vi "myRIO_BRig_RT_v0,84.vi"() -> ()   [LabVIEW 2014]
uses:
  myRIO_BRig_RT__Case_Exp_stateList.ctl
  myRIO_BRig_RT__Case_NonExp_stateList.ctl
  <vilib>/Platform/TimedLoop/XDataNode/timing_clust.ctl
  <vilib>/Platform/TimedLoop/XDataNode/nitl_modes.ctl
  <vilib>/Platform/TimedLoop/XDataNode/wakeup.ctl
  <vilib>/WebDAVClient/Advanced/SessionHandle.ctl
  <vilib>/myRIO/Common/Instrument Driver Framework/myRIO v1.0/UART/vis/myRIO v1.0 Close UART.vi
  <vilib>/FPGAPlugInAG/myRIO-1900/niLvFpga_Open_myRIO-1900.vi
  <vilib>/rvi/interface/common/dynamic/niFpgaDynamicAddResources.vi
  <vilib>/Utility/error.llb/Error Cluster From Error Code.vi
  <vilib>/rvi/errors/niLvFpgaAdjustHostInterfaceError.vi
  <vilib>/FPGAPlugInAG/Dynamic/niLvFpga_Close_Dynamic.vi
  <vilib>/myRIO/Common/Instrument Driver Framework/Utilities/vis/FPGA Ref Manager.vi
  <vilib>/myRIO/Common/Instrument Driver Framework/myRIO v1.0/myRIO v1.0 Reset FPGA.vi
  <vilib>/myRIO/Common/Instrument Driver Framework/myRIO v1.0/IRQ/vis/myRIO v1.0 IRQ Info FGV.vi
  <vilib>/myRIO/Common/Instrument Driver Framework/myRIO v1.0/IRQ/vis/myRIO v1.0 Timer IRQ Info FGV.vi
  <vilib>/myRIO/Common/Instrument Driver Framework/myRIO v1.0/IRQ/vis/myRIO v1.0 ISR Agent.vi
  <vilib>/rvi/interface/nirviOpenFPGA/nirviOpenFPGA.xnode
  myRIO_BRig_FPGA_v3,81_build.lvbitx
  myRIO_BRig_FPGA_v3,81.vi
  <vilib>/rvi/interface/nirviReadWriteControl/nirviReadWriteControl.xnode
  <vilib>/Platform/TimedLoop/XDataNode/XDataNode.xnode
  <vilib>/rvi/interface/nirviCloseFPGA/nirviCloseFPGA.xnode
  <vilib>/Platform/TimedLoop/XDataNode/XDNodeRunTimeDep.lvlib
  <vilib>/rvi/interface/Simulation/niFpgaSimulationCallBeginRW.vi
  <vilib>/myRIO/Instrument Drivers/Utilities/Utilities.lvlib
  <vilib>/WebDAVClient/NI_WebDAV.lvlib
  NiFpgaLv.dll
panel:
  in  "Laser2_baseline":bool
  in  "Laser1_baseline":bool
  in  "CueLed_baseline":bool
  out "allReward_R":bool
  out "allReward_L":bool
  in  "I_allReward":bool caption="NonSpecific Lick Direction"
  in  "Tcycle_Reward_max_R":u16=1000 caption="Max" min=5 max=5000 step=5
  in  "Tcycle_Reward_min_R":u16=1000 caption="Min" min=5 max=5000 step=5
  in  "Tcycle_Reward_step_R":u16=1000 caption="Penalty" min=1 max=10000 step=1
  in  "Tcycle_Reward_max_L":u16=1000 caption="Max" min=5 max=5000 step=5
  in  "Tcycle_Reward_min_L":u16=1000 caption="Min" min=5 max=5000 step=5
  in  "Tcycle_Reward_step_L":u16=1000 caption="Penalty" min=1 max=10000 step=1
  in  "MTrig_CueLed":bool
  out "Threshold":bool
  out "tLoop":dbl
  in  "Tcycle_Cue_LED_max":u16=1000 caption="Max" min=5 max=5000 step=5
  in  "Tcycle_Cue_LED_min":u16=1000 caption="Min" min=5 max=5000 step=5
  in  "Tcycle_CuePenalty_LED":u16=1000 caption="Penalty" min=1 max=10000 step=1
  out "power_l2":dbl
  in  "MTrig_Laser_Switch":bool
  in  "Cue1Param_AudioLed_Count_NS":u16
  in  "Cue1Param_AudioLed_Count_Switch":u16
  in  "Cue1Param_AudioLed_Probability_NS":u16
  in  "Cue1Param_CueType_NS":u16(slide) max=2 step=1 scale=0.0..2.0
  in  "Cue1Param_AudioLed_Probability_Switch":u16
  in  "Cue1Param_CueType_Switch":u16(slide) max=2 step=1 scale=0.0..2.0
  in  "CueLed_Freq":dbl=10.0
  in  "CueLed_Tpeak":dbl=2.0
  in  "Laser_power_step_l2":dbl
  in  "Laser_power_max_l2":dbl
  in  "Laser_power_min_l2":dbl
  in  "Laser_Tshutter_l2":dbl=2.0
  in  "Laser_Freq_l2":dbl=10.0
  in  "Laser_Tpeak_l2":dbl=2.0
  in  "Laser_duration_l2":u16
  in  "LC_Sel_Count_NS_l2":u16
  in  "LC_Sel_Count_Switch_l2":u16
  in  "LC_Sel_Probability_NS_l2":u16
  in  "LC_Sel_Block_NS_l2":u16(slide) max=2 step=1 scale=0.0..2.0
  in  "LC_Sel_OnOff_NS_l2":bool
  in  "LC_Sel_Probability_Switch_l2":u16
  in  "LC_Sel_Block_Switch_l2":u16(slide) max=2 step=1 scale=0.0..2.0
  in  "LC_Sel_OnOff_Switch_l2":bool
  in  "LC_Sel_Tdelay_NS_l2":u16
  in  "LC_Sel_Tdelay_Switch_l2":u16
  in  "LC_Cue1_Count_NS_l2":u16
  in  "LC_Cue1_Count_Switch_l2":u16
  in  "LC_Cue1_delayOpt_NS_l2":bool
  in  "LC_ENL1_delayOpt_NS_l2":bool
  in  "LC_ENL1_Count_NS_l2":u16
  in  "LC_ENL1_Count_Switch_l2":u16
  in  "LC_Cue1_delayOpt_Switch_l2":bool
  in  "LC_ENL1_delayOpt_Switch_l2":bool
  in  "LC_Cue1_Probability_NS_l2":u16
  in  "LC_Cue1_Block_NS_l2":u16(slide) max=2 step=1 scale=0.0..2.0
  in  "LC_Cue1_OnOff_NS_l2":bool
  in  "LC_Cue1_Probability_Switch_l2":u16
  in  "LC_Cue1_Block_Switch_l2":u16(slide) max=2 step=1 scale=0.0..2.0
  in  "LC_Cue1_OnOff_Switch_l2":bool
  in  "LC_ENL1_Probability_NS_l2":u16 max=100 step=1
  in  "LC_ENL1_Block_NS_l2":u16(slide) max=2 step=1 scale=0.0..2.0
  in  "LC_ENL1_OnOff_NS_l2":bool
  in  "LC_ENL1_Probability_Switch_l2":u16 max=100 step=1
  in  "LC_ENL1_Block_Switch_l2":u16(slide) max=2 step=1 scale=0.0..2.0
  in  "LC_Cue1_Tdelay_NS_l2":u16
  in  "LC_ENL1_Tdelay_NS_l2":u16
  in  "LC_Cue1_Tdelay_Switch_l2":u16
  in  "LC_ENL1_Tdelay_Switch_l2":u16
  in  "LC_ENL1_OnOff_Switch_l2":bool
  in  "LC_Wrong_Probability_l2":u16
  in  "LC_Wrong_Trial_l2":u16(slide) max=2 step=1 scale=0.0..2.0
  in  "LC_Wrong_Block_l2":u16(slide) max=2 step=1 scale=0.0..2.0
  in  "LC_Wrong_OnOff_l2":bool
  in  "LC_Reward_Probability_l2":u16
  in  "LC_Reward_Trial_l2":u16(slide) max=2 step=1 scale=0.0..2.0
  in  "LC_Reward_Block_l2":u16(slide) max=2 step=1 scale=0.0..2.0
  in  "LC_Reward_OnOff_l2":bool
  in  "LC_Wrong_Tdelay_l2":u16
  in  "LC_Reward_Tdelay_l2":u16
  in  "LC_Sel_Count_NS_l1":u16
  in  "LC_Sel_Count_Switch_l1":u16
  in  "LC_Sel_Probability_NS_l1":u16
  in  "LC_Sel_Block_NS_l1":u16(slide) max=2 step=1 scale=0.0..2.0
  in  "LC_Sel_OnOff_NS_l1":bool
  in  "LC_Sel_Probability_Switch_l1":u16
  in  "LC_Sel_Block_Switch_l1":u16(slide) max=2 step=1 scale=0.0..2.0
  in  "LC_Sel_OnOff_Switch_l1":bool
  in  "LC_Sel_Tdelay_NS_l1":u16
  in  "LC_Sel_Tdelay_Switch_l1":u16
  out "I_connect_TCP":bool
  in  "get_countPerMS":bool
  in  "count_warmup_R_reset":bool
  in  "count_warmup_L_reset":bool
  out "count_warmup_R":u16
  out "count_warmup_L":u16
  out "SolenoidReward":bool
  in  "SolenoidProbability_L":u16=100 caption="Reward Time [ms]" min=1 max=1000 step=1
  in  "SolenoidProbability_R":u16=100 caption="Reward Time [ms]" min=1 max=1000 step=1
  out "power_l1":dbl caption="LaserPower"
  in  "Laser_power_step_l1":dbl
  in  "Laser_power_max_l1":dbl
  in  "Recording":bool
  in  "Laser_power_min_l1":dbl
  in  "FPGA_count2ms":dbl=159.0
  in  "Laser_Tshutter_l1":dbl=2.0
  in  "Laser_Freq_l1":dbl=10.0
  in  "Laser_Tpeak_l1":dbl=2.0
  in  "Laser_duration_l1":u16
  out "error out":errorcluster
  in  "LC_Cue1_Count_NS_l1":u16
  in  "LC_Cue1_Count_Switch_l1":u16
  in  "LC_Cue1_delayOpt_NS_l1":bool
  in  "LC_ENL1_delayOpt_NS_l1":bool
  in  "LC_ENL1_Count_NS_l1":u16
  in  "LC_ENL1_Count_Switch_l1":u16
  in  "LC_Cue1_delayOpt_Switch_l1":bool
  in  "LC_ENL1_delayOpt_Switch_l1":bool
  in  "Tcycle_Cue_Audio_max":u16=1000 caption="Max" min=5 max=5000 step=5
  in  "Tcycle_Cue_Audio_min":u16=1000 caption="Min" min=5 max=5000 step=5
  in  "SendData":bool
  out "cSpout":enum16{"Left", "Right"}(ring) caption="Left or Right Spout"
  out "A4":u32 caption="LickCounter_Right"
  out "A2":u32 caption="LickCounter_Left"
  in  "LR_wrong_Event":bool
  out "SelectWrong":bool
  out "SelectReward":bool
  in  "Left(F)_or_Right(T)":bool
  in  "ignoreWrong":bool
  in  "SelectionState":bool
  in  "LR_wrong_Laser":bool
  in  "LR_reward_Laser":bool
  in  "LR_reward_Event":bool
  out "nRewards_Right":u16 caption="# Rewards Total (Right)"
  out "nRewards_Left":u16 caption="# Rewards Total (Left)"
  out "nRewards_cur":u16 caption="# Rewards in Current Block"
  out "TpB_target":u16 caption="Target Trials Per Block"
  out "cState_NonExp":T1 caption="WarmUp State"
  out "iBlock":u16 caption="Current Block"
  out "cState":T2 caption="Experimental State"
  out "iTrial":u16 caption="Current Trial"
  in  "warmupType":u8(slide) max=2 step=1 scale=0.0..2.0
  in  "TestConnection":bool
  in  "warmup":bool caption="WarmUp"
  in  "Data Set Prefix":string="Exp1_TM2"
  out "Connected To Host?":bool
  in  "Host Password":string="sabalab"
  in  "Host UserName":string="Test2"
  in  "sp_RightSpout":u16(slide)=2 max=2 step=1 scale=0.0..2.0
  in  "sp_LeftSpout":u16(slide)=2 max=2 step=1 scale=0.0..2.0
  in  "BUR_max":u16 caption="Count Reward Structure  (0 = off)"
  in  "LC_Wrong_Probability_l1":u16
  in  "LC_Wrong_Trial_l1":u16(slide) max=2 step=1 scale=0.0..2.0
  in  "LC_Wrong_Block_l1":u16(slide) max=2 step=1 scale=0.0..2.0
  in  "LC_Wrong_OnOff_l1":bool
  in  "LC_Reward_Probability_l1":u16
  in  "LC_Reward_Trial_l1":u16(slide) max=2 step=1 scale=0.0..2.0
  in  "LC_Reward_Block_l1":u16(slide) max=2 step=1 scale=0.0..2.0
  in  "LC_Reward_OnOff_l1":bool
  in  "LC_Cue1_Probability_NS_l1":u16
  in  "LC_Cue1_Block_NS_l1":u16(slide) max=2 step=1 scale=0.0..2.0
  in  "LC_Cue1_OnOff_NS_l1":bool
  in  "LC_Cue1_Probability_Switch_l1":u16
  in  "LC_Cue1_Block_Switch_l1":u16(slide) max=2 step=1 scale=0.0..2.0
  in  "LC_Cue1_OnOff_Switch_l1":bool
  in  "LC_ENL1_Probability_NS_l1":u16 max=100 step=1
  in  "LC_ENL1_Block_NS_l1":u16(slide) max=2 step=1 scale=0.0..2.0
  in  "LC_ENL1_OnOff_NS_l1":bool
  in  "LC_ENL1_Probability_Switch_l1":u16 max=100 step=1
  in  "LC_ENL1_Block_Switch_l1":u16(slide) max=2 step=1 scale=0.0..2.0
  in  "Tcycle_Timeout":u16=1000 caption="Timeout Time [ms]" min=10 max=10000 step=1
  in  "Tcycle_Wrong":u16=1000 caption="Wrong Time [ms]" min=10 max=10000 step=1
  in  "Tcycle_Selection":u16=1000 caption="Answer Time [ms]" min=1 max=10000 step=1
  in  "Tcycle_RewardPost":u16=1000 caption="Consumption Time [ms]" min=250 max=10000 step=250
  in  "TpB_Max_R":u16=4 caption="Max TrialsPerBlock" min=1 max=12 step=1
  in  "TpB_Min_R":u16=4 caption="Min TrialsPerBlock" min=1 max=12 step=1
  in  "TpB_Max_L":u16=4 caption="Max TrialsPerBlock" min=1 max=12 step=1
  in  "TpB_Min_L":u16=4 caption="Min TrialsPerBlock" min=1 max=12 step=1
  in  "BUR_min":u16 caption="Count Reward Structure\n(0 = off)"
  in  "TrialUntilReward":bool caption="Ignore Wrong Selection"
  in  "CueCycles":u16=1 caption="Cue Structure" min=1 max=1 step=1
  in  "MTrig_Laser_Tcycle":u16=10 caption="Time [ms]"
  in  "MTrig_Laser_trig":bool
  in  "MTrig_Audio_trig__R":bool caption="Trigger Audio"
  in  "MTrig_Audio_trig__L":bool caption="Trigger Audio"
  in  "RewCalib_Trig_R":bool caption="Calibrate_R"
  in  "RewCalib_Trig_L":bool caption="Calibrate_L"
  in  "MTrig_Solenoid_Tcycle__R":u16=300 caption="Time [ms]"
  in  "MTrig_Solenoid_Tcycle__L":u16=300 caption="Time [ms]"
  in  "MTrig_Solenoid_trig__R":bool caption="Solenoid"
  in  "MTrig_Solenoid_trig__L":bool caption="Solenoid"
  in  "STOP_abort":bool caption="Stop LabView\n(Stops myRio and FPGA)"
  in  "STOP_endBlock":bool caption="Stop Experiment\n@ End of Block"
  in  "STOP_endTrial":bool caption="Stop Experiment\n@ End of Trial"
  in  "START":bool caption="Start Experiment"
  in  "Tcycle_CuePenalty_Audio":u16=1000 caption="Penalty" min=1 max=10000 step=1
  in  "Audio_Amp__R":u16=100 caption="Amp"
  in  "Audio_Freq__R":u8=5 caption="Freq [kHz]" max=14 step=1
  in  "Audio_Amp__L":u16=100 caption="Amp"
  in  "Audio_Freq__L":u8=5 caption="Freq [kHz]" max=14 step=1
  in  "LC_Wrong_Tdelay_l1":u16
  in  "LC_Cue1_Tdelay_NS_l1":u16
  in  "LC_ENL1_Tdelay_NS_l1":u16
  in  "LC_Reward_Tdelay_l1":u16
  in  "LC_Cue1_Tdelay_Switch_l1":u16
  in  "LC_ENL1_Tdelay_Switch_l1":u16
  in  "LC_ENL1_OnOff_Switch_l1":bool
  in  "Tcycle_ENLPenalty":u16=100 caption="Penalty" min=10 max=10000 step=10
  in  "Tcycle_ENL_max":u16=1000 caption="Max" min=250 max=10000 step=250
  in  "Tcycle_ENL_min":u16=1000 caption="Min" min=250 max=10000 step=250
  # "Communication (Host PC)"
  # "Recording Rig"
  # "Experimental Run"
  # "Experiment Task Structure"
  # "STOP experiment at"
  # "Min            Max            Penalty"
  # "(1) = Switching\n(2) = Two Choice"
  # "Enforced\nNonLick"
  # "FPGA Count per [ms]"
  # "Cue Audio"
  # "Current State"
  # "Cue LED"
  # "Global Parameters                                                         Trial Parameters"
  # "Selection"
  # "WarmUp"
  # "Reward - Dispense Water"
  # "Left/Right        Give Reward?        Laser Power [V]"
  # "Laser1      Laser2"
  # "Left"
  # "Cue then reward (no lick)\n \nLeft                    Right"
  # "Right"
  # "Min"
  # "Max"
  # "Dispense Water Probability"
  # "Block                   Trial            Target Trials       # Rewards \n                                                            Per Block             Current"
  # "Left"
  # "WarmUp State"
  # "Trial Per Block Structure \n               Left                        Right"
  # "Lick Counter"
  # "Right"
  # "Left           Right"
  # "Reward - Consumption"
  # "Manual Control"
  # "Min"
  # "# Rewards Total\n                                                                  Left                    Right"
  # "Experimental State"
  # "Penalty - Wrong Choice"
  # "Solenoid\n \nLeft              Right"
  # "Speaker\n \nLeft                    Right"
  # "Laser 1  |  Laser 2"
  # "Max"
  # "Penalty - Choice Timeout"
  # "Time\n[ms]"
  # "Time\n[ms]"
  # "Time = Cue Min"
  # "Cue LED"
  # "Power = Min"
  # "Cue1 Control\n                                  Cue Type           LED Probability [%]      Count"
  # "Laser1 Control\n                               On/Off      Block        Probability [%]   Delay [ms]                              Count"
  # "Laser2 Control\n                               On/Off      Block        Probability [%]   Delay [ms]                              Count"
  # "Audio or LED"
  # "Cue 1"
  # "Enforced\nNonLick\n      1"
  # "Enforced\nNonLick\n      1"
  # "from end"
  # "from end"
  # "Switch\nTrial"
  # "Switch\nTrial"
  # "Switch\nTrial"
  # "from start"
  # "from start"
  # "from end"
  # "from end"
  # "NonSwitch\nTrials"
  # "NonSwitch\nTrials"
  # "NonSwitch\nTrials"
  # "from start"
  # "from start"
  # "Cue 1"
  # "Cue 1"
  # "from end"
  # "from end"
  # "Switch\nTrial"
  # "Switch\nTrial"
  # "Cue Audio Parameters"
  # "Cue LED Parameters"
  # "from start"
  # "from start"
  # "Left                  Right"
  # "Frequency\n[Hz]"
  # "Frequency\n[kHz]"
  # "from end"
  # "from end"
  # "NonSwitch\nTrials"
  # "NonSwitch\nTrials"
  # "Timing [ms]\n                    Peak Width"
  # "from start"
  # "from start"
  # "Amp\n(0 - 32,000)"
  # "Selection"
  # "Selection"
  # "from start"
  # "from start"
  # "Switch\nTrial"
  # "Switch\nTrial"
  # "Speaker\nPattern\nDuring Cue"
  # "from start"
  # "from start"
  # "NonSwitch\nTrials"
  # "NonSwitch\nTrials"
  # "Laser1 Parameters"
  # "Laser2 Parameters"
  # "Laser1 Response\n                               On/Off      Block       Trial       Probability [%]   Delay [ms]"
  # "Laser2 Response\n                               On/Off      Block       Trial       Probability [%]   Delay [ms]"
  # "Frequency\n[Hz]"
  # "Frequency\n[Hz]"
  # "Timing [ms]\n Duration     Peak Width   Shutter"
  # "Timing [ms]\n Duration     Peak Width   Shutter"
  # "Selection Reward"
  # "Selection Reward"
  # "Laser Power [V]\nMin          Max              Step"
  # "Laser Power [V]\nMin          Max              Step"
  # "Selection Wrong"
  # "Selection Wrong"
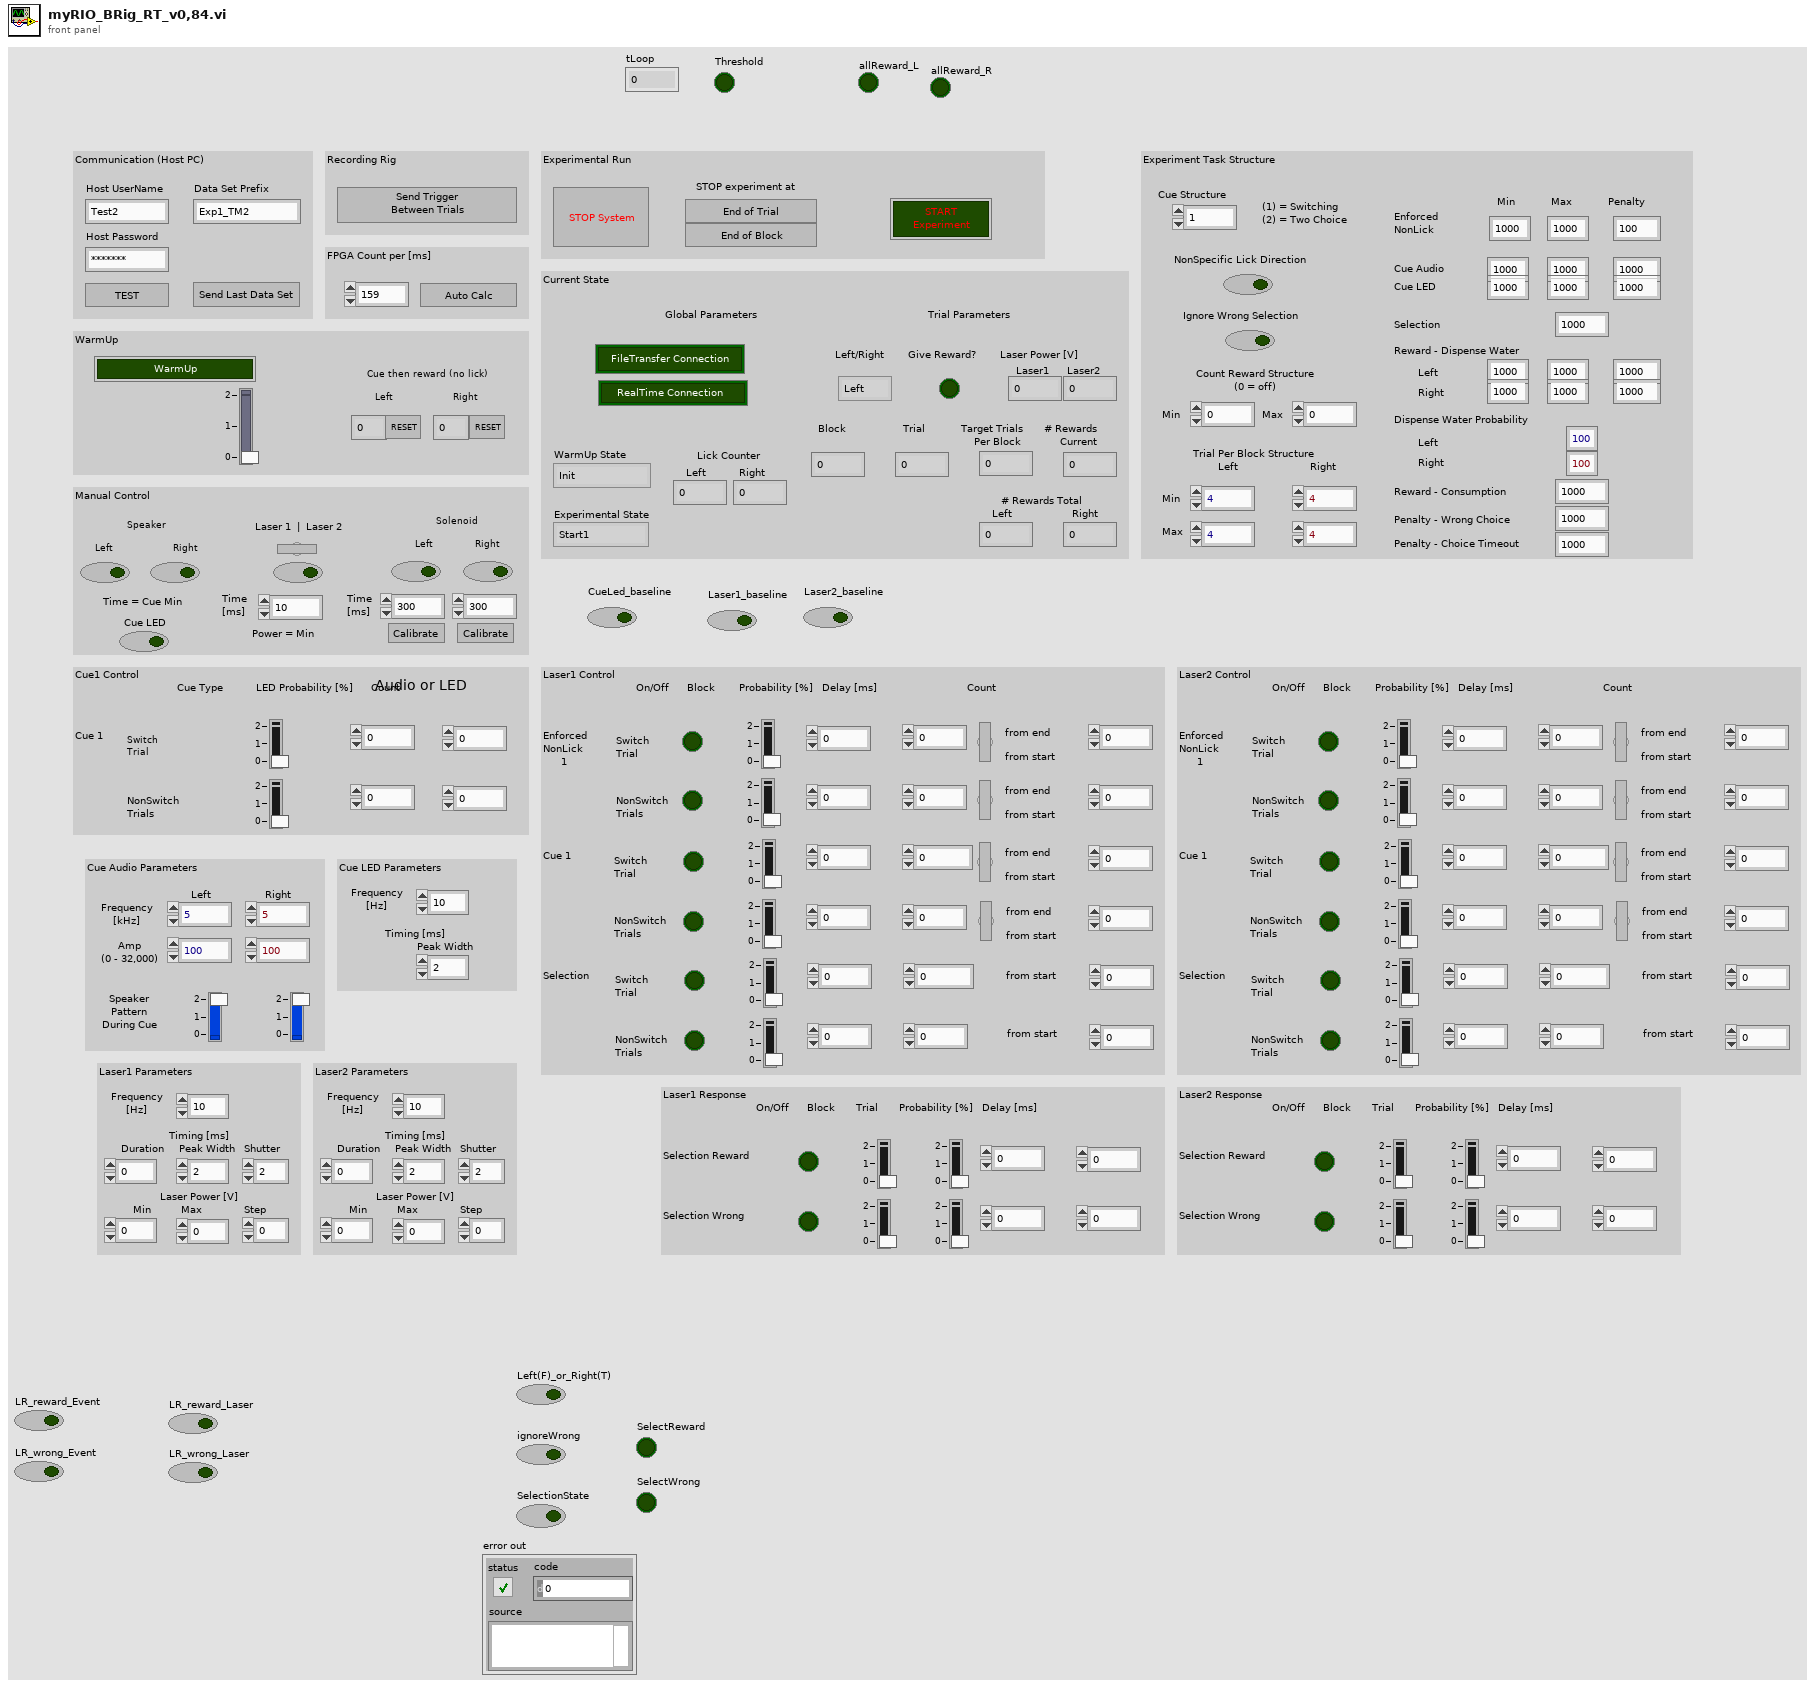
[diagram p1: front panel]
types:
  T1 = typedef "myRIO_BRig_RT__Case_NonExp_stateList.ctl" = enum16{"Init", "UploadSettings_pre", "UploadSettings_Read_dataExp", "UploadSettings_dataExp_1", "UploadSettings_dataExp_2", "UploadSettings_Read_dataLC", "UploadSettings_dataLC_1", "UploadSettings_dataLC_2", "UploadSettings_dataLC_3", "UploadSettings_dataLC_4", "UploadSettings_Read_dataMTrig", "UploadSettings_dataMTrig_1", "UploadSettings_post", "Idle_pre", "IdleEmpty", "IdleEmpty2", "IdleEmpty3", "IdleEmpty4", "Idle", "Idle_2", "Idle_3", "Idle_4", "Idle_5", "Idle_6", "Idle_post", "Cue_pre__pre", "Cue_pre", "Cue", "Cue_LED", "Cue_post", "RewardCalibration_pre", "DispenseWater_pre__pre", "DispenseWater_pre", "DispenseWater", "DispenseWater_post", "TestConnection", "SendData", "Get_FPGA_count_per_ms", "End"}
  T2 = typedef "myRIO_BRig_RT__Case_Exp_stateList.ctl" = enum16{"Start1", "Start2", "Start3", "saveSettings1", "saveSettings2", "saveSettings3", "saveSettings4", "saveSettings_LC_ENL_l1", "saveSettings_LC_ENL_l2", "saveSettings_LC_Cue_l1", "saveSettings_LC_Cue_l2", "saveSettings6_LC_l1_Other", "SaveSettings6_LC_l2_Other", "setSettings_Audio", "setSettings_Laser", "initBlock_pre", "initBlock", "initBlock2", "initBlock_post", "initTrial_pre", "initTrial", "initTrial2", "initTrial3", "initTrial4", "initTrial_LC_ENL1", "initTrial_LC_Cue1", "initTrial_LC_Cue1_2", "initTrial_LC_Sel", "initTrial_post", "ENL1_pre", "ENL1", "ENL1_post", "ENL1Penalty_pre", "ENL1Penalty", "ENL2_pre", "ENL2", "ENL2Penalty_pre", "ENL2Penalty", "Cue1_pre", "Cue1", "Cue1_post", "Cue1Penalty_pre", "Cue1Penalty", "Cue2_pre", "Cue2", "Cue2Penalty_pre", "Cue2Penalty", "Selection_pre", "Selection", "Select_post", "SelectReward_pre", "SelectReward", "SelectRewardPost_pre", "SelectRewardPost", "SelectWrong_pre", "SelectWrong", "SelectWrong_post", "SelectTimeout_pre", "SelectTimeout", "SelectTimeout_post", "endTrial_pre", "endTrial1", "endTrial2", "endTrial3", "endTrial_post", "endBlock_pre", "endBlock", "endBlock_post", "endExp", "commConnect", "commUpload_pre", "commUpload_dataBlock", "commUpload_dataCurrent", "commUpload_dataExp", "commUpload_dataLC", "commUpload_dataTrial", "commUpload_post", "saveData_pre", "saveData_dataBlock", "saveData_dataCurrent", "saveData_dataExp", "saveData_dataLC", "saveData_dataTrial", "saveData_post", "empty_endBlock1", "empty_endBlock2", "empty_endTrial1", "empty_endTrial2", "empty_endTrial3", "empty_endTrial4", "empty_endTrial5", "dummyState", "dummyState_endBlock"}
  T3 = typedef "XDNodeRunTimeDep.lvlib/timing_clust.ctl" = cluster{"Expected End [f-1]":u64, "Actual End [f-1]":u64, "Finished Late? [f-1]":bool, "Expected End [i-1]":u64, "Actual End [i-1]":u64, "Finished Late? [i-1]":bool, "Expected Start [i]":u64, "Actual Start [i]":u64, "Expected Start [f]":u64, "Actual Start [f]":u64, "Source Name":string, "Structure Name":string, "Period":i64, "Deadline":i64, "Offset":i64, "Start":i64, "Priority":i32, "Timeout":i32, "Mode":T4, "Wakeup Reason":T5, "Error":errorcluster, "Source Type":string, "Secondary Source Type":string, "Global End Time":u64, "Global Start Time":u64, "Frame Duration":u64, "Iteration Duration":u64, "Assigned CPU":i32, "I/O Scan Engine Mode":u32}
  T4 = typedef "XDNodeRunTimeDep.lvlib/nitl_modes.ctl" = enum32{"No Change", "Process missed periods, maintain original phase", "Discard missed periods, maintain original phase", "Process missed periods, ignore original phase", "Discard missed periods, ignore original phase"}
  T5 = typedef "XDNodeRunTimeDep.lvlib/wakeup.ctl" = enum32{"Normal", "Aborted", "Asynchronous wakeup", "Timing source error", "Timed loop error", "Timeout"}
  T6 = typedef "NI_WebDAV.lvlib/SessionHandle.ctl" = refnum<k1>
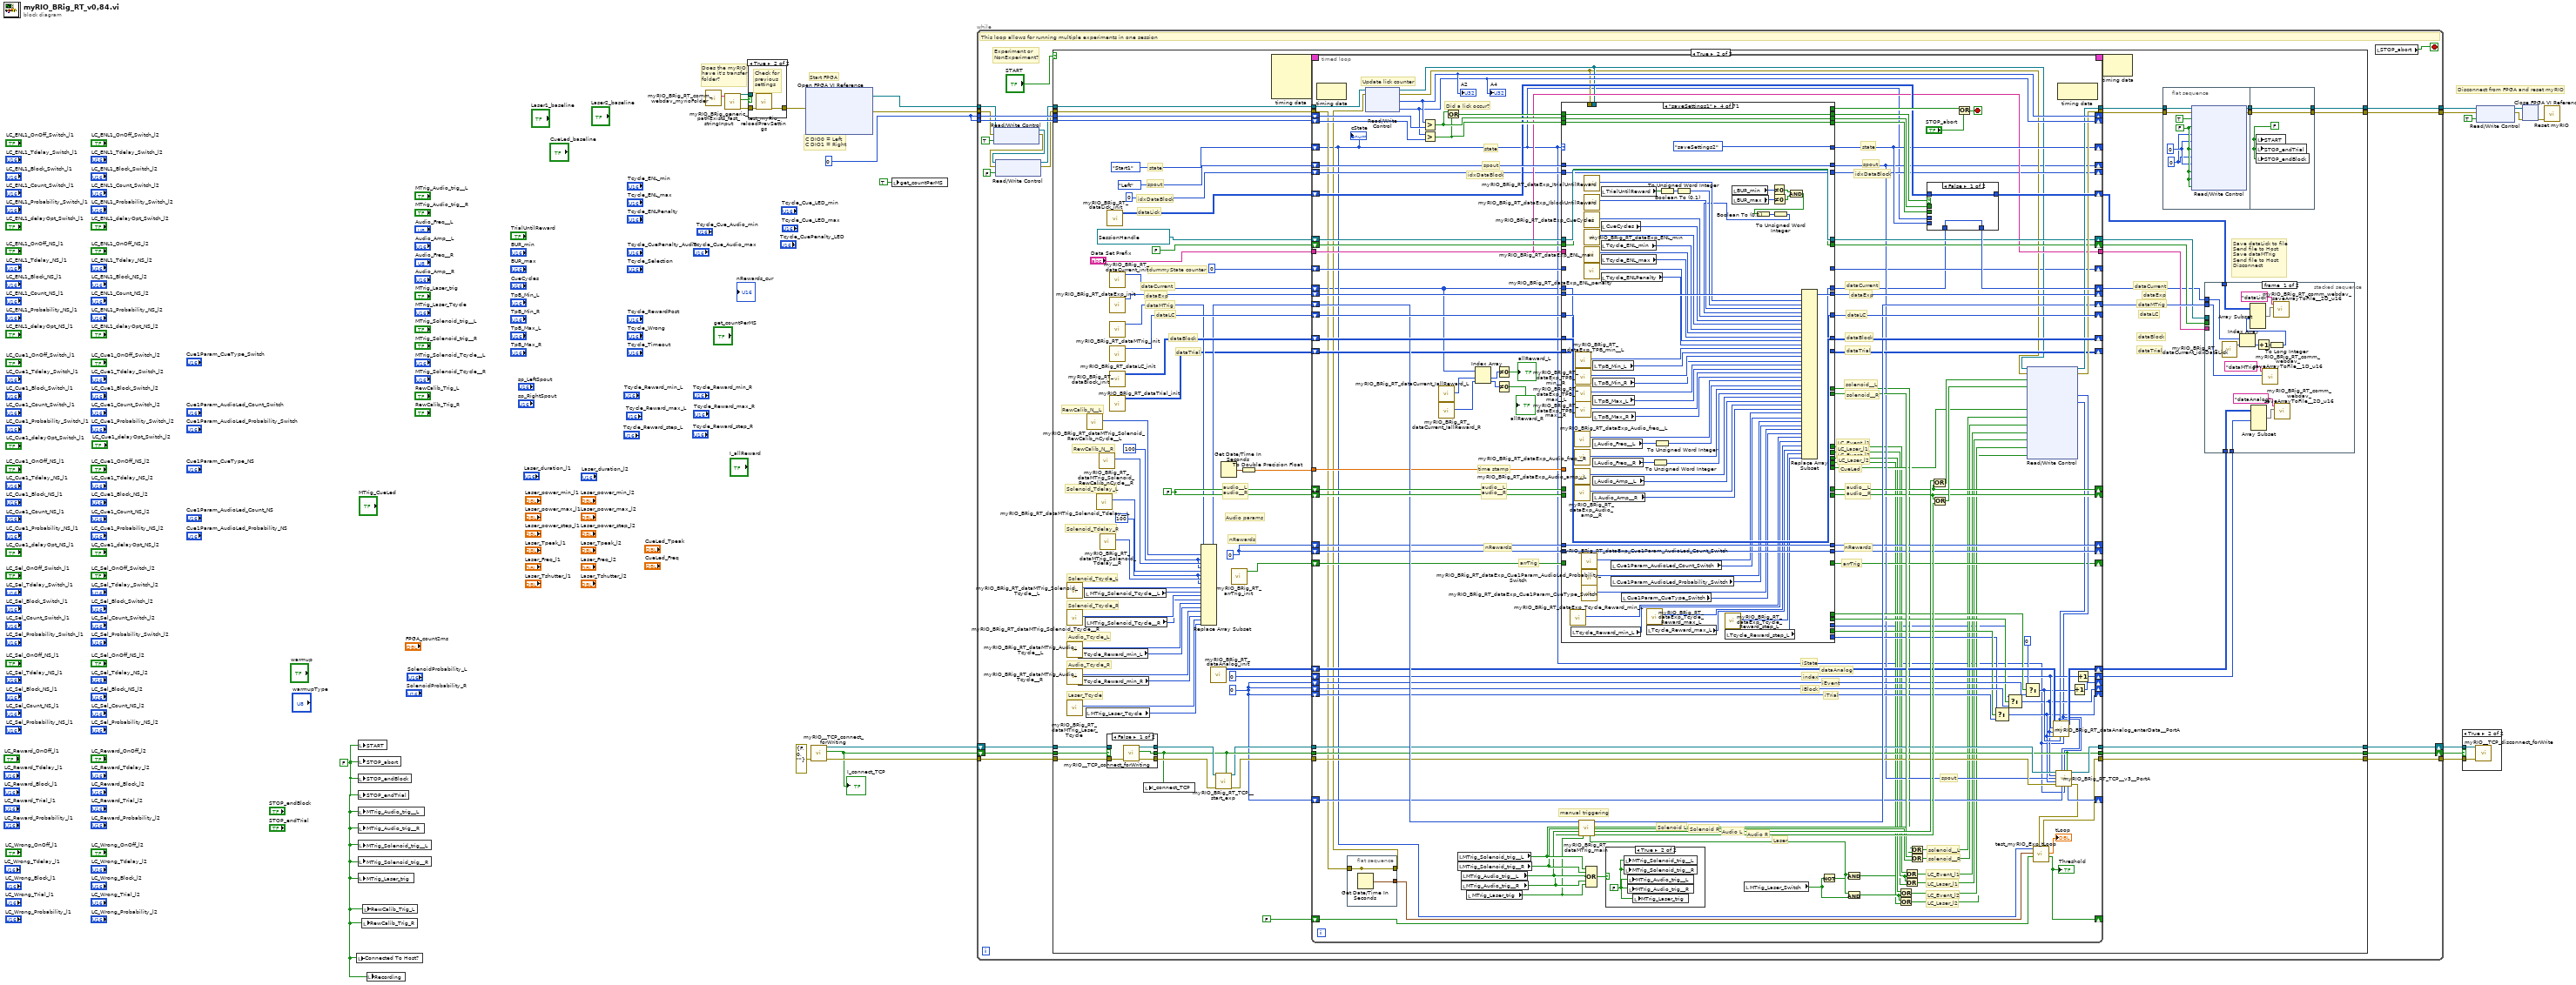
[diagram p0: block diagram]
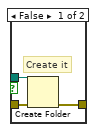
[diagram p3: hidden frame]
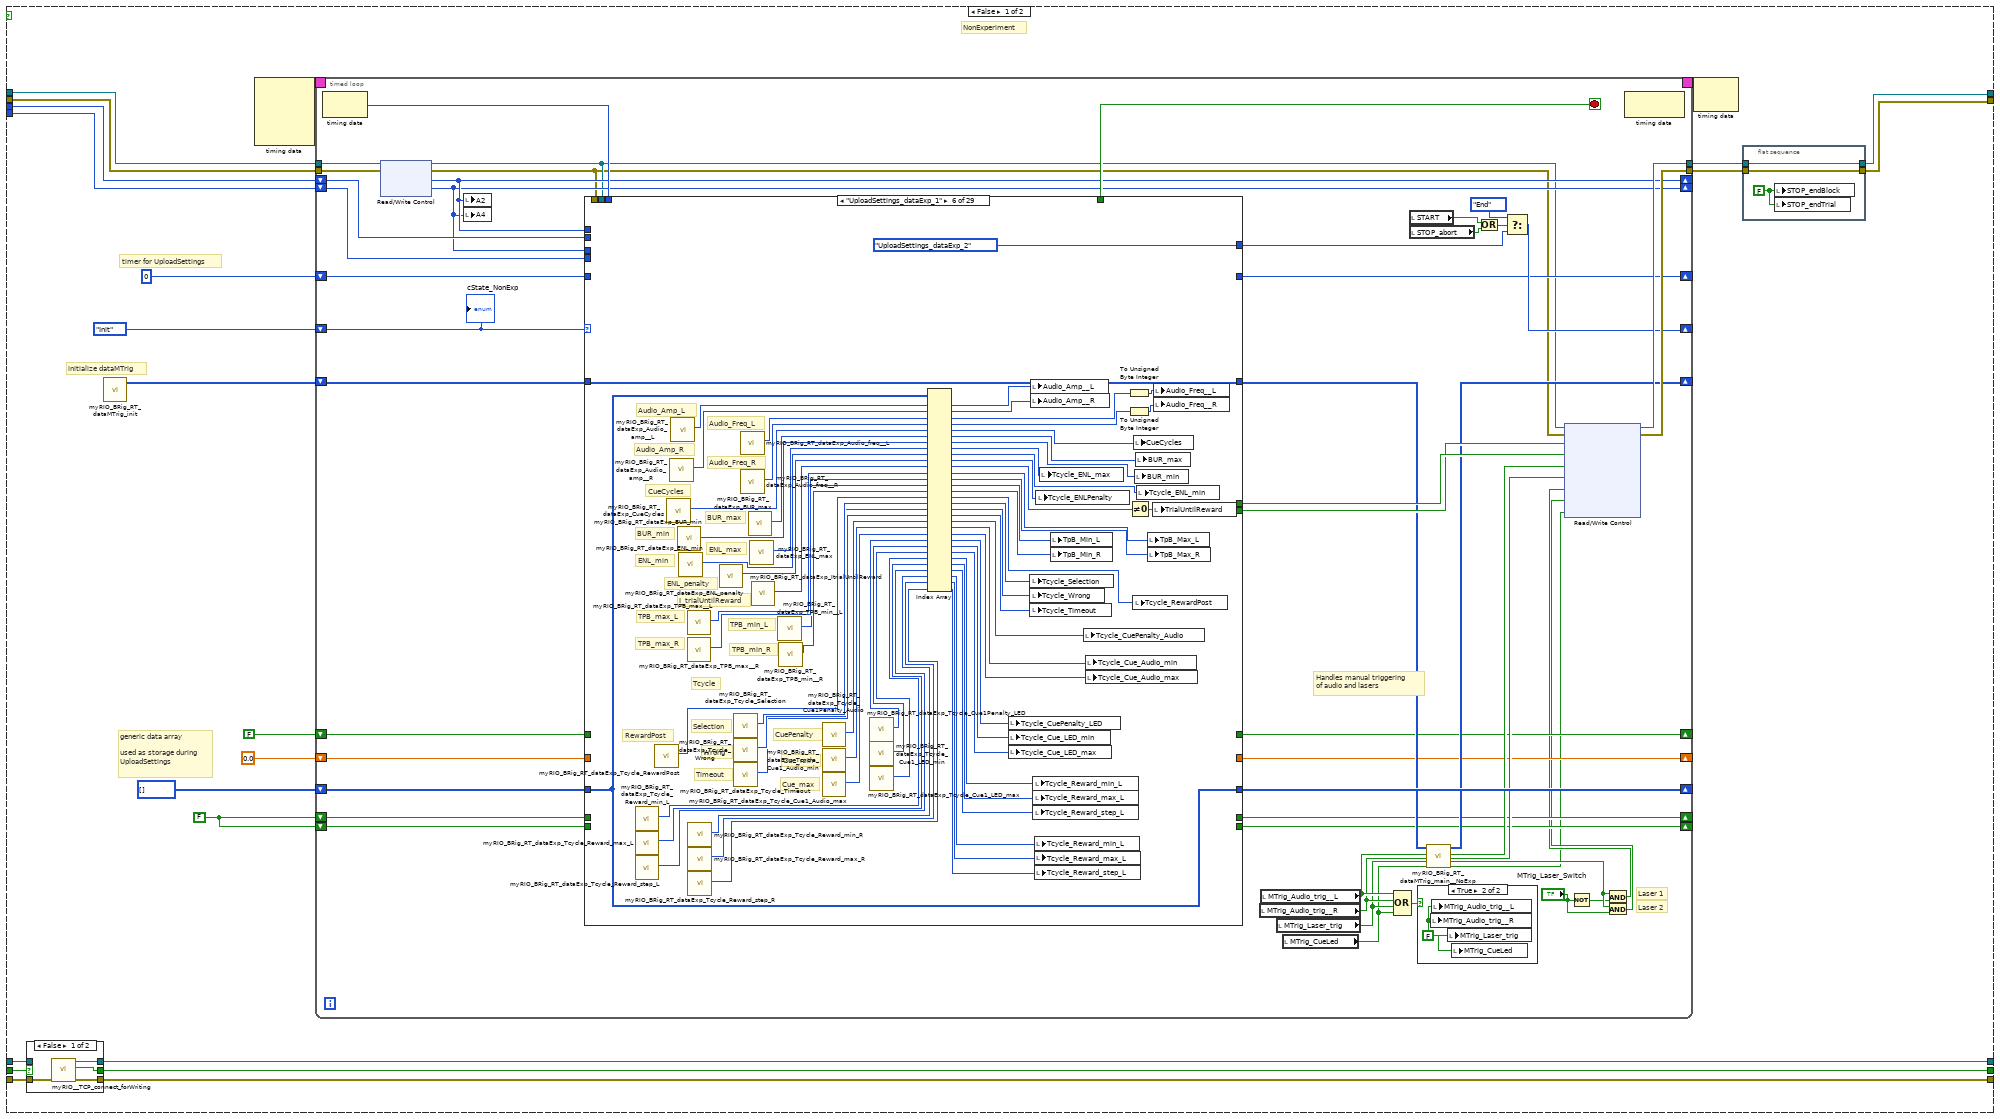
[diagram p4: hidden frame]
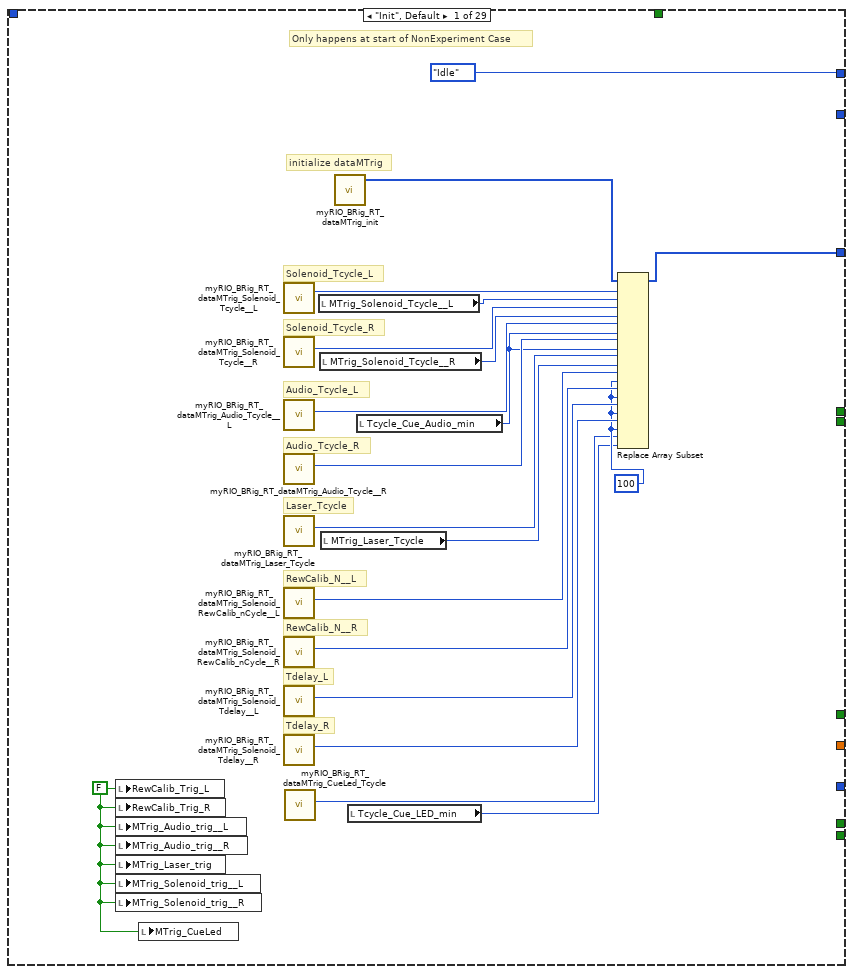
[diagram p7: hidden frame]
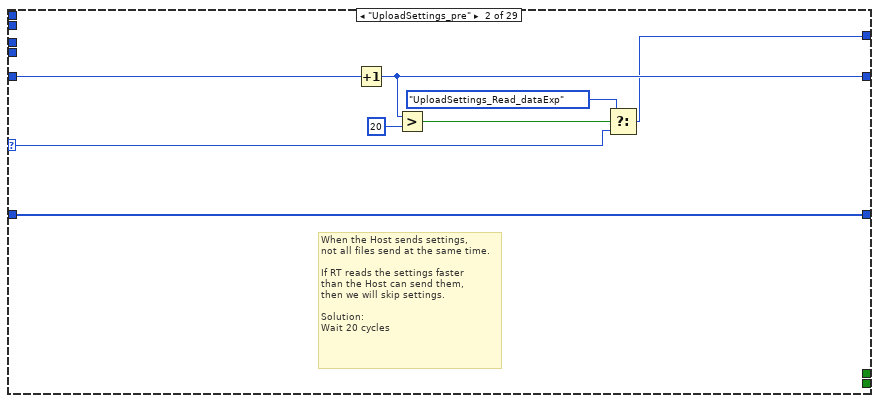
[diagram p8: hidden frame]
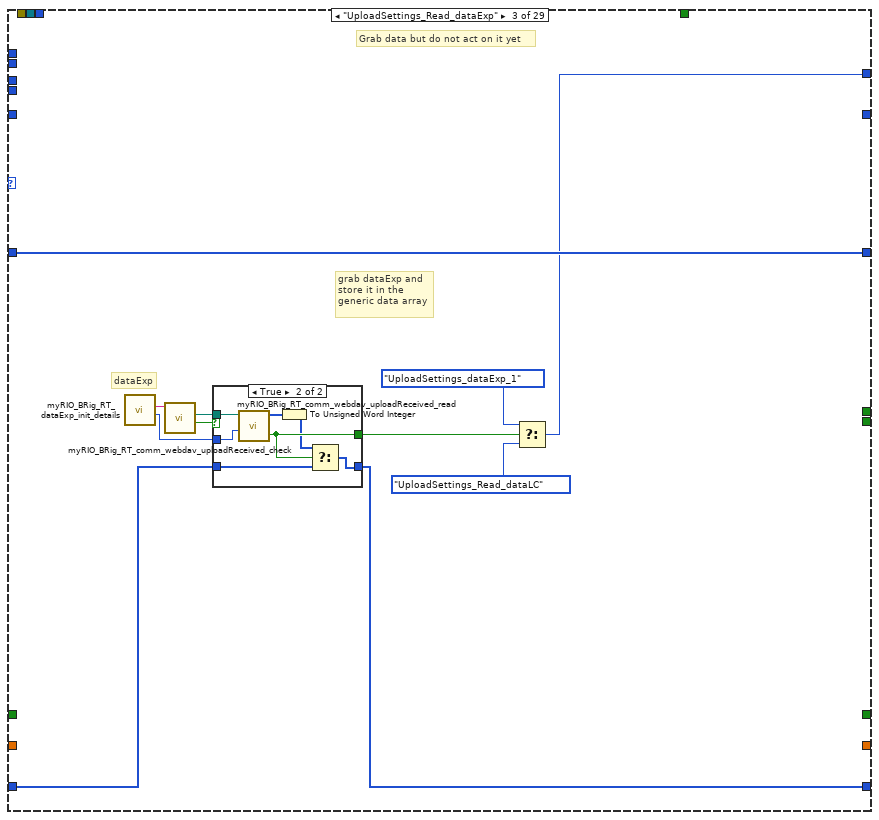
[diagram p9: hidden frame]
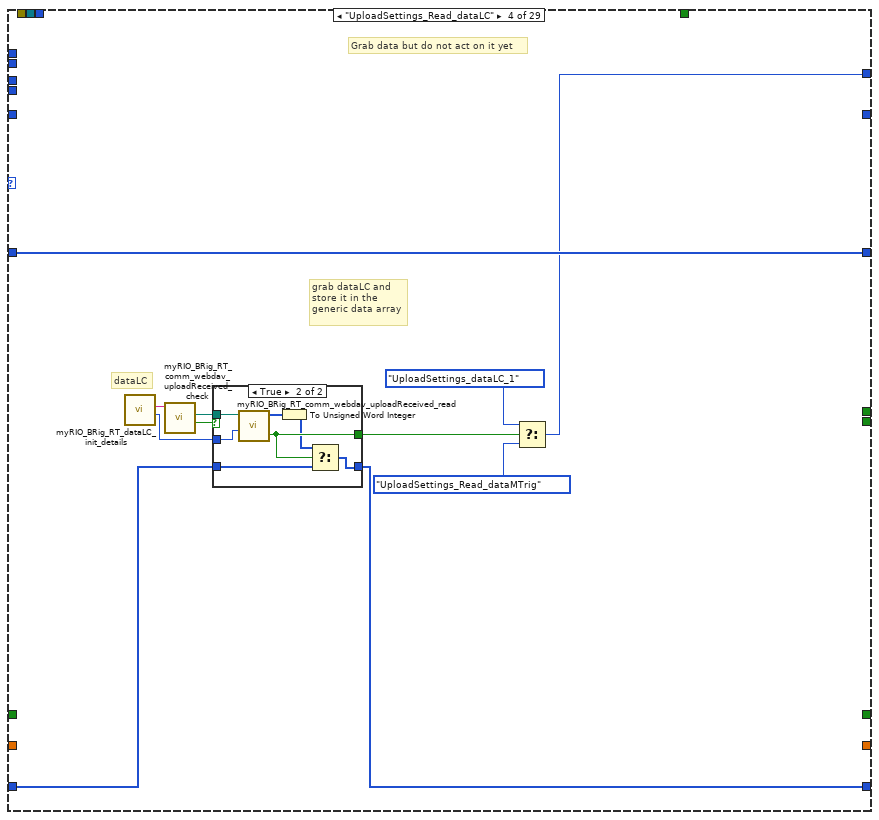
[diagram p11: hidden frame]
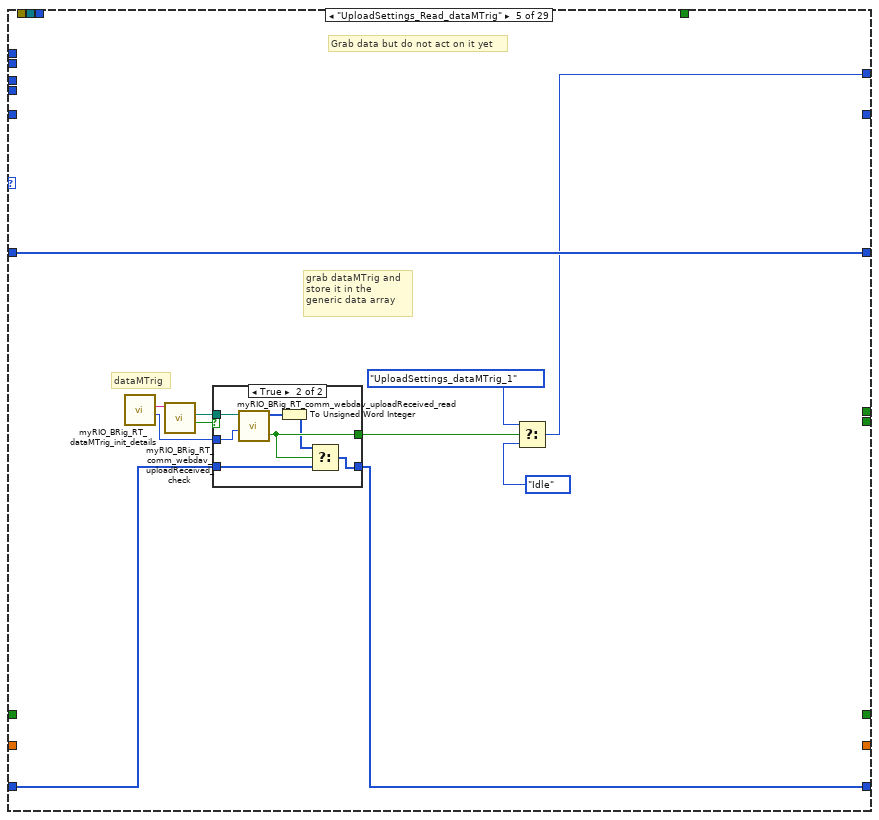
[diagram p13: hidden frame]
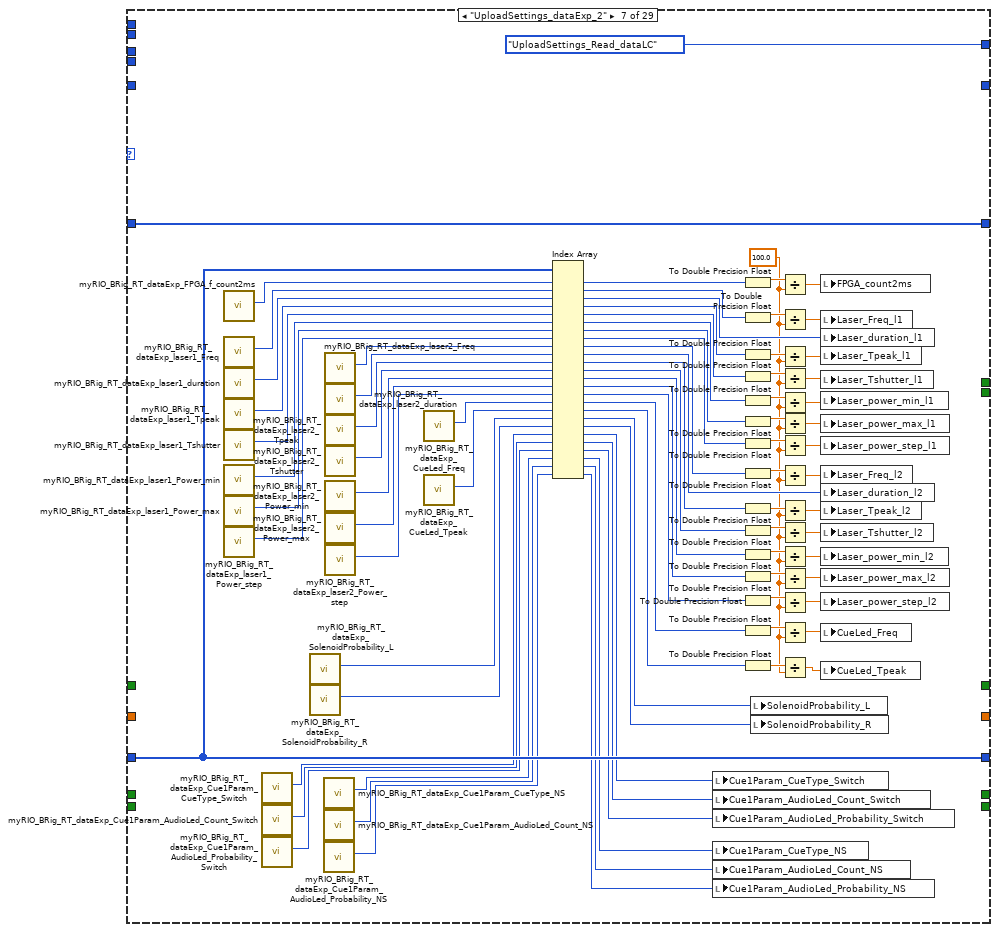
[diagram p15: hidden frame]
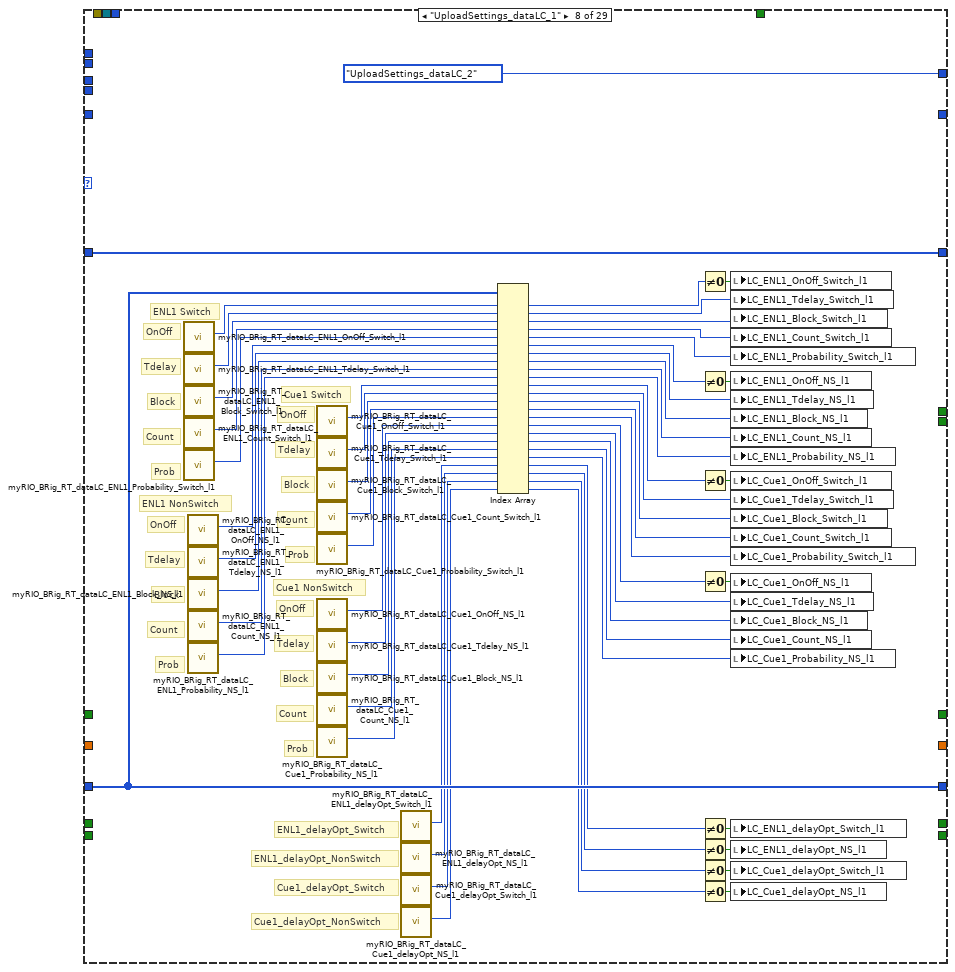
[diagram p16: hidden frame]
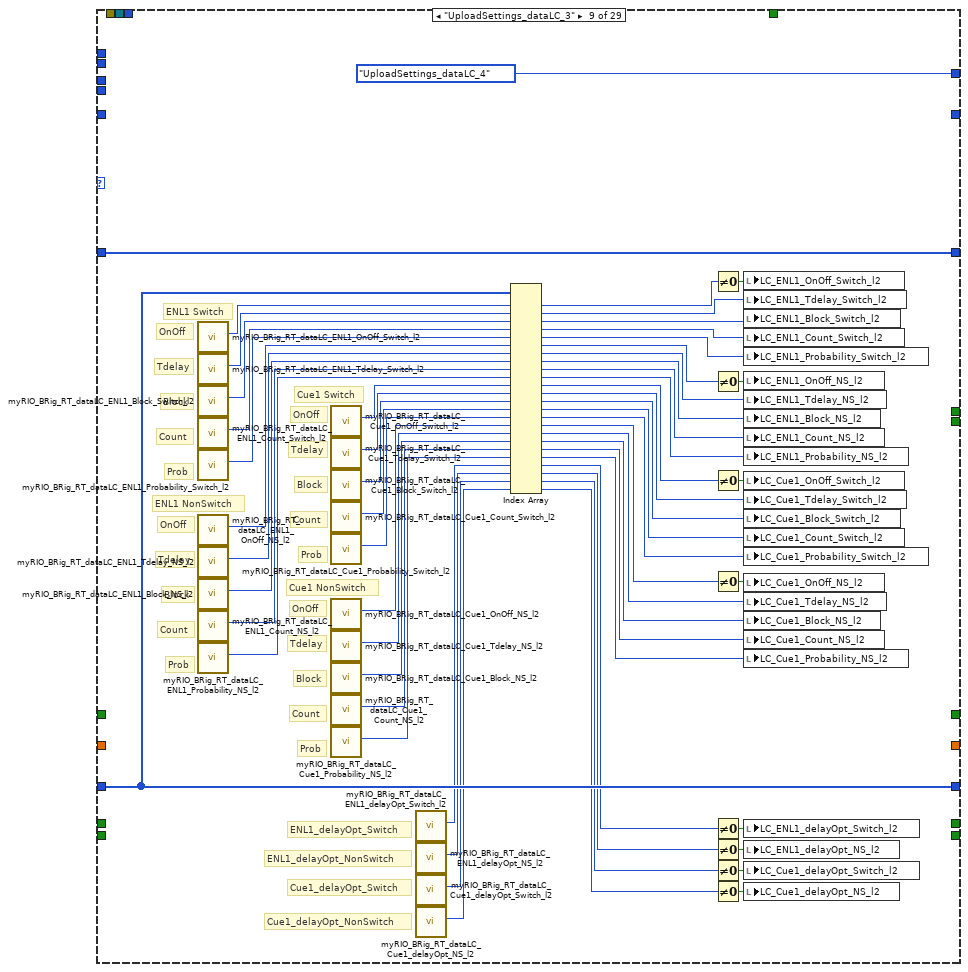
[diagram p17: hidden frame]
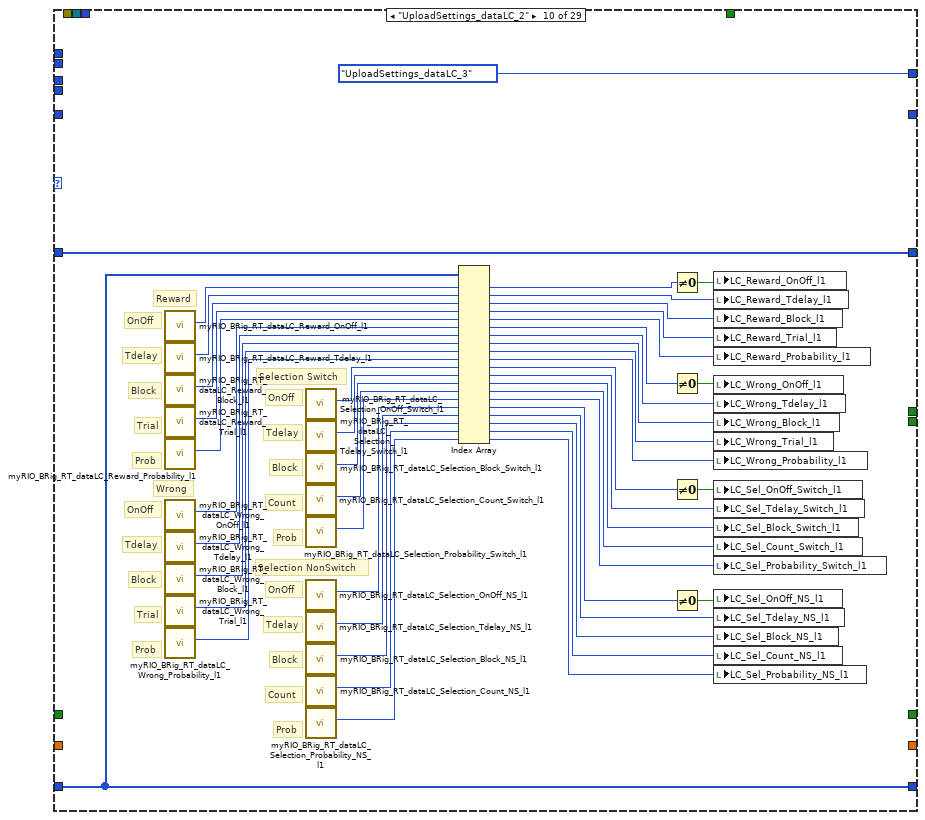
[diagram p18: hidden frame]
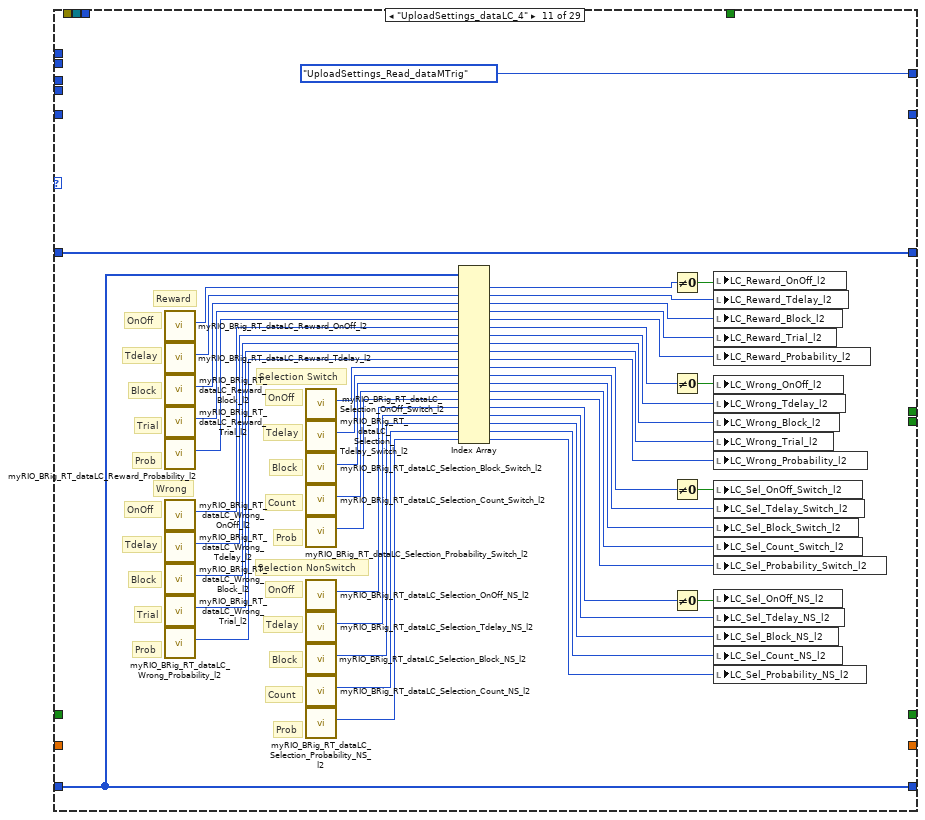
[diagram p19: hidden frame]
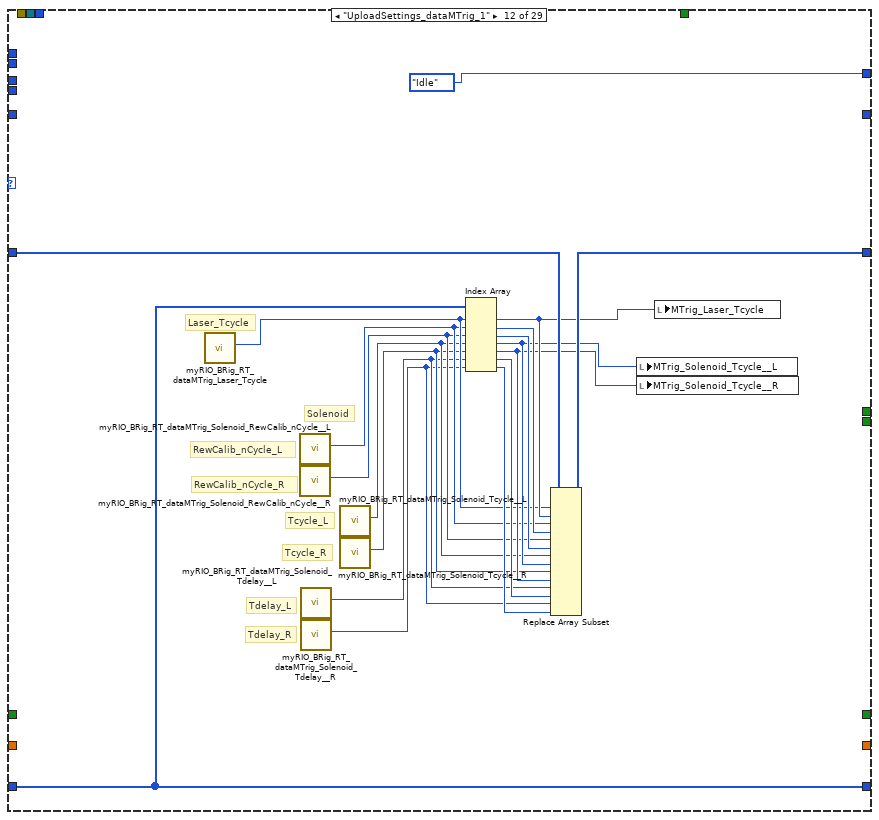
[diagram p20: hidden frame]
diagram:
  w17 = u32 0
  w1 = FALSE
  # "Does the myRIO\nhave it's transfer\nfolder?"
  # "C DIO0 = Left\nC DIO1 = Right"
  # "Start FPGA"
  # "Disconnect from FPGA and reset myRIO"
  n1 = local write "Connected To Host?"(w1) -> ()
  n2 = local write "START"(w1) -> ()
  n3 = local write "STOP_abort"(w1) -> ()
  n4 = local write "STOP_endBlock"(w1) -> ()
  n5 = local write "STOP_endTrial"(w1) -> ()
  n6 = local write "MTrig_Audio_trig__L"(w1) -> ()
  n7 = local write "MTrig_Audio_trig__R"(w1) -> ()
  n8 = local write "MTrig_Solenoid_trig__L"(w1) -> ()
  n9 = local write "MTrig_Solenoid_trig__R"(w1) -> ()
  n10 = local write "MTrig_Laser_trig"(w1) -> ()
  n11 = local write "RewCalib_Trig_R"(w1) -> ()
  n12 = local write "RewCalib_Trig_L"(w1) -> ()
  n13 = local write "Recording"(w1) -> ()
  n14 = call "myRIO_BRig_RT_comm_webdav_myrioFolder.vi"() -> ("output_myrioFolder"=w14:string)  [unwired: 11 in]
  n15 = call "myRIO_BRig_generic_pathExists_fast_stringInput.vi"("input_filePath"=w14) -> ("output_error"=w13:errorcluster, "output_Iexist"=w12:bool, "output_filePath"=w11:path)  [unwired: 8 in]
  n16 = case shown="True" w12 {
    tunnel: w11 -> [w26 _]
    tunnel: w13 -> [w25 w28]
    tunnel: [w24 w27] -> w9
    frame False {
      # "Create it"
      n17 = Create Folder(path (use dialog)=w26, error in=w25) -> (error out=w24:errorcluster)  [unwired: 1 in, 2 out]
    }
    frame True {
      # "Check for\nprevious\nsettings"
      n18 = call "test_myRio_reloadPrevSettings.vi"("input_error"=w28) -> ("output_error"=w27:errorcluster)  [unwired: 10 in]
    }
  }
  n19 = xnode "Open FPGA VI Reference"("error in"=w9) -> ("FPGA VI Reference Out"=w19:refnum<k20>, "error out"=w18:errorcluster)  [unwired: 1 in]
  n20 = call "myRIO__TCP_connect_forWriting.vi"("input_error"=errorcluster {"status"=FALSE, "code"=0, "source"=""}) -> ("output_error"=w7:errorcluster, "output_connected"=w6:bool, "output_hTCP"=w10:refnum<k5>)  [unwired: 8 in]
  "I_connect_TCP" <- w6
  n21 = local write "get_countPerMS"(TRUE ("get_countPerMS")) -> ()
  n22 = while {
    tunnel: w19 -> [w38]
    tunnel: w18 -> [w43]
    tunnel: w17 -> [w46]
    tunnel: w17 -> [w45]
    tunnel: [w36] -> w16
    tunnel: [w35] -> w15
    shift-right: [w32] -> w5
    shift-left: w6 -> [w33]
    tunnel: w7 -> [w31]
    shift-right: [w30] -> w4
    shift-left: w10 -> [w34]
    tunnel: [w29] -> w3
    stop <- w44 stop-if-true
    # "Experiment or\nNonExperiment?"
    # "This loop allows for running multiple experiments in one session"
    n23 = xnode "Read/Write Control"("FPGA VI Reference In"=w38, "error in"=w43, "Counts_Reset"=TRUE) -> ("FPGA VI Reference Out"=w40:refnum<k20>, "error out"=w41:errorcluster)
    n24 = xnode "Read/Write Control"("FPGA VI Reference In"=w40, "error in"=w41, "Counts_Reset"=FALSE) -> ("FPGA VI Reference Out"=w37:refnum<k20>, "error out"=w39:errorcluster)
    n25 = case shown="True" "START" {
      tunnel: w46 -> [w67 w1525]
      tunnel: w45 -> [w66 w1524]
      tunnel: w39 -> [w64 w1459]
      tunnel: w37 -> [w65 w1460]
      tunnel: [w62 w1521] -> w36
      tunnel: [w60 w1516] -> w35
      tunnel: w34 -> [w53 w1470]
      tunnel: [w51 w1474] -> w30
      tunnel: w33 -> [w52 w1472]
      tunnel: [w50 w1473] -> w32
      tunnel: w31 -> [w54 w1471]
      tunnel: [w49 w1469] -> w29
      frame False {
        w57 = FALSE
        # "generic data array\n\nused as storage during\nUploadSettings"
        # "timer for UploadSettings"
        # "initialize dataMTrig"
        # "NonExperiment"
        n26 = case shown="False" w52 {
          selector: w52 -> [_ w76]
          tunnel: w54 -> [w73 w78]
          tunnel: [w74 w78] -> w49
          tunnel: w53 -> [_ w77]
          tunnel: [w75 w77] -> w51
          tunnel: [w72 w76] -> w50
          frame False {
            n27 = call "myRIO__TCP_connect_forWriting.vi"("input_error"=w73) -> ("output_error"=w74:errorcluster, "output_connected"=w72:bool, "output_hTCP"=w75:refnum<k5>)  [unwired: 8 in]
          }
          frame True {
          }
        }
        n28 = call "myRIO_BRig_RT_dataMTrig_init.vi"() -> ("output_dataMTrig"=w68:u16[])  [unwired: 5 in]
        n29 = node-c288() -> (w71:T3)  [unwired: 4 in]
        n30 = timed-loop {
          timing: w71 -> [_]
          timing-out: [_] -> w70
          shift-right: [w117] -> _
          shift-left: w68 -> [w129]
          shift-right: [w111] -> _
          shift-left: myRIO_BRig_RT__Case_NonExp_stateList."Init" ("Enum") -> [w123]
          shift-right: [w105] -> _
          shift-left: w67 -> [w106]
          shift-right: [w103] -> _
          shift-left: w66 -> [w104]
          tunnel: [w125] -> w63
          tunnel: [w124] -> w61
          tunnel: w64 -> [w127]
          tunnel: w65 -> [w126]
          shift-right: [w122] -> _
          shift-left: u16[] [] ("output_data") -> [w121]
          shift-right: [w107] -> _
          shift-left: u16 0 ("Audio_Amp__L") -> [w108]
          shift-right: [w100] -> _
          shift-left: w57 -> [w102]
          shift-right: [w99] -> _
          shift-left: w57 -> [w101]
          shift-right: [w95] -> _
          shift-left: FALSE -> [w96]
          shift-right: [w93] -> _
          shift-left: 0.0 -> [w94]
          stop <- w130 stop-if-true
          # "Laser 2"
          # "Laser 1"
          # "Handles manual triggering\nof audio and lasers"
          n31 = node-c288() -> (w128:i64)  [unwired: 1 in]
          n32 = xnode "Read/Write Control"("FPGA VI Reference In"=w126, "error in"=w127) -> ("FPGA VI Reference Out"=w98:refnum<k20>, "error out"=w97:errorcluster, "A2_LickL"=w105:u32, "A4_LickR"=w103:u32)
          n33 = local write "A2"(w105) -> ()
          n34 = local write "A4"(w103) -> ()
          n35 = case shown="\"UploadSettings_dataExp_1\"" w123 {
            selector: w123 -> [_ w155 _ _ _ _ _ _ _ _ _ _ _ _ _ _ _ _ _ w1074 w1133 _ _ w1338 _ _ _ w1411 w1452]
            tunnel: [myRIO_BRig_RT__Case_NonExp_stateList."Idle" ("Enum") w153 w160 w179 w198 myRIO_BRig_RT__Case_NonExp_stateList."UploadSettings_dataExp_2" ("Enum") myRIO_BRig_RT__Case_NonExp_stateList."UploadSettings_Read_dataLC" ("Enum") myRIO_BRig_RT__Case_NonExp_stateList."UploadSettings_dataLC_2" ("Enum") myRIO_BRig_RT__Case_NonExp_stateList."UploadSettings_dataLC_4" ("Enum") myRIO_BRig_RT__Case_NonExp_stateList."UploadSettings_dataLC_3" ("f") myRIO_BRig_RT__Case_NonExp_stateList."UploadSettings_Read_dataMTrig" ("f") myRIO_BRig_RT__Case_NonExp_stateList."Idle" ("Enum") w621 w657 myRIO_BRig_RT__Case_NonExp_stateList."Idle_5" ("Enum") w730 w848 w1010 w1041 w1069 w1128 myRIO_BRig_RT__Case_NonExp_stateList."DispenseWater_pre" ("Enum") w1284 w1336 w1358 myRIO_BRig_RT__Case_NonExp_stateList."Idle" ("Enum") myRIO_BRig_RT__Case_NonExp_stateList."Idle" ("Enum") w1410 w1452] -> w112
            tunnel: [w143 w152 w170 w189 w208 w284 w368 w421 w480 w533 w580 w596 w625 w672 w716 w735 w853 w1008 w1048 w1075 w1134 w1195 w1321 w1343 w1369 w1403 w1408 w1420 w1450] -> w118
            tunnel: [_ _ _ _ _ _ _ _ _ _ _ _ _ _ _ _ _ _ _ _ _ _ _ _ _ _ _ _ TRUE] -> w130
            tunnel: w129 -> [_ w152 w170 w189 w208 w284 w368 w421 w480 w533 w580 w597 w624 w672 w716 w736 w854 w1008 w1049 w1076 w1135 w1181 w1317 w1344 w1370 w1403 w1408 w1420 w1450]
            tunnel: w128 -> [_ _ _ _ _ _ _ _ _ _ _ _ _ _ _ _ _ _ _ _ _ _ _ w1348 _ _ _ _ _]
            tunnel: [_ _ w161 w180 w199 w249 w366 w422 w481 w529 w576 w581 _ _ _ _ _ _ w1037 _ w1122 _ _ _ _ _ _ _ _] -> w122
            tunnel: w121 -> [_ _ w162 w181 w200 w249 w366 w422 w481 w529 w576 w581 _ _ _ _ _ _ _ _ w1123 _ _ _ _ _ _ _ _]
            tunnel: [_ _ _ _ _ _ _ _ _ _ _ _ _ _ _ _ _ _ _ _ _ _ _ w1345 _ _ _ _ _] -> w120
            tunnel: [_ _ _ _ _ _ _ _ _ _ _ _ _ _ _ _ _ _ _ _ _ _ _ w1327 _ _ _ _ _] -> w119
            tunnel: w108 -> [_ w159 _ _ _ _ _ _ _ _ _ _ _ _ _ _ _ _ _ _ _ _ _ _ _ _ _ _ _]
            tunnel: [_ w158 _ _ _ _ _ _ _ _ _ _ _ _ _ _ _ _ _ _ _ _ _ _ _ _ _ _ _] -> w107
            tunnel: w106 -> [_ _ _ _ _ _ _ _ _ _ _ _ _ _ _ _ _ _ _ w1080 w1139 _ _ _ _ _ _ _ _]
            tunnel: w105 -> [_ _ _ _ _ _ _ _ _ _ _ _ _ _ _ _ _ _ _ w1081 w1140 _ _ _ _ _ _ _ _]
            tunnel: w104 -> [_ _ _ _ _ _ _ _ _ _ _ _ _ _ _ _ _ _ _ w1078 w1137 _ _ _ _ _ _ _ _]
            tunnel: w103 -> [_ _ _ _ _ _ _ _ _ _ _ _ _ _ _ _ _ _ _ w1079 w1138 _ _ _ _ _ _ _ _]
            tunnel: w102 -> [_ _ _ _ _ _ _ _ _ _ _ _ _ _ _ _ _ _ _ w1066 w1125 _ _ _ _ _ _ _ _]
            tunnel: w101 -> [_ _ _ _ _ _ _ _ _ _ _ _ _ _ _ _ _ _ _ w1065 w1124 _ _ _ _ _ _ _ _]
            tunnel: [_ _ _ _ _ _ _ _ _ _ _ _ _ _ _ _ _ _ w1039 w1066 w1125 _ _ _ _ _ _ _ _] -> w100
            tunnel: [_ _ _ _ _ _ _ _ _ _ _ _ _ _ _ _ _ _ w1038 w1065 w1124 _ _ _ _ _ _ _ _] -> w99
            tunnel: w98 -> [_ _ _ _ _ _ _ _ _ _ _ _ w614 w630 w718 _ _ _ _ _ w1121 _ _ _ _ _ _ w1415 _]
            tunnel: w97 -> [_ _ _ _ _ _ _ _ _ _ _ _ w613 w631 w717 _ _ _ _ _ w1120 _ _ _ _ _ _ w1414 _]
            tunnel: w96 -> [_ _ _ _ _ _ _ _ _ _ _ _ _ _ _ _ _ _ _ _ _ _ _ _ _ _ _ w1419 _]
            tunnel: [_ _ _ _ _ _ _ _ _ _ _ _ _ _ _ _ _ _ _ _ _ _ _ _ _ _ _ TRUE _] -> w95
            tunnel: w94 -> [_ _ _ _ _ _ _ _ _ _ _ _ _ _ _ _ _ _ _ _ _ _ _ _ _ _ _ w1417 _]
            tunnel: [_ _ _ _ _ _ _ _ _ _ _ _ _ _ _ _ _ _ _ _ _ _ _ _ _ _ _ w1416 _] -> w93
            frame "Init", Default {
              w134 = FALSE ("RewCalib_Trig_L")
              w135 = u16 100 ("new element/subarray")
              # "Only happens at start of NonExperiment Case"
              # "Tdelay_R"
              # "Tdelay_L"
              # "RewCalib_N__R"
              # "RewCalib_N__L"
              # "Solenoid_Tcycle_R"
              # "Solenoid_Tcycle_L"
              # "Laser_Tcycle"
              # "Audio_Tcycle_R"
              # "Audio_Tcycle_L"
              # "initialize dataMTrig"
              n36 = local write "RewCalib_Trig_L"(w134) -> ()
              n37 = local write "RewCalib_Trig_R"(w134) -> ()
              n38 = local write "MTrig_Audio_trig__L"(w134) -> ()
              n39 = local write "MTrig_Audio_trig__R"(w134) -> ()
              n40 = local write "MTrig_Laser_trig"(w134) -> ()
              n41 = local write "MTrig_Solenoid_trig__L"(w134) -> ()
              n42 = local write "MTrig_Solenoid_trig__R"(w134) -> ()
              n43 = local write "MTrig_CueLed"(w134) -> ()
              n44 = call "myRIO_BRig_RT_dataMTrig_Solenoid_Tcycle__L.vi"() -> ("output_Solenoid_Tcycle__L"=w145:i32)  [unwired: 11 in]
              n45 = call "myRIO_BRig_RT_dataMTrig_Solenoid_Tcycle__R.vi"() -> ("output_Solenoid_Tcycle__R"=w146:i32)  [unwired: 11 in]
              n46 = call "myRIO_BRig_RT_dataMTrig_Audio_Tcycle__L.vi"() -> ("output_Audio_Tcycle__L"=w147:i32)  [unwired: 11 in]
              n47 = call "myRIO_BRig_RT_dataMTrig_Audio_Tcycle__R.vi"() -> ("output_Audio_Tcycle__R"=w148:i32)  [unwired: 11 in]
              n48 = call "myRIO_BRig_RT_dataMTrig_Laser_Tcycle.vi"() -> ("output_Laser_Tcycle"=w149:i32)  [unwired: 11 in]
              n49 = call "myRIO_BRig_RT_dataMTrig_Solenoid_RewCalib_nCycle__L.vi"() -> ("output_Solenoid_RewCalib_nCycle__L"=w141:i32)  [unwired: 11 in]
              n50 = call "myRIO_BRig_RT_dataMTrig_Solenoid_RewCalib_nCycle__R.vi"() -> ("output_Solenoid_RewCalib_nCycle__R"=w140:i32)  [unwired: 11 in]
              n51 = call "myRIO_BRig_RT_dataMTrig_Solenoid_Tdelay__L.vi"() -> ("output_Solenoid_Tdelay__L"=w139:i32)  [unwired: 11 in]
              n52 = call "myRIO_BRig_RT_dataMTrig_Solenoid_Tdelay__R.vi"() -> ("output_Solenoid_Tdelay__R"=w138:i32)  [unwired: 11 in]
              n53 = call "myRIO_BRig_RT_dataMTrig_CueLed_Tcycle.vi"() -> ("output_CueLed_Tcycle"=w133:i32)  [unwired: 11 in]
              n54 = local read "MTrig_Solenoid_Tcycle__L"() -> (w150:u16)
              n55 = local read "MTrig_Solenoid_Tcycle__R"() -> (w151:u16)
              n56 = local read "MTrig_Laser_Tcycle"() -> (w136:u16)
              n57 = call "myRIO_BRig_RT_dataMTrig_init.vi"() -> ("output_dataMTrig"=w144:u16[])  [unwired: 5 in]
              n58 = local read "Tcycle_Cue_LED_min"() -> (w132:u16)
              n59 = local read "Tcycle_Cue_Audio_min"() -> (w137:u16)
              n60 = Replace Array Subset(array=w144, new element #1=w150, index #1=w145, new element #2=w151, index #2=w146, new element #3=w137, index #3=w147, new element #4=w137, index #4=w148, new element #5=w136, index #5=w149, new element #6=w135, index #6=w141, new element #7=w135, index #7=w140, new element #8=w135, index #8=w139, new element #9=w135, index #9=w138, new element #10=w132, index #10=w133) -> (w143:u16[])
            }
            frame "UploadSettings_pre" {
              # "When the Host sends settings,\nnot all files send at the same time.\n\nIf RT reads the settings faster\nthan the Host can send them,\nthen we will skip settings.\n\nSolution:\nWait 20 cycles"
              n61 = Increment(x=w159) -> (x+1=w158:u16)
              n62 = Greater?(x=w158, y=u16 20) -> (0:w156:bool)
              n63 = Select(t=myRIO_BRig_RT__Case_NonExp_stateList."UploadSettings_Read_dataExp", s=w156, f=w155) -> (s? t:f=w153:T1)
            }
            frame "UploadSettings_Read_dataExp" {
              # "Grab data but do not act on it yet"
              # "grab dataExp and\nstore it in the\ngeneric data array"
              # "dataExp"
              n64 = call "myRIO_BRig_RT_dataExp_init_details.vi"() -> ("output_dataSize"=w166:i32, "output_dataName"=w169:string)  [unwired: 10 in]
              n65 = call "myRIO_BRig_RT_comm_webdav_uploadReceived_check.vi"("input_dataName"=w169) -> ("output_Iexist"=w168:bool, "output_dataPath"=w167:path)  [unwired: 9 in]
              n66 = case shown="True" w168 {
                tunnel: w167 -> [_ w178]
                tunnel: w166 -> [_ w177]
                tunnel: [_ w176] -> w165
                tunnel: w162 -> [w171 w175]
                tunnel: [w171 w172] -> w161
                frame False {
                }
                frame True {
                  n67 = call "myRIO_BRig_RT_comm_webdav_uploadReceived_read.vi"("input_dataSize"=w177, "input_filePath"=w178) -> ("output_Ivalid"=w176:bool, "output_data"=w174:i64[])  [unwired: 8 in]
                  n68 = To Unsigned Word Integer(number=w174) -> (unsigned 16bit integer=w173:u16[])
                  n69 = Select(t=w173, s=w176, f=w175) -> (s? t:f=w172:u16[])
                }
              }
              n70 = Select(t=myRIO_BRig_RT__Case_NonExp_stateList."UploadSettings_dataExp_1", s=w165, f=myRIO_BRig_RT__Case_NonExp_stateList."UploadSettings_Read_dataLC" ("t")) -> (s? t:f=w160:T1)
            }
            frame "UploadSettings_Read_dataLC" {
              # "Grab data but do not act on it yet"
              # "grab dataLC and\nstore it in the\ngeneric data array"
              # "dataLC"
              n71 = call "myRIO_BRig_RT_dataLC_init_details.vi"() -> ("output_dataSize"=w185:i32, "output_dataName"=w188:string)  [unwired: 10 in]
              n72 = call "myRIO_BRig_RT_comm_webdav_uploadReceived_check.vi"("input_dataName"=w188) -> ("output_Iexist"=w187:bool, "output_dataPath"=w186:path)  [unwired: 9 in]
              n73 = case shown="True" w187 {
                tunnel: w186 -> [_ w197]
                tunnel: w185 -> [_ w196]
                tunnel: [_ w195] -> w184
                tunnel: w181 -> [w190 w194]
                tunnel: [w190 w191] -> w180
                frame False {
                }
                frame True {
                  n74 = call "myRIO_BRig_RT_comm_webdav_uploadReceived_read.vi"("input_dataSize"=w196, "input_filePath"=w197) -> ("output_Ivalid"=w195:bool, "output_data"=w193:i64[])  [unwired: 8 in]
                  n75 = To Unsigned Word Integer(number=w193) -> (unsigned 16bit integer=w192:u16[])
                  n76 = Select(t=w192, s=w195, f=w194) -> (s? t:f=w191:u16[])
                }
              }
              n77 = Select(t=myRIO_BRig_RT__Case_NonExp_stateList."UploadSettings_dataLC_1", s=w184, f=myRIO_BRig_RT__Case_NonExp_stateList."UploadSettings_Read_dataMTrig" ("t")) -> (s? t:f=w179:T1)
            }
            frame "UploadSettings_Read_dataMTrig" {
              # "Grab data but do not act on it yet"
              # "grab dataMTrig and\nstore it in the\ngeneric data array"
              # "dataMTrig"
              n78 = call "myRIO_BRig_RT_dataMTrig_init_details.vi"() -> ("output_dataSize"=w204:i32, "output_dataName"=w207:string)  [unwired: 10 in]
              n79 = call "myRIO_BRig_RT_comm_webdav_uploadReceived_check.vi"("input_dataName"=w207) -> ("output_Iexist"=w206:bool, "output_dataPath"=w205:path)  [unwired: 9 in]
              n80 = case shown="True" w206 {
                tunnel: w205 -> [_ w216]
                tunnel: w204 -> [_ w215]
                tunnel: [_ w214] -> w203
                tunnel: w200 -> [w209 w213]
                tunnel: [w209 w210] -> w199
                frame False {
                }
                frame True {
                  n81 = call "myRIO_BRig_RT_comm_webdav_uploadReceived_read.vi"("input_dataSize"=w215, "input_filePath"=w216) -> ("output_Ivalid"=w214:bool, "output_data"=w212:i64[])  [unwired: 8 in]
                  n82 = To Unsigned Word Integer(number=w212) -> (unsigned 16bit integer=w211:u16[])
                  n83 = Select(t=w211, s=w214, f=w213) -> (s? t:f=w210:u16[])
                }
              }
              n84 = Select(t=myRIO_BRig_RT__Case_NonExp_stateList."UploadSettings_dataMTrig_1", s=w203, f=myRIO_BRig_RT__Case_NonExp_stateList."Idle" ("t")) -> (s? t:f=w198:T1)
            }
            frame "UploadSettings_dataExp_1" {
              # "Cue_max"
              # "Cue_min"
              # "CuePenalty"
              # "Timeout"
              # "Wrong"
              # "Selection"
              # "RewardPost"
              # "Tcycle"
              # "TPB_min_R"
              # "TPB_min_L"
              # "TPB_max_R"
              # "TPB_max_L"
              # "I_trialUntilReward"
              # "ENL_penalty"
              # "ENL_min"
              # "ENL_max"
              # "BUR_max"
              # "BUR_min"
              # "CueCycles"
              # "Audio_Freq_R"
              # "Audio_Freq_L"
              # "Audio_Amp_R"
              # "Audio_Amp_L"
              n85 = call "myRIO_BRig_RT_dataExp_Tcycle_Reward_min_L.vi"() -> ("output_Tcycle_Reward_min_L"=w228:i32)  [unwired: 11 in]
              n86 = call "myRIO_BRig_RT_dataExp_Tcycle_Reward_max_L.vi"() -> ("output_Tcycle_Reward_max_L"=w227:i32)  [unwired: 11 in]
              n87 = call "myRIO_BRig_RT_dataExp_Tcycle_Reward_step_L.vi"() -> ("output_Tcycle_Reward_step_L"=w226:i32)  [unwired: 11 in]
              n88 = call "myRIO_BRig_RT_dataExp_Tcycle_RewardPost.vi"() -> ("output_Tcycle_RewardPost"=w248:i32)  [unwired: 11 in]
              n89 = call "myRIO_BRig_RT_dataExp_CueCycles.vi"() -> ("output_CueCycles"=w276:i32)  [unwired: 11 in]
              n90 = call "myRIO_BRig_RT_dataExp_Audio_amp__R.vi"() -> ("output_Audio_amp__R"=w280:i32)  [unwired: 11 in]
              n91 = call "myRIO_BRig_RT_dataExp_Audio_amp__L.vi"() -> ("output_Audio_amp__L"=w282:i32)  [unwired: 11 in]
              n92 = call "myRIO_BRig_RT_dataExp_BUR_min.vi"() -> ("output_BUR_min"=w273:i32)  [unwired: 11 in]
              n93 = call "myRIO_BRig_RT_dataExp_ENL_min.vi"() -> ("output_ENL_min"=w269:i32)  [unwired: 11 in]
              n94 = call "myRIO_BRig_RT_dataExp_TPB_max__L.vi"() -> ("output_TPB_max__L"=w261:i32)  [unwired: 11 in]
              n95 = call "myRIO_BRig_RT_dataExp_TPB_max__R.vi"() -> ("output_TPB_max__R"=w260:i32)  [unwired: 11 in]
              n96 = call "myRIO_BRig_RT_dataExp_Tcycle_Reward_min_R.vi"() -> ("output_Tcycle_Reward_min_R"=w225:i32)  [unwired: 11 in]
              n97 = call "myRIO_BRig_RT_dataExp_Tcycle_Reward_max_R.vi"() -> ("output_Tcycle_Reward_max_R"=w224:i32)  [unwired: 11 in]
              n98 = call "myRIO_BRig_RT_dataExp_Tcycle_Reward_step_R.vi"() -> ("output_Tcycle_Reward_step_R"=w223:i32)  [unwired: 11 in]
              n99 = call "myRIO_BRig_RT_dataExp_ENL_penalty.vi"() -> ("output_ENL_penalty"=w268:i32)  [unwired: 11 in]
              n100 = call "myRIO_BRig_RT_dataExp_Tcycle_Selection.vi"() -> ("output_Tcycle_Selection"=w247:i32)  [unwired: 11 in]
              n101 = call "myRIO_BRig_RT_dataExp_Tcycle_Wrong.vi"() -> ("output_Tcycle_Wrong"=w246:i32)  [unwired: 11 in]
              n102 = call "myRIO_BRig_RT_dataExp_Tcycle_Timeout.vi"() -> ("output_Tcycle_Timeout"=w242:i32)  [unwired: 11 in]
              n103 = call "myRIO_BRig_RT_dataExp_Audio_freq__L.vi"() -> ("output_Audio_freq__L"=w278:i32)  [unwired: 11 in]
              n104 = call "myRIO_BRig_RT_dataExp_Audio_freq__R.vi"() -> ("output_Audio_freq__R"=w277:i32)  [unwired: 11 in]
              n105 = call "myRIO_BRig_RT_dataExp_BUR_max.vi"() -> ("output_BUR_max"=w274:i32)  [unwired: 11 in]
              n106 = call "myRIO_BRig_RT_dataExp_ENL_max.vi"() -> ("output_ENL_max"=w270:i32)  [unwired: 11 in]
              n107 = call "myRIO_BRig_RT_dataExp_ItrialUntilReward.vi"() -> ("output_I_trialUntilReward"=w264:i32)  [unwired: 11 in]
              n108 = call "myRIO_BRig_RT_dataExp_TPB_min__L.vi"() -> ("output_TPB_min__L"=w259:i32)  [unwired: 11 in]
              n109 = call "myRIO_BRig_RT_dataExp_TPB_min__R.vi"() -> ("output_TPB_min__R"=w258:i32)  [unwired: 11 in]
              n110 = call "myRIO_BRig_RT_dataExp_Tcycle_Cue1Penalty_Audio.vi"() -> ("output_Tcycle_Cue1Penalty_Audio"=w240:i32)  [unwired: 11 in]
              n111 = call "myRIO_BRig_RT_dataExp_Tcycle_Cue1_Audio_min.vi"() -> ("output_Tcycle_Cue1_Audio_min"=w238:i32)  [unwired: 11 in]
              n112 = call "myRIO_BRig_RT_dataExp_Tcycle_Cue1_Audio_max.vi"() -> ("output_Tcycle_Cue1_Audio_max"=w236:i32)  [unwired: 11 in]
              n113 = call "myRIO_BRig_RT_dataExp_Tcycle_Cue1Penalty_LED.vi"() -> ("output_Tcycle_Cue1Penalty_LED"=w234:i32)  [unwired: 11 in]
              n114 = call "myRIO_BRig_RT_dataExp_Tcycle_Cue1_LED_min.vi"() -> ("output_Tcycle_Cue1_LED_min"=w233:i32)  [unwired: 11 in]
              n115 = call "myRIO_BRig_RT_dataExp_Tcycle_Cue1_LED_max.vi"() -> ("output_Tcycle_Cue1_LED_max"=w232:i32)  [unwired: 11 in]
              n116 = Index Array(array=w249, index #1=w282, index #2=w280, index #3=w278, index #4=w277, index #5=w276, index #6=w274, index #7=w273, index #8=w270, index #9=w269, index #10=w268, index #11=w264, index #12=w261, index #13=w260, index #14=w259, index #15=w258, index #16=w248, index #17=w247, index #18=w246, index #19=w242, index #20=w240, index #21=w238, index #22=w236, index #23=w234, index #24=w233, index #25=w232, index #26=w228, index #27=w227, index #28=w226, index #29=w225, index #30=w224, index #31=w223) -> (element #1=w281:u16, element #2=w279:u16, element #3=w252:u16, element #4=w251:u16, element #5=w275:u16, element #6=w272:u16, element #7=w271:u16, element #8=w267:u16, element #9=w266:u16, element #10=w265:u16, element #11=w262:u16, element #12=w257:u16, element #13=w256:u16, element #14=w255:u16, element #15=w254:u16, element #16=w245:u16, element #17=w244:u16, element #18=w243:u16, element #19=w241:u16, element #20=w239:u16, element #21=w237:u16, element #22=w235:u16, element #23=w231:u16, element #24=w230:u16, element #25=w229:u16, element #26=w222:u16, element #27=w221:u16, element #28=w220:u16, element #29=w219:u16, element #30=w218:u16, element #31=w217:u16)
              n117 = local write "Tcycle_CuePenalty_LED"(w231) -> ()
              n118 = local write "Tcycle_Cue_LED_min"(w230) -> ()
              n119 = local write "Tcycle_Cue_LED_max"(w229) -> ()
              n120 = local write "Tcycle_Selection"(w244) -> ()
              n121 = local write "Tcycle_Wrong"(w243) -> ()
              n122 = local write "Tcycle_Timeout"(w241) -> ()
              n123 = local write "Audio_Amp__L"(w281) -> ()
              n124 = local write "Audio_Amp__R"(w279) -> ()
              n125 = local write "Tcycle_Reward_min_L"(w222) -> ()
              n126 = local write "Tcycle_Reward_max_L"(w221) -> ()
              n127 = local write "Tcycle_Reward_step_L"(w220) -> ()
              n128 = local write "Tcycle_Reward_min_L"(w219) -> ()
              n129 = local write "Tcycle_Reward_max_L"(w218) -> ()
              n130 = local write "Tcycle_Reward_step_L"(w217) -> ()
              n131 = local write "Tcycle_ENLPenalty"(w265) -> ()
              n132 = local write "Tcycle_ENL_max"(w267) -> ()
              n133 = local write "TpB_Min_L"(w255) -> ()
              n134 = local write "TpB_Min_R"(w254) -> ()
              n135 = local write "Tcycle_CuePenalty_Audio"(w239) -> ()
              n136 = local write "Tcycle_Cue_Audio_min"(w237) -> ()
              n137 = local write "Tcycle_Cue_Audio_max"(w235) -> ()
              n138 = To Unsigned Byte Integer(number=w252) -> (unsigned 8bit integer=w253:u8)
              n139 = To Unsigned Byte Integer(number=w251) -> (unsigned 8bit integer=w250:u8)
              n140 = Not Equal To 0?(x=w262) -> (x != 0?=w263:bool)
              n141 = local write "Tcycle_RewardPost"(w245) -> ()
              n142 = local write "CueCycles"(w275) -> ()
              n143 = local write "BUR_min"(w271) -> ()
              n144 = local write "BUR_max"(w272) -> ()
              n145 = local write "Tcycle_ENL_min"(w266) -> ()
              n146 = local write "TpB_Max_L"(w257) -> ()
              n147 = local write "TpB_Max_R"(w256) -> ()
              n148 = local write "TrialUntilReward"(w263) -> ()
              n149 = local write "Audio_Freq__L"(w253) -> ()
              n150 = local write "Audio_Freq__R"(w250) -> ()
            }
            frame "UploadSettings_dataExp_2" {
              w304 = 100.0 ("y")
              n151 = call "myRIO_BRig_RT_dataExp_FPGA_f_count2ms.vi"() -> ("output_FPGA_f_count2ms"=w365:i32)  [unwired: 11 in]
              n152 = call "myRIO_BRig_RT_dataExp_laser1_Freq.vi"() -> ("output_laser1_Freq"=w353:i32)  [unwired: 11 in]
              n153 = call "myRIO_BRig_RT_dataExp_laser1_duration.vi"() -> ("output_laser1_duration"=w352:i32)  [unwired: 11 in]
              n154 = call "myRIO_BRig_RT_dataExp_laser1_Tpeak.vi"() -> ("output_laser1_Tpeak"=w351:i32)  [unwired: 11 in]
              n155 = call "myRIO_BRig_RT_dataExp_laser1_Tshutter.vi"() -> ("output_laser1_Tshutter"=w350:i32)  [unwired: 11 in]
              n156 = call "myRIO_BRig_RT_dataExp_laser1_Power_min.vi"() -> ("output_laser1_Power_min"=w349:i32)  [unwired: 11 in]
              n157 = call "myRIO_BRig_RT_dataExp_laser1_Power_max.vi"() -> ("output_laser1_Power_max"=w348:i32)  [unwired: 11 in]
              n158 = call "myRIO_BRig_RT_dataExp_laser1_Power_step.vi"() -> ("output_laser1_Power_step"=w347:i32)  [unwired: 11 in]
              n159 = call "myRIO_BRig_RT_dataExp_Cue1Param_CueType_Switch.vi"() -> ("output_Cue1Param_CueType_Switch"=w298:i32)  [unwired: 11 in]
              n160 = call "myRIO_BRig_RT_dataExp_Cue1Param_AudioLed_Count_Switch.vi"() -> ("output_Cue1Param_AudioLed_Count_Switch"=w297:i32)  [unwired: 11 in]
              n161 = call "myRIO_BRig_RT_dataExp_Cue1Param_AudioLed_Probability_Switch.vi"() -> ("output_Cue1Param_AudioLed_Probability_Switch"=w296:i32)  [unwired: 11 in]
              n162 = call "myRIO_BRig_RT_dataExp_SolenoidProbability_L.vi"() -> ("output_SolenoidProbability_L"=w300:i32)  [unwired: 11 in]
              n163 = call "myRIO_BRig_RT_dataExp_SolenoidProbability_R.vi"() -> ("output_SolenoidProbability_R"=w299:i32)  [unwired: 11 in]
              n164 = call "myRIO_BRig_RT_dataExp_Cue1Param_CueType_NS.vi"() -> ("output_Cue1Param_CueType_NS"=w295:i32)  [unwired: 11 in]
              n165 = call "myRIO_BRig_RT_dataExp_Cue1Param_AudioLed_Count_NS.vi"() -> ("output_Cue1Param_AudioLed_Count_NS"=w294:i32)  [unwired: 11 in]
              n166 = call "myRIO_BRig_RT_dataExp_Cue1Param_AudioLed_Probability_NS.vi"() -> ("output_Cue1Param_AudioLed_Probability_NS"=w293:i32)  [unwired: 11 in]
              n167 = call "myRIO_BRig_RT_dataExp_laser2_Freq.vi"() -> ("output_laser2_Freq"=w346:i32)  [unwired: 11 in]
              n168 = call "myRIO_BRig_RT_dataExp_laser2_duration.vi"() -> ("output_laser2_duration"=w345:i32)  [unwired: 11 in]
              n169 = call "myRIO_BRig_RT_dataExp_laser2_Tpeak.vi"() -> ("output_laser2_Tpeak"=w344:i32)  [unwired: 11 in]
              n170 = call "myRIO_BRig_RT_dataExp_laser2_Tshutter.vi"() -> ("output_laser2_Tshutter"=w343:i32)  [unwired: 11 in]
              n171 = call "myRIO_BRig_RT_dataExp_laser2_Power_min.vi"() -> ("output_laser2_Power_min"=w342:i32)  [unwired: 11 in]
              n172 = call "myRIO_BRig_RT_dataExp_laser2_Power_max.vi"() -> ("output_laser2_Power_max"=w341:i32)  [unwired: 11 in]
              n173 = call "myRIO_BRig_RT_dataExp_laser2_Power_step.vi"() -> ("output_laser2_Power_step"=w340:i32)  [unwired: 11 in]
              n174 = call "myRIO_BRig_RT_dataExp_CueLed_Freq.vi"() -> ("output_CueLed_Freq"=w309:i32)  [unwired: 11 in]
              n175 = call "myRIO_BRig_RT_dataExp_CueLed_Tpeak.vi"() -> ("output_CueLed_Tpeak"=w302:i32)  [unwired: 11 in]
              n176 = Index Array(array=w366, index #1=w365, index #2=w353, index #3=w352, index #4=w351, index #5=w350, index #6=w349, index #7=w348, index #8=w347, index #9=w346, index #10=w345, index #11=w344, index #12=w343, index #13=w342, index #14=w341, index #15=w340, index #16=w309, index #17=w302, index #18=w300, index #19=w299, index #20=w298, index #21=w297, index #22=w296, index #23=w295, index #24=w294, index #25=w293) -> (element #1=w364:u16, element #2=w339:u16, element #3=w338:u16, element #4=w337:u16, element #5=w336:u16, element #6=w335:u16, element #7=w325:u16, element #8=w324:u16, element #9=w320:u16, element #10=w319:u16, element #11=w318:u16, element #12=w317:u16, element #13=w316:u16, element #14=w311:u16, element #15=w310:u16, element #16=w303:u16, element #17=w301:u16, element #18=w292:u16, element #19=w291:u16, element #20=w290:u16, element #21=w289:u16, element #22=w288:u16, element #23=w287:u16, element #24=w286:u16, element #25=w285:u16)
              n177 = local write "Cue1Param_CueType_Switch"(w290) -> ()
              n178 = local write "Cue1Param_AudioLed_Count_Switch"(w289) -> ()
              n179 = local write "Cue1Param_AudioLed_Probability_Switch"(w288) -> ()
              n180 = local write "Cue1Param_CueType_NS"(w287) -> ()
              n181 = local write "Cue1Param_AudioLed_Count_NS"(w286) -> ()
              n182 = local write "Cue1Param_AudioLed_Probability_NS"(w285) -> ()
              n183 = To Double Precision Float(number=w364) -> (double precision float=w363:dbl)
              n184 = To Double Precision Float(number=w339) -> (double precision float=w361:dbl)
              n185 = To Double Precision Float(number=w337) -> (double precision float=w358:dbl)
              n186 = To Double Precision Float(number=w336) -> (double precision float=w357:dbl)
              n187 = To Double Precision Float(number=w335) -> (double precision float=w359:dbl)
              n188 = To Double Precision Float(number=w325) -> (double precision float=w330:dbl)
              n189 = To Double Precision Float(number=w324) -> (double precision float=w326:dbl)
              n190 = To Double Precision Float(number=w320) -> (double precision float=w331:dbl)
              n191 = To Double Precision Float(number=w318) -> (double precision float=w333:dbl)
              n192 = To Double Precision Float(number=w317) -> (double precision float=w334:dbl)
              n193 = To Double Precision Float(number=w316) -> (double precision float=w332:dbl)
              n194 = To Double Precision Float(number=w311) -> (double precision float=w314:dbl)
              n195 = To Double Precision Float(number=w310) -> (double precision float=w315:dbl)
              n196 = To Double Precision Float(number=w303) -> (double precision float=w308:dbl)
              n197 = To Double Precision Float(number=w301) -> (double precision float=w307:dbl)
              n198 = local write "SolenoidProbability_L"(w292) -> ()
              n199 = local write "SolenoidProbability_R"(w291) -> ()
              n200 = Divide(x=w363, y=w304) -> (x/y=w362:dbl)
              n201 = Divide(x=w361, y=w304) -> (x/y=w360:dbl)
              n202 = Divide(x=w358, y=w304) -> (x/y=w355:dbl)
              n203 = Divide(x=w357, y=w304) -> (x/y=w354:dbl)
              n204 = Divide(x=w359, y=w304) -> (x/y=w356:dbl)
              n205 = Divide(x=w330, y=w304) -> (x/y=w328:dbl)
              n206 = Divide(x=w326, y=w304) -> (x/y=w327:dbl)
              n207 = Divide(x=w331, y=w304) -> (x/y=w329:dbl)
              n208 = Divide(x=w333, y=w304) -> (x/y=w323:dbl)
              n209 = Divide(x=w334, y=w304) -> (x/y=w322:dbl)
              n210 = Divide(x=w332, y=w304) -> (x/y=w321:dbl)
              n211 = Divide(x=w314, y=w304) -> (x/y=w313:dbl)
              n212 = Divide(x=w315, y=w304) -> (x/y=w312:dbl)
              n213 = Divide(x=w308, y=w304) -> (x/y=w306:dbl)
              n214 = Divide(x=w307, y=w304) -> (x/y=w305:dbl)
              n215 = local write "FPGA_count2ms"(w362) -> ()
              n216 = local write "Laser_Freq_l1"(w360) -> ()
              n217 = local write "Laser_duration_l1"(w338) -> ()
              n218 = local write "Laser_Tpeak_l1"(w355) -> ()
              n219 = local write "Laser_Tshutter_l1"(w354) -> ()
              n220 = local write "Laser_power_min_l1"(w356) -> ()
              n221 = local write "Laser_power_max_l1"(w328) -> ()
              n222 = local write "Laser_power_step_l1"(w327) -> ()
              n223 = local write "Laser_Freq_l2"(w329) -> ()
              n224 = local write "Laser_duration_l2"(w319) -> ()
              n225 = local write "Laser_Tpeak_l2"(w323) -> ()
              n226 = local write "Laser_Tshutter_l2"(w322) -> ()
              n227 = local write "Laser_power_min_l2"(w321) -> ()
              n228 = local write "Laser_power_max_l2"(w313) -> ()
              n229 = local write "Laser_power_step_l2"(w312) -> ()
              n230 = local write "CueLed_Freq"(w306) -> ()
              n231 = local write "CueLed_Tpeak"(w305) -> ()
            }
            frame "UploadSettings_dataLC_1" {
              # "Cue1_delayOpt_NonSwitch"
              # "ENL1_delayOpt_NonSwitch"
              # "Cue1_delayOpt_Switch"
              # "ENL1_delayOpt_Switch"
              # "Count"
              # "Tdelay"
              # "Prob"
              # "OnOff"
              # "Block"
              # "Count"
              # "Tdelay"
              # "Prob"
              # "OnOff"
              # "Block"
              # "Count"
              # "Tdelay"
              # "Prob"
              # "OnOff"
              # "Block"
              # "ENL1 Switch"
              # "Cue1 NonSwitch"
              # "Cue1 Switch"
              # "ENL1 NonSwitch"
              # "Count"
              # "Tdelay"
              # "Prob"
              # "OnOff"
              # "Block"
              n232 = call "myRIO_BRig_RT_dataLC_ENL1_OnOff_Switch_l1.vi"() -> ("output_ENL1_OnOff_Switch_l1"=w420:i32)  [unwired: 11 in]
              n233 = call "myRIO_BRig_RT_dataLC_ENL1_Tdelay_Switch_l1.vi"() -> ("output_ENL1_Tdelay_Switch_l1"=w419:i32)  [unwired: 11 in]
              n234 = call "myRIO_BRig_RT_dataLC_ENL1_Block_Switch_l1.vi"() -> ("output_ENL1_Block_Switch_l1"=w418:i32)  [unwired: 11 in]
              n235 = call "myRIO_BRig_RT_dataLC_ENL1_Count_Switch_l1.vi"() -> ("output_ENL1_Count_Switch_l1"=w417:i32)  [unwired: 11 in]
              n236 = call "myRIO_BRig_RT_dataLC_ENL1_Probability_Switch_l1.vi"() -> ("output_ENL1_Probability_Switch_l1"=w416:i32)  [unwired: 11 in]
              n237 = call "myRIO_BRig_RT_dataLC_ENL1_OnOff_NS_l1.vi"() -> ("output_ENL1_OnOff_NS_l1"=w415:i32)  [unwired: 11 in]
              n238 = call "myRIO_BRig_RT_dataLC_ENL1_Tdelay_NS_l1.vi"() -> ("output_ENL1_Tdelay_NS_l1"=w414:i32)  [unwired: 11 in]
              n239 = call "myRIO_BRig_RT_dataLC_ENL1_Block_NS_l1.vi"() -> ("output_ENL1_All_Block"=w413:i32)  [unwired: 11 in]
              n240 = call "myRIO_BRig_RT_dataLC_ENL1_Count_NS_l1.vi"() -> ("output_ENL1_Count_NS_l1"=w412:i32)  [unwired: 11 in]
              n241 = call "myRIO_BRig_RT_dataLC_ENL1_Probability_NS_l1.vi"() -> ("output_ENL1_Probability_NS_l1"=w411:i32)  [unwired: 11 in]
              n242 = call "myRIO_BRig_RT_dataLC_Cue1_OnOff_Switch_l1.vi"() -> ("output_Cue1_OnOff_Switch_l1"=w410:i32)  [unwired: 11 in]
              n243 = call "myRIO_BRig_RT_dataLC_Cue1_Tdelay_Switch_l1.vi"() -> ("output_Cue1_Tdelay_Switch_l1"=w409:i32)  [unwired: 11 in]
              n244 = call "myRIO_BRig_RT_dataLC_Cue1_Block_Switch_l1.vi"() -> ("output_Cue1_Block_Switch_l1"=w408:i32)  [unwired: 11 in]
              n245 = call "myRIO_BRig_RT_dataLC_Cue1_Count_Switch_l1.vi"() -> ("output_Cue1_Count_Switch_l1"=w407:i32)  [unwired: 11 in]
              n246 = call "myRIO_BRig_RT_dataLC_Cue1_Probability_Switch_l1.vi"() -> ("output_Cue1_Probability_Switch_l1"=w406:i32)  [unwired: 11 in]
              n247 = call "myRIO_BRig_RT_dataLC_Cue1_OnOff_NS_l1.vi"() -> ("output_Cue1_OnOff_NS_l1"=w405:i32)  [unwired: 11 in]
              n248 = call "myRIO_BRig_RT_dataLC_Cue1_Tdelay_NS_l1.vi"() -> ("output_Cue1_Tdelay_NS_l1"=w404:i32)  [unwired: 11 in]
              n249 = call "myRIO_BRig_RT_dataLC_Cue1_Block_NS_l1.vi"() -> ("output_Cue1_Block_NS_l1"=w403:i32)  [unwired: 11 in]
              n250 = call "myRIO_BRig_RT_dataLC_Cue1_Count_NS_l1.vi"() -> ("output_Cue1_Count_NS_l1"=w402:i32)  [unwired: 11 in]
              n251 = call "myRIO_BRig_RT_dataLC_Cue1_Probability_NS_l1.vi"() -> ("output_Cue1_l1_All_Probability"=w401:i32)  [unwired: 11 in]
              n252 = call "myRIO_BRig_RT_dataLC_ENL1_delayOpt_Switch_l1.vi"() -> ("output_ENL1_delayOpt_Switch_l1"=w380:i32)  [unwired: 11 in]
              n253 = call "myRIO_BRig_RT_dataLC_ENL1_delayOpt_NS_l1.vi"() -> ("output_ENL1_delayOpt_NS_l1"=w379:i32)  [unwired: 11 in]
              n254 = call "myRIO_BRig_RT_dataLC_Cue1_delayOpt_Switch_l1.vi"() -> ("output_Cue1_delayOpt_Switch_l1"=w378:i32)  [unwired: 11 in]
              n255 = call "myRIO_BRig_RT_dataLC_Cue1_delayOpt_NS_l1.vi"() -> ("output_Cue1_delayOpt_NS_l1"=w377:i32)  [unwired: 11 in]
              n256 = Index Array(array=w422, index #1=w420, index #2=w419, index #3=w418, index #4=w417, index #5=w416, index #6=w415, index #7=w414, index #8=w413, index #9=w412, index #10=w411, index #11=w410, index #12=w409, index #13=w408, index #14=w407, index #15=w406, index #16=w405, index #17=w404, index #18=w403, index #19=w402, index #20=w401, index #21=w380, index #22=w379, index #23=w378, index #24=w377) -> (element #1=w400:u16, element #2=w399:u16, element #3=w398:u16, element #4=w397:u16, element #5=w396:u16, element #6=w395:u16, element #7=w394:u16, element #8=w393:u16, element #9=w392:u16, element #10=w391:u16, element #11=w390:u16, element #12=w389:u16, element #13=w388:u16, element #14=w387:u16, element #15=w386:u16, element #16=w385:u16, element #17=w384:u16, element #18=w383:u16, element #19=w382:u16, element #20=w381:u16, element #21=w372:u16, element #22=w371:u16, element #23=w370:u16, element #24=w369:u16)
              n257 = Not Equal To 0?(x=w400) -> (x != 0?=w424:bool)
              n258 = Not Equal To 0?(x=w395) -> (x != 0?=w423:bool)
              n259 = Not Equal To 0?(x=w390) -> (x != 0?=w426:bool)
              n260 = Not Equal To 0?(x=w385) -> (x != 0?=w425:bool)
              n261 = Not Equal To 0?(x=w372) -> (x != 0?=w374:bool)
              n262 = Not Equal To 0?(x=w371) -> (x != 0?=w375:bool)
              n263 = Not Equal To 0?(x=w370) -> (x != 0?=w376:bool)
              n264 = Not Equal To 0?(x=w369) -> (x != 0?=w373:bool)
              n265 = local write "LC_ENL1_OnOff_Switch_l1"(w424) -> ()
              n266 = local write "LC_ENL1_Tdelay_Switch_l1"(w399) -> ()
              n267 = local write "LC_ENL1_Block_Switch_l1"(w398) -> ()
              n268 = local write "LC_ENL1_Count_Switch_l1"(w397) -> ()
              n269 = local write "LC_ENL1_Probability_Switch_l1"(w396) -> ()
              n270 = local write "LC_ENL1_OnOff_NS_l1"(w423) -> ()
              n271 = local write "LC_ENL1_Tdelay_NS_l1"(w394) -> ()
              n272 = local write "LC_ENL1_Block_NS_l1"(w393) -> ()
              n273 = local write "LC_ENL1_Count_NS_l1"(w392) -> ()
              n274 = local write "LC_ENL1_Probability_NS_l1"(w391) -> ()
              n275 = local write "LC_Cue1_OnOff_Switch_l1"(w426) -> ()
              n276 = local write "LC_Cue1_Tdelay_Switch_l1"(w389) -> ()
              n277 = local write "LC_Cue1_Block_Switch_l1"(w388) -> ()
              n278 = local write "LC_Cue1_Count_Switch_l1"(w387) -> ()
              n279 = local write "LC_Cue1_Probability_Switch_l1"(w386) -> ()
              n280 = local write "LC_Cue1_OnOff_NS_l1"(w425) -> ()
              n281 = local write "LC_Cue1_Tdelay_NS_l1"(w384) -> ()
              n282 = local write "LC_Cue1_Block_NS_l1"(w383) -> ()
              n283 = local write "LC_Cue1_Count_NS_l1"(w382) -> ()
              n284 = local write "LC_Cue1_Probability_NS_l1"(w381) -> ()
              n285 = local write "LC_ENL1_delayOpt_Switch_l1"(w374) -> ()
              n286 = local write "LC_ENL1_delayOpt_NS_l1"(w375) -> ()
              n287 = local write "LC_Cue1_delayOpt_Switch_l1"(w376) -> ()
              n288 = local write "LC_Cue1_delayOpt_NS_l1"(w373) -> ()
            }
            frame "UploadSettings_dataLC_3" {
              # "Cue1_delayOpt_NonSwitch"
              # "ENL1_delayOpt_NonSwitch"
              # "Cue1_delayOpt_Switch"
              # "ENL1_delayOpt_Switch"
              # "Count"
              # "Tdelay"
              # "Prob"
              # "OnOff"
              # "Block"
              # "Count"
              # "Tdelay"
              # "Prob"
              # "OnOff"
              # "Block"
              # "Count"
              # "Tdelay"
              # "Prob"
              # "OnOff"
              # "Block"
              # "ENL1 Switch"
              # "Cue1 NonSwitch"
              # "Cue1 Switch"
              # "ENL1 NonSwitch"
              # "Count"
              # "Tdelay"
              # "Prob"
              # "OnOff"
              # "Block"
              n289 = call "myRIO_BRig_RT_dataLC_ENL1_OnOff_Switch_l2.vi"() -> ("output_ENL1_OnOff_Switch_l2"=w447:i32)  [unwired: 11 in]
              n290 = call "myRIO_BRig_RT_dataLC_ENL1_Tdelay_Switch_l2.vi"() -> ("output_ENL1_Tdelay_Switch_l2"=w448:i32)  [unwired: 11 in]
              n291 = call "myRIO_BRig_RT_dataLC_ENL1_Block_Switch_l2.vi"() -> ("output_ENL1_Block_Switch_l2"=w449:i32)  [unwired: 11 in]
              n292 = call "myRIO_BRig_RT_dataLC_ENL1_Count_Switch_l2.vi"() -> ("output_ENL1_Count_Switch_l2"=w450:i32)  [unwired: 11 in]
              n293 = call "myRIO_BRig_RT_dataLC_ENL1_Probability_Switch_l2.vi"() -> ("output_ENL1_Probability_Switch_l2"=w451:i32)  [unwired: 11 in]
              n294 = call "myRIO_BRig_RT_dataLC_ENL1_OnOff_NS_l2.vi"() -> ("output_ENL1_OnOff_NS_l2"=w442:i32)  [unwired: 11 in]
              n295 = call "myRIO_BRig_RT_dataLC_ENL1_Tdelay_NS_l2.vi"() -> ("output_ENL1_Tdelay_NS_l2"=w443:i32)  [unwired: 11 in]
              n296 = call "myRIO_BRig_RT_dataLC_ENL1_Block_NS_l2.vi"() -> ("output_ENL1_Block_NS_l2"=w444:i32)  [unwired: 11 in]
              n297 = call "myRIO_BRig_RT_dataLC_ENL1_Count_NS_l2.vi"() -> ("output_ENL1_Count_NS_l2"=w445:i32)  [unwired: 11 in]
              n298 = call "myRIO_BRig_RT_dataLC_ENL1_Probability_NS_l2.vi"() -> ("output_ENL1_Probability_NS_l2"=w446:i32)  [unwired: 11 in]
              n299 = call "myRIO_BRig_RT_dataLC_Cue1_OnOff_Switch_l2.vi"() -> ("output_Cue1_OnOff_Switch_l2"=w437:i32)  [unwired: 11 in]
              n300 = call "myRIO_BRig_RT_dataLC_Cue1_Tdelay_Switch_l2.vi"() -> ("output_Cue1_Tdelay_Switch_l2"=w438:i32)  [unwired: 11 in]
              n301 = call "myRIO_BRig_RT_dataLC_Cue1_Block_Switch_l2.vi"() -> ("output_Cue1_Block_Switch_l2"=w439:i32)  [unwired: 11 in]
              n302 = call "myRIO_BRig_RT_dataLC_Cue1_Count_Switch_l2.vi"() -> ("output_Cue1_Count_Switch_l2"=w440:i32)  [unwired: 11 in]
              n303 = call "myRIO_BRig_RT_dataLC_Cue1_Probability_Switch_l2.vi"() -> ("output_Cue1_l2_First_Probability"=w441:i32)  [unwired: 11 in]
              n304 = call "myRIO_BRig_RT_dataLC_Cue1_OnOff_NS_l2.vi"() -> ("output_Cue1_OnOff_NS_l2"=w432:i32)  [unwired: 11 in]
              n305 = call "myRIO_BRig_RT_dataLC_Cue1_Tdelay_NS_l2.vi"() -> ("output_Cue1_Tdelay_NS_l2"=w433:i32)  [unwired: 11 in]
              n306 = call "myRIO_BRig_RT_dataLC_Cue1_Block_NS_l2.vi"() -> ("output_Cue1_Block_NS_l2"=w434:i32)  [unwired: 11 in]
              n307 = call "myRIO_BRig_RT_dataLC_Cue1_Count_NS_l2.vi"() -> ("output_Cue1_Count_NS_l2"=w435:i32)  [unwired: 11 in]
              n308 = call "myRIO_BRig_RT_dataLC_Cue1_Probability_NS_l2.vi"() -> ("output_Cue1_l2_All_Probability"=w436:i32)  [unwired: 11 in]
              n309 = call "myRIO_BRig_RT_dataLC_ENL1_delayOpt_Switch_l2.vi"() -> ("output_ENL1_delayOpt_Switch_l2"=w428:i32)  [unwired: 11 in]
              n310 = call "myRIO_BRig_RT_dataLC_ENL1_delayOpt_NS_l2.vi"() -> ("output_ENL1_delayOpt_NS_l2"=w429:i32)  [unwired: 11 in]
              n311 = call "myRIO_BRig_RT_dataLC_Cue1_delayOpt_Switch_l2.vi"() -> ("output_Cue1_delayOpt_Switch_l2"=w430:i32)  [unwired: 11 in]
              n312 = call "myRIO_BRig_RT_dataLC_Cue1_delayOpt_NS_l2.vi"() -> ("output_Cue1_delayOpt_NS_l2"=w431:i32)  [unwired: 11 in]
              n313 = Index Array(array=w481, index #1=w447, index #2=w448, index #3=w449, index #4=w450, index #5=w451, index #6=w442, index #7=w443, index #8=w444, index #9=w445, index #10=w446, index #11=w437, index #12=w438, index #13=w439, index #14=w440, index #15=w441, index #16=w432, index #17=w433, index #18=w434, index #19=w435, index #20=w436, index #21=w428, index #22=w429, index #23=w430, index #24=w431) -> (element #1=w479:u16, element #2=w478:u16, element #3=w477:u16, element #4=w476:u16, element #5=w475:u16, element #6=w474:u16, element #7=w473:u16, element #8=w472:u16, element #9=w471:u16, element #10=w470:u16, element #11=w469:u16, element #12=w468:u16, element #13=w467:u16, element #14=w466:u16, element #15=w465:u16, element #16=w464:u16, element #17=w463:u16, element #18=w462:u16, element #19=w461:u16, element #20=w460:u16, element #21=w455:u16, element #22=w454:u16, element #23=w453:u16, element #24=w452:u16)
              n314 = Not Equal To 0?(x=w479) -> (x != 0?=w483:bool)
              n315 = Not Equal To 0?(x=w474) -> (x != 0?=w482:bool)
              n316 = Not Equal To 0?(x=w469) -> (x != 0?=w485:bool)
              n317 = Not Equal To 0?(x=w464) -> (x != 0?=w484:bool)
              n318 = Not Equal To 0?(x=w455) -> (x != 0?=w457:bool)
              n319 = Not Equal To 0?(x=w454) -> (x != 0?=w458:bool)
              n320 = Not Equal To 0?(x=w453) -> (x != 0?=w459:bool)
              n321 = Not Equal To 0?(x=w452) -> (x != 0?=w456:bool)
              n322 = local write "LC_ENL1_OnOff_Switch_l2"(w483) -> ()
              n323 = local write "LC_ENL1_Tdelay_Switch_l2"(w478) -> ()
              n324 = local write "LC_ENL1_Block_Switch_l2"(w477) -> ()
              n325 = local write "LC_ENL1_Count_Switch_l2"(w476) -> ()
              n326 = local write "LC_ENL1_Probability_Switch_l2"(w475) -> ()
              n327 = local write "LC_ENL1_OnOff_NS_l2"(w482) -> ()
              n328 = local write "LC_ENL1_Tdelay_NS_l2"(w473) -> ()
              n329 = local write "LC_ENL1_Block_NS_l2"(w472) -> ()
              n330 = local write "LC_ENL1_Count_NS_l2"(w471) -> ()
              n331 = local write "LC_ENL1_Probability_NS_l2"(w470) -> ()
              n332 = local write "LC_Cue1_OnOff_Switch_l2"(w485) -> ()
              n333 = local write "LC_Cue1_Tdelay_Switch_l2"(w468) -> ()
              n334 = local write "LC_Cue1_Block_Switch_l2"(w467) -> ()
              n335 = local write "LC_Cue1_Count_Switch_l2"(w466) -> ()
              n336 = local write "LC_Cue1_Probability_Switch_l2"(w465) -> ()
              n337 = local write "LC_Cue1_OnOff_NS_l2"(w484) -> ()
              n338 = local write "LC_Cue1_Tdelay_NS_l2"(w463) -> ()
              n339 = local write "LC_Cue1_Block_NS_l2"(w462) -> ()
              n340 = local write "LC_Cue1_Count_NS_l2"(w461) -> ()
              n341 = local write "LC_Cue1_Probability_NS_l2"(w460) -> ()
              n342 = local write "LC_ENL1_delayOpt_Switch_l2"(w457) -> ()
              n343 = local write "LC_ENL1_delayOpt_NS_l2"(w458) -> ()
              n344 = local write "LC_Cue1_delayOpt_Switch_l2"(w459) -> ()
              n345 = local write "LC_Cue1_delayOpt_NS_l2"(w456) -> ()
            }
            frame "UploadSettings_dataLC_2" {
              # "Count"
              # "Tdelay"
              # "Prob"
              # "OnOff"
              # "Block"
              # "Selection NonSwitch"
              # "Count"
              # "Tdelay"
              # "Prob"
              # "OnOff"
              # "Block"
              # "Selection Switch"
              # "Trial"
              # "Tdelay"
              # "Prob"
              # "OnOff"
              # "Block"
              # "Wrong"
              # "Reward"
              # "Trial"
              # "Tdelay"
              # "Prob"
              # "OnOff"
              # "Block"
              n346 = call "myRIO_BRig_RT_dataLC_Reward_OnOff_l1.vi"() -> ("output_Reward_OnOff_l1"=w528:i32)  [unwired: 11 in]
              n347 = call "myRIO_BRig_RT_dataLC_Reward_Tdelay_l1.vi"() -> ("output_Reward_Tdelay_l1"=w527:i32)  [unwired: 11 in]
              n348 = call "myRIO_BRig_RT_dataLC_Reward_Block_l1.vi"() -> ("output_Reward_Block_l1"=w526:i32)  [unwired: 11 in]
              n349 = call "myRIO_BRig_RT_dataLC_Reward_Trial_l1.vi"() -> ("output_Reward_Trial_l1"=w525:i32)  [unwired: 11 in]
              n350 = call "myRIO_BRig_RT_dataLC_Reward_Probability_l1.vi"() -> ("output_Reward_Probability_l1"=w524:i32)  [unwired: 11 in]
              n351 = call "myRIO_BRig_RT_dataLC_Wrong_OnOff_l1.vi"() -> ("output_Wrong_OnOff_l1"=w517:i32)  [unwired: 11 in]
              n352 = call "myRIO_BRig_RT_dataLC_Wrong_Tdelay_l1.vi"() -> ("output_Wrong_Tdelay_l1"=w516:i32)  [unwired: 11 in]
              n353 = call "myRIO_BRig_RT_dataLC_Wrong_Block_l1.vi"() -> ("output_Wrong_Block_l1"=w515:i32)  [unwired: 11 in]
              n354 = call "myRIO_BRig_RT_dataLC_Wrong_Trial_l1.vi"() -> ("output_Wrong_Trial_l1"=w514:i32)  [unwired: 11 in]
              n355 = call "myRIO_BRig_RT_dataLC_Wrong_Probability_l1.vi"() -> ("output_Wrong_Probability_l1"=w513:i32)  [unwired: 11 in]
              n356 = call "myRIO_BRig_RT_dataLC_Selection_OnOff_Switch_l1.vi"() -> ("output_Selection_OnOff_Switch_l1"=w508:i32)  [unwired: 11 in]
              n357 = call "myRIO_BRig_RT_dataLC_Selection_Tdelay_Switch_l1.vi"() -> ("output_Selection_Tdelay_Switch_l1"=w507:i32)  [unwired: 11 in]
              n358 = call "myRIO_BRig_RT_dataLC_Selection_Block_Switch_l1.vi"() -> ("output_Selection_Block_Switch_l1"=w506:i32)  [unwired: 11 in]
              n359 = call "myRIO_BRig_RT_dataLC_Selection_Count_Switch_l1.vi"() -> ("output_Selection_Count_Switch_l1"=w505:i32)  [unwired: 11 in]
              n360 = call "myRIO_BRig_RT_dataLC_Selection_Probability_Switch_l1.vi"() -> ("output_Selection_Probability_Switch_l1"=w504:i32)  [unwired: 11 in]
              n361 = call "myRIO_BRig_RT_dataLC_Selection_OnOff_NS_l1.vi"() -> ("output_Selection_OnOff_NS_l1"=w503:i32)  [unwired: 11 in]
              n362 = call "myRIO_BRig_RT_dataLC_Selection_Tdelay_NS_l1.vi"() -> ("output_Selection_Tdelay_NS_l1"=w502:i32)  [unwired: 11 in]
              n363 = call "myRIO_BRig_RT_dataLC_Selection_Block_NS_l1.vi"() -> ("output_Selection_Block_NS_l1"=w501:i32)  [unwired: 11 in]
              n364 = call "myRIO_BRig_RT_dataLC_Selection_Count_NS_l1.vi"() -> ("output_Selection_Count_NS_l1"=w500:i32)  [unwired: 11 in]
              n365 = call "myRIO_BRig_RT_dataLC_Selection_Probability_NS_l1.vi"() -> ("output_Selection_Probability_NS_l1"=w499:i32)  [unwired: 11 in]
              n366 = Index Array(array=w529, index #1=w528, index #2=w527, index #3=w526, index #4=w525, index #5=w524, index #6=w517, index #7=w516, index #8=w515, index #9=w514, index #10=w513, index #11=w508, index #12=w507, index #13=w506, index #14=w505, index #15=w504, index #16=w503, index #17=w502, index #18=w501, index #19=w500, index #20=w499) -> (element #1=w523:u16, element #2=w522:u16, element #3=w521:u16, element #4=w520:u16, element #5=w519:u16, element #6=w518:u16, element #7=w512:u16, element #8=w511:u16, element #9=w510:u16, element #10=w509:u16, element #11=w496:u16, element #12=w495:u16, element #13=w494:u16, element #14=w493:u16, element #15=w492:u16, element #16=w491:u16, element #17=w490:u16, element #18=w489:u16, element #19=w488:u16, element #20=w487:u16)
              n367 = Not Equal To 0?(x=w523) -> (x != 0?=w531:bool)
              n368 = Not Equal To 0?(x=w518) -> (x != 0?=w530:bool)
              n369 = Not Equal To 0?(x=w496) -> (x != 0?=w498:bool)
              n370 = Not Equal To 0?(x=w491) -> (x != 0?=w497:bool)
              n371 = local write "LC_Reward_OnOff_l1"(w531) -> ()
              n372 = local write "LC_Reward_Tdelay_l1"(w522) -> ()
              n373 = local write "LC_Reward_Block_l1"(w521) -> ()
              n374 = local write "LC_Reward_Trial_l1"(w520) -> ()
              n375 = local write "LC_Reward_Probability_l1"(w519) -> ()
              n376 = local write "LC_Wrong_OnOff_l1"(w530) -> ()
              n377 = local write "LC_Wrong_Tdelay_l1"(w512) -> ()
              n378 = local write "LC_Wrong_Block_l1"(w511) -> ()
              n379 = local write "LC_Wrong_Trial_l1"(w510) -> ()
              n380 = local write "LC_Wrong_Probability_l1"(w509) -> ()
              n381 = local write "LC_Sel_OnOff_Switch_l1"(w498) -> ()
              n382 = local write "LC_Sel_Tdelay_Switch_l1"(w495) -> ()
              n383 = local write "LC_Sel_Block_Switch_l1"(w494) -> ()
              n384 = local write "LC_Sel_Count_Switch_l1"(w493) -> ()
              n385 = local write "LC_Sel_Probability_Switch_l1"(w492) -> ()
              n386 = local write "LC_Sel_OnOff_NS_l1"(w497) -> ()
              n387 = local write "LC_Sel_Tdelay_NS_l1"(w490) -> ()
              n388 = local write "LC_Sel_Block_NS_l1"(w489) -> ()
              n389 = local write "LC_Sel_Count_NS_l1"(w488) -> ()
              n390 = local write "LC_Sel_Probability_NS_l1"(w487) -> ()
            }
            frame "UploadSettings_dataLC_4" {
              # "Count"
              # "Tdelay"
              # "Prob"
              # "OnOff"
              # "Block"
              # "Selection NonSwitch"
              # "Count"
              # "Tdelay"
              # "Prob"
              # "OnOff"
              # "Block"
              # "Selection Switch"
              # "Trial"
              # "Tdelay"
              # "Prob"
              # "OnOff"
              # "Block"
              # "Wrong"
              # "Reward"
              # "Trial"
              # "Tdelay"
              # "Prob"
              # "OnOff"
              # "Block"
              n391 = call "myRIO_BRig_RT_dataLC_Reward_OnOff_l2.vi"() -> ("output_Reward_OnOff_l2"=w539:i32)  [unwired: 11 in]
              n392 = call "myRIO_BRig_RT_dataLC_Reward_Tdelay_l2.vi"() -> ("output_Reward_Tdelay_l2"=w540:i32)  [unwired: 11 in]
              n393 = call "myRIO_BRig_RT_dataLC_Reward_Block_l2.vi"() -> ("output_Reward_Block_l2"=w541:i32)  [unwired: 11 in]
              n394 = call "myRIO_BRig_RT_dataLC_Reward_Trial_l2.vi"() -> ("output_Reward_Trial_l2"=w542:i32)  [unwired: 11 in]
              n395 = call "myRIO_BRig_RT_dataLC_Reward_Probability_l2.vi"() -> ("output_Reward_Probability_l2"=w543:i32)  [unwired: 11 in]
              n396 = call "myRIO_BRig_RT_dataLC_Wrong_OnOff_l2.vi"() -> ("output_Wrong_OnOff_l2"=w534:i32)  [unwired: 11 in]
              n397 = call "myRIO_BRig_RT_dataLC_Wrong_Tdelay_l2.vi"() -> ("output_Wrong_Tdelay_l2"=w535:i32)  [unwired: 11 in]
              n398 = call "myRIO_BRig_RT_dataLC_Wrong_Block_l2.vi"() -> ("output_Wrong_Block_l2"=w536:i32)  [unwired: 11 in]
              n399 = call "myRIO_BRig_RT_dataLC_Wrong_Trial_l2.vi"() -> ("output_Wrong_Trial_l2"=w537:i32)  [unwired: 11 in]
              n400 = call "myRIO_BRig_RT_dataLC_Wrong_Probability_l2.vi"() -> ("output_Wrong_Probability_l2"=w538:i32)  [unwired: 11 in]
              n401 = call "myRIO_BRig_RT_dataLC_Selection_OnOff_Switch_l2.vi"() -> ("output_Selection_OnOff_Switch_l2"=w549:i32)  [unwired: 11 in]
              n402 = call "myRIO_BRig_RT_dataLC_Selection_Tdelay_Switch_l2.vi"() -> ("output_Selection_Tdelay_Switch_l2"=w550:i32)  [unwired: 11 in]
              n403 = call "myRIO_BRig_RT_dataLC_Selection_Block_Switch_l2.vi"() -> ("output_Selection_Block_Switch_l2"=w551:i32)  [unwired: 11 in]
              n404 = call "myRIO_BRig_RT_dataLC_Selection_Count_Switch_l2.vi"() -> ("output_Selection_Count_Switch_l2"=w552:i32)  [unwired: 11 in]
              n405 = call "myRIO_BRig_RT_dataLC_Selection_Probability_Switch_l2.vi"() -> ("output_Selection_Probability_Switch_l1"=w553:i32)  [unwired: 11 in]
              n406 = call "myRIO_BRig_RT_dataLC_Selection_OnOff_NS_l2.vi"() -> ("output_Selection_OnOff_NS_l2"=w544:i32)  [unwired: 11 in]
              n407 = call "myRIO_BRig_RT_dataLC_Selection_Tdelay_NS_l2.vi"() -> ("output_Selection_Tdelay_NS_l2"=w545:i32)  [unwired: 11 in]
              n408 = call "myRIO_BRig_RT_dataLC_Selection_Block_NS_l2.vi"() -> ("output_Selection_Block_NS_l2"=w546:i32)  [unwired: 11 in]
              n409 = call "myRIO_BRig_RT_dataLC_Selection_Count_NS_l2.vi"() -> ("output_Selection_Count_NS_l2"=w547:i32)  [unwired: 11 in]
              n410 = call "myRIO_BRig_RT_dataLC_Selection_Probability_NS_l2.vi"() -> ("output_Selection_Probability_NS_l2"=w548:i32)  [unwired: 11 in]
              n411 = Index Array(array=w576, index #1=w539, index #2=w540, index #3=w541, index #4=w542, index #5=w543, index #6=w534, index #7=w535, index #8=w536, index #9=w537, index #10=w538, index #11=w549, index #12=w550, index #13=w551, index #14=w552, index #15=w553, index #16=w544, index #17=w545, index #18=w546, index #19=w547, index #20=w548) -> (element #1=w575:u16, element #2=w574:u16, element #3=w573:u16, element #4=w572:u16, element #5=w571:u16, element #6=w570:u16, element #7=w569:u16, element #8=w568:u16, element #9=w567:u16, element #10=w566:u16, element #11=w563:u16, element #12=w562:u16, element #13=w561:u16, element #14=w560:u16, element #15=w559:u16, element #16=w558:u16, element #17=w557:u16, element #18=w556:u16, element #19=w555:u16, element #20=w554:u16)
              n412 = Not Equal To 0?(x=w575) -> (x != 0?=w578:bool)
              n413 = Not Equal To 0?(x=w570) -> (x != 0?=w577:bool)
              n414 = Not Equal To 0?(x=w563) -> (x != 0?=w565:bool)
              n415 = Not Equal To 0?(x=w558) -> (x != 0?=w564:bool)
              n416 = local write "LC_Reward_OnOff_l2"(w578) -> ()
              n417 = local write "LC_Reward_Tdelay_l2"(w574) -> ()
              n418 = local write "LC_Reward_Block_l2"(w573) -> ()
              n419 = local write "LC_Reward_Trial_l2"(w572) -> ()
              n420 = local write "LC_Reward_Probability_l2"(w571) -> ()
              n421 = local write "LC_Wrong_OnOff_l2"(w577) -> ()
              n422 = local write "LC_Wrong_Tdelay_l2"(w569) -> ()
              n423 = local write "LC_Wrong_Block_l2"(w568) -> ()
              n424 = local write "LC_Wrong_Trial_l2"(w567) -> ()
              n425 = local write "LC_Wrong_Probability_l2"(w566) -> ()
              n426 = local write "LC_Sel_OnOff_Switch_l2"(w565) -> ()
              n427 = local write "LC_Sel_Tdelay_Switch_l2"(w562) -> ()
              n428 = local write "LC_Sel_Block_Switch_l2"(w561) -> ()
              n429 = local write "LC_Sel_Count_Switch_l2"(w560) -> ()
              n430 = local write "LC_Sel_Probability_Switch_l2"(w559) -> ()
              n431 = local write "LC_Sel_OnOff_NS_l2"(w564) -> ()
              n432 = local write "LC_Sel_Tdelay_NS_l2"(w557) -> ()
              n433 = local write "LC_Sel_Block_NS_l2"(w556) -> ()
              n434 = local write "LC_Sel_Count_NS_l2"(w555) -> ()
              n435 = local write "LC_Sel_Probability_NS_l2"(w554) -> ()
            }
            frame "UploadSettings_dataMTrig_1" {
              # "Tdelay_R"
              # "Tdelay_L"
              # "Tcycle_R"
              # "Tcycle_L"
              # "RewCalib_nCycle_R"
              # "RewCalib_nCycle_L"
              # "Solenoid"
              # "Laser_Tcycle"
              n436 = call "myRIO_BRig_RT_dataMTrig_Laser_Tcycle.vi"() -> ("output_Laser_Tcycle"=w588:i32)  [unwired: 11 in]
              n437 = call "myRIO_BRig_RT_dataMTrig_Solenoid_RewCalib_nCycle__L.vi"() -> ("output_Solenoid_RewCalib_nCycle__L"=w587:i32)  [unwired: 11 in]
              n438 = call "myRIO_BRig_RT_dataMTrig_Solenoid_RewCalib_nCycle__R.vi"() -> ("output_Solenoid_RewCalib_nCycle__R"=w586:i32)  [unwired: 11 in]
              n439 = call "myRIO_BRig_RT_dataMTrig_Solenoid_Tdelay__L.vi"() -> ("output_Solenoid_Tdelay__L"=w583:i32)  [unwired: 11 in]
              n440 = call "myRIO_BRig_RT_dataMTrig_Solenoid_Tdelay__R.vi"() -> ("output_Solenoid_Tdelay__R"=w582:i32)  [unwired: 11 in]
              n441 = call "myRIO_BRig_RT_dataMTrig_Solenoid_Tcycle__L.vi"() -> ("output_Solenoid_Tcycle__L"=w585:i32)  [unwired: 11 in]
              n442 = call "myRIO_BRig_RT_dataMTrig_Solenoid_Tcycle__R.vi"() -> ("output_Solenoid_Tcycle__R"=w584:i32)  [unwired: 11 in]
              n443 = Index Array(array=w581, index #1=w588, index #2=w587, index #3=w586, index #4=w585, index #5=w584, index #6=w583, index #7=w582) -> (element #1=w595:u16, element #2=w594:u16, element #3=w593:u16, element #4=w592:u16, element #5=w591:u16, element #6=w590:u16, element #7=w589:u16)
              n444 = Replace Array Subset(array=w597, new element #1=w595, index #1=w588, new element #2=w594, index #2=w587, new element #3=w593, index #3=w586, new element #4=w592, index #4=w585, new element #5=w591, index #5=w584, new element #6=w590, index #6=w583, new element #7=w589, index #7=w582) -> (w596:u16[])
              n445 = local write "MTrig_Solenoid_Tcycle__L"(w592) -> ()
              n446 = local write "MTrig_Solenoid_Tcycle__R"(w591) -> ()
              n447 = local write "MTrig_Laser_Tcycle"(w595) -> ()
            }
            frame "Idle" {
              # "There are a number of tasks we need to perform\nwhile idling. To preserve our timing loop, we\nbreak up the IDLE state into smaller states"
              # "Laser_Tcycle"
              # "Audio_Tcycle_R"
              # "Audio_Tcycle_L"
              n448 = local read "Laser_power_min_l1"() -> (w608:dbl)
              n449 = local read "Laser_power_min_l2"() -> (w607:dbl)
              n450 = local read "Audio_Amp__R"() -> (w610:u16)
              n451 = local read "Audio_Amp__L"() -> (w612:u16)
              n452 = local read "Audio_Freq__R"() -> (w609:u8)
              n453 = local read "Audio_Freq__L"() -> (w611:u8)
              n454 = local read "CueLed_baseline"() -> (w603:bool)
              n455 = local read "Laser2_baseline"() -> (w602:bool)
              n456 = local read "Laser1_baseline"() -> (w601:bool)
              n457 = Select(t=myRIO_BRig_RT__Case_NonExp_stateList."SendData" ("Enum"), s="SendData", f=myRIO_BRig_RT__Case_NonExp_stateList."Idle_2" ("Enum")) -> (s? t:f=w617:T1)
              n458 = call "myRIO__convert__Voltage_to_FPGAvalue.vi"("input_voltage"=w608) -> ("output_PortA"=w599:u16)  [unwired: 9 in, 1 out]
              n459 = call "myRIO__convert__Voltage_to_FPGAvalue.vi"("input_voltage"=w607) -> ("output_PortA"=w600:u16)  [unwired: 9 in, 1 out]
              n460 = Select(t=myRIO_BRig_RT__Case_NonExp_stateList."TestConnection" ("Enum"), s="TestConnection", f=w617) -> (s? t:f=w621:T1)
              n461 = xnode "Read/Write Control"("FPGA VI Reference In"=w614, "error in"=w613, "audioAmp_L"=w612, "audioFreq_L_kHz"=w611, "audioAmp_R"=w610, "audioFreq_R_kHz"=w609, "AnaOut_0"=w599, "AnaOut_1"=w600, "CueLed_Baseline"=w603, "L2Led_Baseline"=w602, "L1Led_Baseline"=w601) -> ("error out"=w606:errorcluster)  [unwired: 1 out]
              n462 = call "myRIO_BRig_RT_dataMTrig_Audio_Tcycle__L.vi"() -> ("output_Audio_Tcycle__L"=w628:i32)  [unwired: 11 in]
              n463 = call "myRIO_BRig_RT_dataMTrig_Audio_Tcycle__R.vi"() -> ("output_Audio_Tcycle__R"=w627:i32)  [unwired: 11 in]
              n464 = call "myRIO_BRig_RT_dataMTrig_Laser_Tcycle.vi"() -> ("output_Laser_Tcycle"=w626:i32)  [unwired: 11 in]
              n465 = call "myRIO_BRig_RT_dataMTrig_CueLed_Tcycle.vi"() -> ("output_CueLed_Tcycle"=w605:i32)  [unwired: 11 in]
              n466 = local write "error out"(w606) -> ()
              n467 = local read "Tcycle_Cue_Audio_min"() -> (w616:u16)
              n468 = local read "MTrig_Laser_Tcycle"() -> (w615:u16)
              n469 = local read "Tcycle_Cue_LED_min"() -> (w604:u16)
              n470 = Replace Array Subset(array=w624, new element #1=w616, index #1=w628, new element #2=w616, index #2=w627, new element #3=w615, index #3=w626, new element #4=w604, index #4=w605) -> (w625:u16[])
            }
            frame "Idle_2" {
              w651 = u16 0 ("t")
              # "There are a number of tasks we need to perform\nwhile idling. To preserve our timing loop, we\nbreak up the IDLE state into smaller states"
              # "Ncycles"
              # "Ncycles"
              # "RewCalib"
              # "RewCalib"
              # "Solenoid R"
              # "Solenoid L"
              n471 = local read "MTrig_Laser_Switch"() -> (w644:bool)
              n472 = local read "count_warmup_R"() -> (w650:u16)
              n473 = local read "count_warmup_L"() -> (w655:u16)
              n474 = call "myRIO_BRig_RT_dataMTrig_Solenoid_RewCalib_OnOff__R.vi"() -> ("output_Solenoid_RewCalib_OnOff__R"=w666:i32)  [unwired: 11 in]
              n475 = call "myRIO_BRig_RT_dataMTrig_Solenoid_N__R.vi"() -> ("output_Solenoid_N__R"=w665:i32)  [unwired: 11 in]
              n476 = call "myRIO_BRig_RT_dataMTrig_Solenoid_RewCalib_OnOff__L.vi"() -> ("output_Solenoid_RewCalib_OnOff__L"=w681:i32)  [unwired: 11 in]
              n477 = call "myRIO_BRig_RT_dataMTrig_Solenoid_N__L.vi"() -> ("output_Solenoid_N__L"=w669:i32)  [unwired: 11 in]
              n478 = case shown="False" w644 {
                tunnel: "LR_reward_Event" -> [w687 w691]
                tunnel: "LR_wrong_Event" -> [w686 w690]
                tunnel: "LR_reward_Laser" -> [w685 w689]
                tunnel: "LR_wrong_Laser" -> [w684 w688]
                tunnel: [w687 _] -> w639
                tunnel: [w686 _] -> w638
                tunnel: [w685 _] -> w637
                tunnel: [w684 _] -> w636
                tunnel: [_ w691] -> w635
                tunnel: [_ w690] -> w634
                tunnel: [_ w689] -> w633
                tunnel: [_ w688] -> w632
                frame False {
                }
                frame True {
                }
              }
              n479 = Index Array(array=w672, index #1=w681, index #2=w669, index #3=w666, index #4=w665) -> (element #1=w668:u16, element #2=w663:u16, element #3=w664:u16, element #4=w662:u16)
              n480 = Select(t=w651, s="count_warmup_L_reset", f=w655) -> (s? t:f=→"count_warmup_L":u16)
              n481 = Select(t=w651, s="count_warmup_R_reset", f=w650) -> (s? t:f=→"count_warmup_R":u16)
              n482 = local read "RewCalib_Trig_L"() -> (w661:bool)
              n483 = local read "RewCalib_Trig_R"() -> (w660:bool)
              n484 = Equal To 0?(x=w663) -> (x = 0?=w671:bool)
              n485 = Equal To 0?(x=w662) -> (x = 0?=w670:bool)
              n486 = Not Equal To 0?(x=w664) -> (x != 0?=w682:bool)
              n487 = Not Equal To 0?(x=w668) -> (x != 0?=w683:bool)
              n488 = And(x=w671, y=w670) -> (x .and. y?=w675:bool)
              n489 = Or(x=w661, y=w660) -> (x .or. y?=w676:bool)
              n490 = Not Exclusive Or(1:w683, 2:w661) -> (0:w678:bool)
              n491 = xnode "Read/Write Control"("FPGA VI Reference In"=w630, "error in"=w631, "Left(F)_or_Right(T)"="Left(F)_or_Right(T)", "SelectionState"="SelectionState", "ignoreWrong"="ignoreWrong", "LR_reward_Event_l1"=w639, "LR_wrong_Event_l1"=w638, "LR_reward_Laser_l1"=w637, "LR_wrong_Laser_l1"=w636, "LR_reward_Event_l2"=w635, "LR_wrong_Event_l2"=w634, "LR_reward_Laser_l2"=w633, "LR_wrong_laser_l2"=w632) -> ("error out"=w629:errorcluster, "SelectReward"=→"SelectReward":bool, "SelectWrong"=→"SelectWrong":bool)  [unwired: 1 out]
              n492 = Not Exclusive Or(1:w682, 2:w660) -> (0:w680:bool)
              n493 = And(x=w676, y=w675) -> (x .and. y?=w658:bool)
              n494 = Not(x=w678) -> (.not. x?=w677:bool)
              n495 = Not(x=w680) -> (.not. x?=w679:bool)
              n496 = Or(x=w677, y=w679) -> (x .or. y?=w659:bool)
              n497 = Or(x=w658, y=w659) -> (x .or. y?=w674:bool)
              n498 = local write "error out"(w629) -> ()
              n499 = Select(t=myRIO_BRig_RT__Case_NonExp_stateList."RewardCalibration_pre" ("Enum"), s=w674, f=myRIO_BRig_RT__Case_NonExp_stateList."Idle_3" ("Enum")) -> (s? t:f=w657:T1)
            }
            frame "Idle_3" {
              # "There are a number of tasks we need to perform\nwhile idling. To preserve our timing loop, we\nbreak up the IDLE state into smaller states"
              n500 = local read "Laser_Tshutter_l1"() -> (w710:dbl)
              n501 = local read "Laser_duration_l1"() -> (w709:u16)
              n502 = local read "Laser_Tshutter_l2"() -> (w706:dbl)
              n503 = local read "Laser_duration_l2"() -> (w705:u16)
              n504 = local read "Laser_Tpeak_l1"() -> (w712:dbl)
              n505 = local read "Laser_Tpeak_l2"() -> (w708:dbl)
              n506 = local read "CueLed_Tpeak"() -> (w703:dbl)
              n507 = local read "Laser_Freq_l1"() -> (w711:dbl)
              n508 = local read "Laser_Freq_l2"() -> (w707:dbl)
              n509 = local read "CueLed_Freq"() -> (w702:dbl)
              n510 = local read "FPGA_count2ms"() -> (w704:dbl)
              n511 = To Unsigned Word Integer(number=w704) -> (unsigned 16bit integer=w713:u16)
              n512 = call "myRIO_BRig_RT__calc_laser_FPGA_N.vi"("input_FPGA_ms2count"=w704, "input_Tpeak"=w712, "input_Freq"=w711, "input_Tshutter"=w710, "input_duration"=w709) -> ("output_laser_Npeak"=w701:u32, "output_laser_Nvalley"=w699:u32, "output_laser_Nshutter"=w697:u32, "output_laser_Nduration"=w695:u32)  [unwired: 6 in, 1 out]
              n513 = call "myRIO_BRig_RT__calc_laser_FPGA_N.vi"("input_FPGA_ms2count"=w704, "input_Tpeak"=w708, "input_Freq"=w707, "input_Tshutter"=w706, "input_duration"=w705) -> ("output_laser_Npeak"=w700:u32, "output_laser_Nvalley"=w698:u32, "output_laser_Nshutter"=w696:u32, "output_laser_Nduration"=w694:u32)  [unwired: 6 in, 1 out]
              n514 = call "myRIO_BRig_RT__calc_laser_FPGA_N__CueLed.vi"("input_FPGA_ms2count"=w704, "input_Tpeak"=w703, "input_Freq"=w702) -> ("output_laser_Npeak"=w693:u32, "output_laser_Nvalley"=w692:u32)  [unwired: 11 in]
              n515 = xnode "Read/Write Control"("FPGA VI Reference In"=w718, "error in"=w717, "k1__counter_per_ms"=w713, "LC_nPeak_l1"=w701, "LC_nPeak_l2"=w700, "LC_nValley_l1"=w699, "LC_nValley_l2"=w698, "LC_nShutter_l1"=w697, "LC_nShutter_l2"=w696, "LR_reward_nTotal_l1"=w695, "LR_wrong_nTotal_l1"=w695, "LR_reward_nTotal_l2"=w694, "LR_wrong_nTotal_l2"=w694, "CueLed_nPeak"=w693, "CueLed_nValley"=w692) -> ("error out"=w714:errorcluster)  [unwired: 1 out]
              n516 = local write "error out"(w714) -> ()
            }
            frame "Idle_4" {
              w740 = u8 0 ("f")
              # "There are a number of tasks we need to perform\nwhile idling. To preserve our timing loop, we\nbreak up the IDLE state into smaller states"
              n517 = local read "MTrig_Solenoid_trig__L"() -> (w731:bool)
              n518 = local read "MTrig_Solenoid_trig__R"() -> (w741:bool)
              n519 = local read "warmupType"() -> (w724:u8)
              n520 = local read "warmup"() -> (w733:bool)
              n521 = Not Equal To 0?(x=w724) -> (x != 0?=w723:bool)
              n522 = Not(x=w723) -> (.not. x?=w734:bool)
              n523 = Select(t=u8 1, s=w731, f=w740) -> (s? t:f=w739:u8)
              n524 = Select(t=u8 2, s=w741, f=w740) -> (s? t:f=w738:u8)
              n525 = And(x=w733, y=w734) -> (x .and. y?=w732:bool)
              n526 = And(x=w733, y=w723) -> (x .and. y?=w727:bool)
              n527 = Add(x=w739, y=w738) -> (x+y=w737:u8)
              n528 = case shown="3" w737 {
                tunnel: w736 -> [w744 w748 w781 w812]
                tunnel: [w744 w747 w780 w811] -> w735
                tunnel: w732 -> [_ w746 w779 w810]
                tunnel: [_ TRUE TRUE TRUE] -> w729
                frame 0, Default {
                }
                frame 1 {
                  n529 = case shown="False" w746 {
                    tunnel: w748 -> [w761 w776]
                    tunnel: [w760 w775] -> w747
                    frame True {
                      # "Audio_L"
                      # "Solenoid_L"
                      n530 = call "myRIO_BRig_RT_dataMTrig_Solenoid_N__L.vi"() -> ("output_Solenoid_N__L"=w758:i32)  [unwired: 11 in]
                      n531 = call "myRIO_BRig_RT_dataMTrig_Audio_N__L.vi"() -> ("output_Audio_N__L"=w756:i32)  [unwired: 11 in]
                      n532 = call "myRIO_BRig_RT_dataMTrig_Audio_N__R.vi"() -> ("output_Audio_N__R"=w751:i32)  [unwired: 11 in]
                      n533 = local read "sp_LeftSpout"() -> (w755:u16)
                      n534 = Index Array(array=w761, index #1=w758, index #2=w756, index #3=w751) -> (element #1=w759:u16, element #2=w754:u16, element #3=w753:u16)
                      n535 = Increment(x=w759) -> (x+1=w757:u16)
                      n536 = case shown="2" w755 {
                        tunnel: w754 -> [w764 w767 w769]
                        tunnel: w753 -> [w762 w766 w771]
                        tunnel: [w763 w767 w768] -> w752
                        tunnel: [w762 w765 w770] -> w750
                        frame 0, Default {
                          n537 = Increment(x=w764) -> (x+1=w763:u16)
                        }
                        frame 1 {
                          n538 = Increment(x=w766) -> (x+1=w765:u16)
                        }
                        frame 2 {
                          n539 = Increment(x=w771) -> (x+1=w770:u16)
                          n540 = Increment(x=w769) -> (x+1=w768:u16)
                        }
                      }
                      n541 = Replace Array Subset(array=w761, new element #1=w757, index #1=w758, new element #2=w752, index #2=w756, new element #3=w750, index #3=w751) -> (w760:u16[])
                    }
                    frame False {
                      # "Solenoid_L"
                      n542 = call "myRIO_BRig_RT_dataMTrig_Solenoid_N__L.vi"() -> ("output_Solenoid_N__L"=w773:i32)  [unwired: 11 in]
                      n543 = Index Array(array=w776, index=w773) -> (element=w774:u16)
                      n544 = Increment(x=w774) -> (x+1=w772:u16)
                      n545 = Replace Array Subset(array=w776, new element=w772, index=w773) -> (w775:u16[])
                    }
                  }
                  n546 = local write "MTrig_Solenoid_trig__L"(FALSE) -> ()
                }
                frame 2 {
                  n547 = case shown="True" w779 {
                    tunnel: w781 -> [w793 w808]
                    tunnel: [w792 w807] -> w780
                    frame True {
                      # "Solenoid_R"
                      n548 = call "myRIO_BRig_RT_dataMTrig_Solenoid_N__R.vi"() -> ("output_Solenoid_N__R"=w782:i32)  [unwired: 11 in]
                      n549 = call "myRIO_BRig_RT_dataMTrig_Audio_N__L.vi"() -> ("output_Audio_N__L"=w789:i32)  [unwired: 11 in]
                      n550 = call "myRIO_BRig_RT_dataMTrig_Audio_N__R.vi"() -> ("output_Audio_N__R"=w784:i32)  [unwired: 11 in]
                      n551 = local read "sp_RightSpout"() -> (w788:u16)
                      n552 = Index Array(array=w793, index #1=w782, index #2=w789, index #3=w784) -> (element #1=w791:u16, element #2=w787:u16, element #3=w786:u16)
                      n553 = Increment(x=w791) -> (x+1=w790:u16)
                      n554 = case shown="2" w788 {
                        tunnel: w787 -> [w796 w799 w801]
                        tunnel: w786 -> [w794 w798 w803]
                        tunnel: [w795 w799 w800] -> w785
                        tunnel: [w794 w797 w802] -> w783
                        frame 0, Default {
                          n555 = Increment(x=w796) -> (x+1=w795:u16)
                        }
                        frame 1 {
                          n556 = Increment(x=w798) -> (x+1=w797:u16)
                        }
                        frame 2 {
                          n557 = Increment(x=w803) -> (x+1=w802:u16)
                          n558 = Increment(x=w801) -> (x+1=w800:u16)
                        }
                      }
                      n559 = Replace Array Subset(array=w793, new element #1=w790, index #1=w782, new element #2=w785, index #2=w789, new element #3=w783, index #3=w784) -> (w792:u16[])
                    }
                    frame False {
                      # "Solenoid_R"
                      n560 = call "myRIO_BRig_RT_dataMTrig_Solenoid_N__R.vi"() -> ("output_Solenoid_N__R"=w804:i32)  [unwired: 11 in]
                      n561 = Index Array(array=w808, index=w804) -> (element=w806:u16)
                      n562 = Increment(x=w806) -> (x+1=w805:u16)
                      n563 = Replace Array Subset(array=w808, new element=w805, index=w804) -> (w807:u16[])
                    }
                  }
                  n564 = local write "MTrig_Solenoid_trig__R"(FALSE) -> ()
                }
                frame 3 {
                  w813 = FALSE
                  n565 = case shown="True" w810 {
                    tunnel: w812 -> [w827 w835]
                    tunnel: [w826 w834] -> w811
                    frame True {
                      # "Audio_R"
                      # "Solenoid_R"
                      # "Audio_L"
                      # "Solenoid_L"
                      n566 = call "myRIO_BRig_RT_dataMTrig_Solenoid_N__L.vi"() -> ("output_Solenoid_N__L"=w821:i32)  [unwired: 11 in]
                      n567 = call "myRIO_BRig_RT_dataMTrig_Audio_N__L.vi"() -> ("output_Audio_N__L"=w819:i32)  [unwired: 11 in]
                      n568 = call "myRIO_BRig_RT_dataMTrig_Solenoid_N__R.vi"() -> ("output_Solenoid_N__R"=w817:i32)  [unwired: 11 in]
                      n569 = call "myRIO_BRig_RT_dataMTrig_Audio_N__R.vi"() -> ("output_Audio_N__R"=w816:i32)  [unwired: 11 in]
                      n570 = Index Array(array=w827, index #1=w821, index #2=w819, index #3=w817, index #4=w816) -> (element #1=w825:u16, element #2=w824:u16, element #3=w823:u16, element #4=w822:u16)
                      n571 = Increment(x=w822) -> (x+1=w814:u16)
                      n572 = Increment(x=w825) -> (x+1=w820:u16)
                      n573 = Increment(x=w824) -> (x+1=w818:u16)
                      n574 = Increment(x=w823) -> (x+1=w815:u16)
                      n575 = Replace Array Subset(array=w827, new element #1=w820, index #1=w821, new element #2=w818, index #2=w819, new element #3=w815, index #3=w817, new element #4=w814, index #4=w816) -> (w826:u16[])
                    }
                    frame False {
                      # "Solenoid_R"
                      # "Solenoid_L"
                      n576 = call "myRIO_BRig_RT_dataMTrig_Solenoid_N__L.vi"() -> ("output_Solenoid_N__L"=w831:i32)  [unwired: 11 in]
                      n577 = call "myRIO_BRig_RT_dataMTrig_Solenoid_N__R.vi"() -> ("output_Solenoid_N__R"=w828:i32)  [unwired: 11 in]
                      n578 = Index Array(array=w835, index #1=w831, index #2=w828) -> (element #1=w833:u16, element #2=w832:u16)
                      n579 = Increment(x=w833) -> (x+1=w830:u16)
                      n580 = Increment(x=w832) -> (x+1=w829:u16)
                      n581 = Replace Array Subset(array=w835, new element #1=w830, index #1=w831, new element #2=w829, index #2=w828) -> (w834:u16[])
                    }
                  }
                  n582 = local write "MTrig_Solenoid_trig__L"(w813) -> ()
                  n583 = local write "MTrig_Solenoid_trig__R"(w813) -> ()
                }
              }
              n584 = local read "get_countPerMS"() -> (w722:bool)
              n585 = Select(t=myRIO_BRig_RT__Case_NonExp_stateList."Get_FPGA_count_per_ms" ("Enum"), s=w722, f=myRIO_BRig_RT__Case_NonExp_stateList."Idle_6" ("Enum")) -> (s? t:f=w720:T1)
              n586 = Select(t=myRIO_BRig_RT__Case_NonExp_stateList."Cue_pre", s=w727, f=myRIO_BRig_RT__Case_NonExp_stateList."DispenseWater_pre" ("Enum")) -> (s? t:f=w725:T1)
              n587 = Select(t=w725, s=w729, f=w720) -> (s? t:f=w730:T1)
            }
            frame "Idle_5" {
              w858 = u8 0 ("f")
              # "There are a number of tasks we need to perform\nwhile idling. To preserve our timing loop, we\nbreak up the IDLE state into smaller states"
              n588 = local read "MTrig_Solenoid_trig__L"() -> (w849:bool)
              n589 = local read "MTrig_Solenoid_trig__R"() -> (w859:bool)
              n590 = local read "warmupType"() -> (w837:u8)
              n591 = local read "Cue1Param_CueType_Switch"() -> (w836:u16)
              n592 = local read "warmup"() -> (w851:bool)
              n593 = Not Equal To 0?(x=w837) -> (x != 0?=w842:bool)
              n594 = Not(x=w842) -> (.not. x?=w852:bool)
              n595 = Select(t=u8 1, s=w849, f=w858) -> (s? t:f=w857:u8)
              n596 = Select(t=u8 2, s=w859, f=w858) -> (s? t:f=w856:u8)
              n597 = And(x=w851, y=w852) -> (x .and. y?=w850:bool)
              n598 = And(x=w851, y=w842) -> (x .and. y?=w845:bool)
              n599 = Add(x=w857, y=w856) -> (x+y=w855:u8)
              n600 = case shown="2" w855 {
                tunnel: w854 -> [w862 w867 w916 w966]
                tunnel: [w862 w866 w915 w965] -> w853
                tunnel: w850 -> [_ w865 w914 w964]
                tunnel: [_ TRUE TRUE TRUE] -> w847
                tunnel: w836 -> [_ w863 w912 w962]
                frame 0, Default {
                }
                frame 1 {
                  n601 = case shown="True" w865 {
                    tunnel: w867 -> [w872 w911]
                    tunnel: [w871 w910] -> w866
                    tunnel: w863 -> [w870 _]
                    frame True {
                      n602 = case shown="0, Default" w870 {
                        tunnel: [TRUE _ w904] -> w869
                        frame 0, Default {
                          # "Audio"
                        }
                        frame 1 {
                          # "LED"
                        }
                        frame 2 {
                          # "Audio or LED"
                          n603 = local read "Cue1Param_AudioLed_Probability_Switch"() -> (w906:u16)
                          n604 = call "myRIO__convert__Probability_to_TrueFalse.vi"("input_probability_u16"=w906) -> ("output_TF"=w905:bool)  [unwired: 10 in]
                          n605 = Not(x=w905) -> (.not. x?=w904:bool)
                        }
                      }
                      n606 = case shown="True" w869 {
                        tunnel: w872 -> [w884 w902]
                        tunnel: [w883 w901] -> w871
                        frame True {
                          n607 = call "myRIO_BRig_RT_dataMTrig_Solenoid_N__L.vi"() -> ("output_Solenoid_N__L"=w881:i32)  [unwired: 11 in]
                          n608 = call "myRIO_BRig_RT_dataMTrig_Audio_N__L.vi"() -> ("output_Audio_N__L"=w879:i32)  [unwired: 11 in]
                          n609 = call "myRIO_BRig_RT_dataMTrig_Audio_N__R.vi"() -> ("output_Audio_N__R"=w874:i32)  [unwired: 11 in]
                          n610 = local read "sp_LeftSpout"() -> (w878:u16)
                          n611 = Index Array(array=w884, index #1=w881, index #2=w879, index #3=w874) -> (element #1=w882:u16, element #2=w877:u16, element #3=w876:u16)
                          n612 = case shown="2" w878 {
                            tunnel: w877 -> [w887 w890 w892]
                            tunnel: w876 -> [w885 w889 w894]
                            tunnel: [w886 w890 w891] -> w875
                            tunnel: [w885 w888 w893] -> w873
                            frame 0, Default {
                              n613 = Increment(x=w887) -> (x+1=w886:u16)
                            }
                            frame 1 {
                              n614 = Increment(x=w889) -> (x+1=w888:u16)
                            }
                            frame 2 {
                              n615 = Increment(x=w894) -> (x+1=w893:u16)
                              n616 = Increment(x=w892) -> (x+1=w891:u16)
                            }
                          }
                          n617 = Increment(x=w882) -> (x+1=w880:u16)
                          n618 = Replace Array Subset(array=w884, new element #1=w880, index #1=w881, new element #2=w875, index #2=w879, new element #3=w873, index #3=w874) -> (w883:u16[])
                        }
                        frame False {
                          n619 = call "myRIO_BRig_RT_dataMTrig_Solenoid_N__L.vi"() -> ("output_Solenoid_N__L"=w899:i32)  [unwired: 11 in]
                          n620 = call "myRIO_BRig_RT_dataMTrig_CueLed_N.vi"() -> ("output_CueLed_N"=w897:i32)  [unwired: 11 in]
                          n621 = Index Array(array=w902, index #1=w899, index #2=w897) -> (element #1=w900:u16, element #2=w896:u16)
                          n622 = Increment(x=w900) -> (x+1=w898:u16)
                          n623 = Increment(x=w896) -> (x+1=w895:u16)
                          n624 = Replace Array Subset(array=w902, new element #1=w898, index #1=w899, new element #2=w895, index #2=w897) -> (w901:u16[])
                        }
                      }
                    }
                    frame False {
                      # "Solenoid_L"
                      n625 = call "myRIO_BRig_RT_dataMTrig_Solenoid_N__L.vi"() -> ("output_Solenoid_N__L"=w908:i32)  [unwired: 11 in]
                      n626 = Index Array(array=w911, index=w908) -> (element=w909:u16)
                      n627 = Increment(x=w909) -> (x+1=w907:u16)
                      n628 = Replace Array Subset(array=w911, new element=w907, index=w908) -> (w910:u16[])
                    }
                  }
                  n629 = local write "MTrig_Solenoid_trig__L"(FALSE) -> ()
                }
                frame 2 {
                  n630 = case shown="True" w914 {
                    tunnel: w916 -> [w921 w960]
                    tunnel: [w920 w959] -> w915
                    tunnel: w912 -> [w919 _]
                    frame True {
                      n631 = case shown="0, Default" w919 {
                        tunnel: [TRUE _ w953] -> w918
                        frame 0, Default {
                          # "Audio"
                        }
                        frame 1 {
                          # "LED"
                        }
                        frame 2 {
                          # "Audio or LED"
                          n632 = local read "Cue1Param_AudioLed_Probability_Switch"() -> (w955:u16)
                          n633 = call "myRIO__convert__Probability_to_TrueFalse.vi"("input_probability_u16"=w955) -> ("output_TF"=w954:bool)  [unwired: 10 in]
                          n634 = Not(x=w954) -> (.not. x?=w953:bool)
                        }
                      }
                      n635 = case shown="True" w918 {
                        tunnel: w921 -> [w933 w951]
                        tunnel: [w932 w950] -> w920
                        frame True {
                          n636 = call "myRIO_BRig_RT_dataMTrig_Solenoid_N__R.vi"() -> ("output_Solenoid_N__R"=w930:i32)  [unwired: 11 in]
                          n637 = call "myRIO_BRig_RT_dataMTrig_Audio_N__L.vi"() -> ("output_Audio_N__L"=w928:i32)  [unwired: 11 in]
                          n638 = call "myRIO_BRig_RT_dataMTrig_Audio_N__R.vi"() -> ("output_Audio_N__R"=w923:i32)  [unwired: 11 in]
                          n639 = local read "sp_RightSpout"() -> (w927:u16)
                          n640 = Index Array(array=w933, index #1=w930, index #2=w928, index #3=w923) -> (element #1=w931:u16, element #2=w926:u16, element #3=w925:u16)
                          n641 = case shown="2" w927 {
                            tunnel: w926 -> [w936 w939 w941]
                            tunnel: w925 -> [w934 w938 w943]
                            tunnel: [w935 w939 w940] -> w924
                            tunnel: [w934 w937 w942] -> w922
                            frame 0, Default {
                              n642 = Increment(x=w936) -> (x+1=w935:u16)
                            }
                            frame 1 {
                              n643 = Increment(x=w938) -> (x+1=w937:u16)
                            }
                            frame 2 {
                              n644 = Increment(x=w943) -> (x+1=w942:u16)
                              n645 = Increment(x=w941) -> (x+1=w940:u16)
                            }
                          }
                          n646 = Increment(x=w931) -> (x+1=w929:u16)
                          n647 = Replace Array Subset(array=w933, new element #1=w929, index #1=w930, new element #2=w924, index #2=w928, new element #3=w922, index #3=w923) -> (w932:u16[])
                        }
                        frame False {
                          n648 = call "myRIO_BRig_RT_dataMTrig_Solenoid_N__R.vi"() -> ("output_Solenoid_N__R"=w948:i32)  [unwired: 11 in]
                          n649 = call "myRIO_BRig_RT_dataMTrig_CueLed_N.vi"() -> ("output_CueLed_N"=w946:i32)  [unwired: 11 in]
                          n650 = Index Array(array=w951, index #1=w948, index #2=w946) -> (element #1=w949:u16, element #2=w945:u16)
                          n651 = Increment(x=w949) -> (x+1=w947:u16)
                          n652 = Increment(x=w945) -> (x+1=w944:u16)
                          n653 = Replace Array Subset(array=w951, new element #1=w947, index #1=w948, new element #2=w944, index #2=w946) -> (w950:u16[])
                        }
                      }
                    }
                    frame False {
                      # "Solenoid_R"
                      n654 = call "myRIO_BRig_RT_dataMTrig_Solenoid_N__R.vi"() -> ("output_Solenoid_N__R"=w957:i32)  [unwired: 11 in]
                      n655 = Index Array(array=w960, index=w957) -> (element=w958:u16)
                      n656 = Increment(x=w958) -> (x+1=w956:u16)
                      n657 = Replace Array Subset(array=w960, new element=w956, index=w957) -> (w959:u16[])
                    }
                  }
                  n658 = local write "MTrig_Solenoid_trig__R"(FALSE) -> ()
                }
                frame 3 {
                  w961 = FALSE
                  n659 = case shown="True" w964 {
                    tunnel: w966 -> [w970 w1007]
                    tunnel: [w969 w1006] -> w965
                    tunnel: w962 -> [w968 _]
                    frame True {
                      n660 = case shown="2" w968 {
                        tunnel: [TRUE _ w997] -> w967
                        frame 0, Default {
                          # "Audio"
                        }
                        frame 1 {
                          # "LED"
                        }
                        frame 2 {
                          # "Audio or LED"
                          n661 = local read "Cue1Param_AudioLed_Probability_Switch"() -> (w999:u16)
                          n662 = call "myRIO__convert__Probability_to_TrueFalse.vi"("input_probability_u16"=w999) -> ("output_TF"=w998:bool)  [unwired: 10 in]
                          n663 = Not(x=w998) -> (.not. x?=w997:bool)
                        }
                      }
                      n664 = case shown="True" w967 {
                        tunnel: w970 -> [w984 w995]
                        tunnel: [w983 w994] -> w969
                        frame True {
                          n665 = call "myRIO_BRig_RT_dataMTrig_Solenoid_N__L.vi"() -> ("output_Solenoid_N__L"=w972:i32)  [unwired: 11 in]
                          n666 = call "myRIO_BRig_RT_dataMTrig_Solenoid_N__R.vi"() -> ("output_Solenoid_N__R"=w981:i32)  [unwired: 11 in]
                          n667 = call "myRIO_BRig_RT_dataMTrig_Audio_N__L.vi"() -> ("output_Audio_N__L"=w979:i32)  [unwired: 11 in]
                          n668 = call "myRIO_BRig_RT_dataMTrig_Audio_N__R.vi"() -> ("output_Audio_N__R"=w975:i32)  [unwired: 11 in]
                          n669 = Index Array(array=w984, index #1=w972, index #2=w981, index #3=w979, index #4=w975) -> (element #1=w973:u16, element #2=w982:u16, element #3=w978:u16, element #4=w977:u16)
                          n670 = Increment(x=w973) -> (x+1=w971:u16)
                          n671 = Increment(x=w982) -> (x+1=w980:u16)
                          n672 = Increment(x=w977) -> (x+1=w974:u16)
                          n673 = Increment(x=w978) -> (x+1=w976:u16)
                          n674 = Replace Array Subset(array=w984, new element #1=w971, index #1=w972, new element #2=w980, index #2=w981, new element #3=w976, index #3=w979, new element #4=w974, index #4=w975) -> (w983:u16[])
                        }
                        frame False {
                          n675 = call "myRIO_BRig_RT_dataMTrig_Solenoid_N__L.vi"() -> ("output_Solenoid_N__L"=w985:i32)  [unwired: 11 in]
                          n676 = call "myRIO_BRig_RT_dataMTrig_Solenoid_N__R.vi"() -> ("output_Solenoid_N__R"=w992:i32)  [unwired: 11 in]
                          n677 = call "myRIO_BRig_RT_dataMTrig_CueLed_N.vi"() -> ("output_CueLed_N"=w990:i32)  [unwired: 11 in]
                          n678 = Index Array(array=w995, index #1=w985, index #2=w992, index #3=w990) -> (element #1=w987:u16, element #2=w993:u16, element #3=w989:u16)
                          n679 = Increment(x=w987) -> (x+1=w986:u16)
                          n680 = Increment(x=w993) -> (x+1=w991:u16)
                          n681 = Increment(x=w989) -> (x+1=w988:u16)
                          n682 = Replace Array Subset(array=w995, new element #1=w986, index #1=w985, new element #2=w991, index #2=w992, new element #3=w988, index #3=w990) -> (w994:u16[])
                        }
                      }
                    }
                    frame False {
                      n683 = call "myRIO_BRig_RT_dataMTrig_Solenoid_N__L.vi"() -> ("output_Solenoid_N__L"=w1003:i32)  [unwired: 11 in]
                      n684 = call "myRIO_BRig_RT_dataMTrig_Solenoid_N__R.vi"() -> ("output_Solenoid_N__R"=w1002:i32)  [unwired: 11 in]
                      n685 = Index Array(array=w1007, index #1=w1003, index #2=w1002) -> (element #1=w1005:u16, element #2=w1001:u16)
                      n686 = Increment(x=w1001) -> (x+1=w1000:u16)
                      n687 = Increment(x=w1005) -> (x+1=w1004:u16)
                      n688 = Replace Array Subset(array=w1007, new element #1=w1004, index #1=w1003, new element #2=w1000, index #2=w1002) -> (w1006:u16[])
                    }
                  }
                  n689 = local write "MTrig_Solenoid_trig__L"(w961) -> ()
                  n690 = local write "MTrig_Solenoid_trig__R"(w961) -> ()
                }
              }
              n691 = local read "get_countPerMS"() -> (w841:bool)
              n692 = Select(t=myRIO_BRig_RT__Case_NonExp_stateList."Get_FPGA_count_per_ms" ("Enum"), s=w841, f=myRIO_BRig_RT__Case_NonExp_stateList."Idle_6" ("Enum")) -> (s? t:f=w839:T1)
              n693 = Select(t=myRIO_BRig_RT__Case_NonExp_stateList."Cue_pre", s=w845, f=myRIO_BRig_RT__Case_NonExp_stateList."DispenseWater_pre" ("Enum")) -> (s? t:f=w843:T1)
              n694 = Select(t=w843, s=w847, f=w839) -> (s? t:f=w848:T1)
            }
            frame "Idle_6" {
              # "There are a number of tasks we need to perform\nwhile idling. To preserve our timing loop, we\nbreak up the IDLE state into smaller states"
              # "use dataMTrig as it is one of the last to transfer"
              n695 = call "myRIO_BRig_RT_comm_webdav_uploadReceived_check_v2,0.vi"("input_dataName"="dataMTrig") -> ("output_Iexist"=w1012:bool)  [unwired: 9 in, 1 out]
              n696 = Select(t=myRIO_BRig_RT__Case_NonExp_stateList."UploadSettings_pre" ("Enum"), s=w1012, f=myRIO_BRig_RT__Case_NonExp_stateList."Idle") -> (s? t:f=w1010:T1)
            }
            frame "Cue_pre" {
              w1019 = u16 0 ("new element/subarray")
              # "Audio cue or LED cue?"
              # "Audio, LED, or \"Audio or LED\""
              # "Right Audio?"
              # "Left Audio?"
              # "Left or Right?"
              # "Cue Audio?\n(T=Audio, F=LED)"
              # "Ncycle"
              # "count"
              # "Audio_R"
              # "Ncycle"
              # "count"
              # "Audio_L"
              n697 = local read "Cue1Param_CueType_Switch"() -> (w1043:u16)
              n698 = case shown="2" w1043 {
                tunnel: [TRUE _ w1061] -> w1015
                frame 0, Default {
                  # "Audio"
                }
                frame 1 {
                  # "LED"
                }
                frame 2 {
                  # "Audio or LED"
                  n699 = local read "Cue1Param_AudioLed_Probability_Switch"() -> (w1063:u16)
                  n700 = call "myRIO__convert__Probability_to_TrueFalse.vi"("input_probability_u16"=w1063) -> ("output_TF"=w1062:bool)  [unwired: 10 in]
                  n701 = Not(x=w1062) -> (.not. x?=w1061:bool)
                }
              }
              n702 = call "myRIO_BRig_RT_dataMTrig_Solenoid_N__L.vi"() -> ("output_Solenoid_N__L"=w1053:i32)  [unwired: 11 in]
              n703 = call "myRIO_BRig_RT_dataMTrig_Solenoid_N__R.vi"() -> ("output_Solenoid_N__R"=w1052:i32)  [unwired: 11 in]
              n704 = Index Array(array=w1049, index #1=w1053, index #2=w1052) -> (element #1=w1051:u16, element #2=w1050:u16)
              n705 = Not Equal To 0?(x=w1051) -> (x != 0?=w1039:bool)
              n706 = Not Equal To 0?(x=w1050) -> (x != 0?=w1038:bool)
              n707 = Not(x=w1015) -> (.not. x?=w1014:bool)
              n708 = And(x=w1015, y=w1039) -> (x .and. y?=w1033:bool)
              n709 = And(x=w1015, y=w1038) -> (x .and. y?=w1031:bool)
              n710 = Select(t=myRIO_BRig_RT__Case_NonExp_stateList."Cue", s=w1015, f=myRIO_BRig_RT__Case_NonExp_stateList."Cue") -> (s? t:f=w1041:T1)
              n711 = local read "sp_RightSpout"() -> (w1032:u16)
              n712 = local read "sp_LeftSpout"() -> (w1034:u16)
              n713 = Boolean To (0,1)(Boolean=w1014) -> (0, 1=w1017:i16)
              n714 = To Unsigned Word Integer(number=w1017) -> (unsigned 16bit integer=w1016:u16)
              n715 = case shown="0, Default" w1034 {
                tunnel: [w1057 _ w1059] -> w1030
                tunnel: [_ w1058 w1059] -> w1028
                tunnel: w1033 -> [w1057 w1058 w1059]
                frame 0, Default {
                }
                frame 1 {
                }
                frame 2 {
                }
              }
              n716 = case shown="0, Default" w1032 {
                tunnel: [w1054 _ w1056] -> w1029
                tunnel: [_ w1055 w1056] -> w1027
                tunnel: w1031 -> [w1054 w1055 w1056]
                frame 0, Default {
                }
                frame 1 {
                }
                frame 2 {
                }
              }
              n717 = call "myRIO_BRig_RT_dataMTrig_Audio_c__L.vi"() -> ("output_Audio_c__L"=w1047:i32)  [unwired: 11 in]
              n718 = call "myRIO_BRig_RT_dataMTrig_Audio_N__L.vi"() -> ("output_Audio_N__L"=w1046:i32)  [unwired: 11 in]
              n719 = call "myRIO_BRig_RT_dataMTrig_Audio_c__R.vi"() -> ("output_Audio_c__R"=w1045:i32)  [unwired: 11 in]
              n720 = call "myRIO_BRig_RT_dataMTrig_Audio_N__R.vi"() -> ("output_Audio_N__R"=w1044:i32)  [unwired: 11 in]
              n721 = call "myRIO_BRig_RT_dataMTrig_CueLed_c.vi"() -> ("output_CueLed_c"=w1020:i32)  [unwired: 11 in]
              n722 = call "myRIO_BRig_RT_dataMTrig_CueLed_N.vi"() -> ("output_CueLed_N"=w1018:i32)  [unwired: 11 in]
              n723 = Or(x=w1030, y=w1029) -> (x .or. y?=w1026:bool)
              n724 = Boolean To (0,1)(Boolean=w1026) -> (0, 1=w1024:i16)
              n725 = To Unsigned Word Integer(number=w1024) -> (unsigned 16bit integer=w1023:u16)
              n726 = Or(x=w1028, y=w1027) -> (x .or. y?=w1025:bool)
              n727 = Boolean To (0,1)(Boolean=w1025) -> (0, 1=w1022:i16)
              n728 = To Unsigned Word Integer(number=w1022) -> (unsigned 16bit integer=w1021:u16)
              n729 = Replace Array Subset(array=w1049, new element #1=w1019, index #1=w1047, new element #2=w1023, index #2=w1046, new element #3=w1019, index #3=w1045, new element #4=w1021, index #4=w1044, new element #5=w1019, index #5=w1020, new element #6=w1016, index #6=w1018) -> (w1048:u16[])
              n730 = Initialize Array(u16 0 ("element"), 1 ("dimension size")) -> (w1037:u16[])
            }
            frame "Cue" {
              # "warmupType\n0 = Cue with reward (not possible to be in this state with value==0)\n1 = Cue then reward\n2 = Cue then reward (no lick)"
              # "Audio cue"
              # "lick did not occur or warmupType==1"
              # "lick occurred?"
              # "Ncycle"
              # "Audio_R"
              # "Ncycle"
              # "Audio_L"
              n731 = local read "warmupType"() -> (w1073:u8)
              n732 = Greater?(x=w1079, y=w1078) -> (0:w1082:bool)
              n733 = Greater?(x=w1081, y=w1080) -> (0:w1077:bool)
              n734 = Or(x=w1077, y=w1082) -> (x .or. y?=w1071:bool)
              n735 = Equal?(x=w1073, y=u8 1) -> (x = y?=w1067:bool)
              n736 = Not(x=w1071) -> (.not. x?=w1070:bool)
              n737 = call "myRIO_BRig_RT_dataMTrig_Audio_N__L.vi"() -> ("output_Audio_N__L"=w1084:i32)  [unwired: 11 in]
              n738 = call "myRIO_BRig_RT_dataMTrig_Audio_N__R.vi"() -> ("output_Audio_N__R"=w1083:i32)  [unwired: 11 in]
              n739 = call "myRIO_BRig_RT_dataMTrig_CueLed_N.vi"() -> ("output_CueLed_N"=w1064:i32)  [unwired: 11 in]
              n740 = Or(x=w1070, y=w1067) -> (x .or. y?=w1068:bool)
              n741 = case shown="True" w1068 {
                tunnel: w1084 -> [w1090 w1111]
                tunnel: w1083 -> [w1089 w1110]
                tunnel: w1076 -> [w1092 w1105]
                tunnel: [w1091 w1105] -> w1075
                tunnel: w1074 -> [_ w1103]
                tunnel: [myRIO_BRig_RT__Case_NonExp_stateList."Idle" ("t") w1102] -> w1069
                tunnel: w1067 -> [_ w1101]
                tunnel: w1066 -> [_ w1097]
                tunnel: w1065 -> [_ w1096]
                tunnel: w1064 -> [_ w1095]
                frame False {
                  w1085 = u16 0 ("new element/subarray")
                  # "lick occurred and warmupType==2"
                  n742 = call "myRIO_BRig_RT_dataMTrig_Solenoid_N__R.vi"() -> ("output_Solenoid_N__R"=w1086:i32)  [unwired: 11 in]
                  n743 = call "myRIO_BRig_RT_dataMTrig_Solenoid_N__L.vi"() -> ("output_Solenoid_N__L"=w1087:i32)  [unwired: 11 in]
                  n744 = Replace Array Subset(array=w1092, new element #1=w1085, index #1=w1090, new element #2=w1085, index #2=w1089, new element #3=w1085, index #3=w1087, new element #4=w1085, index #4=w1086) -> (w1091:u16[])
                }
                frame True {
                  n745 = Not(x=w1101) -> (.not. x?=w1100:bool)
                  n746 = Index Array(array=w1105, index #1=w1111, index #2=w1110, index #3=w1095) -> (element #1=w1109:u16, element #2=w1108:u16, element #3=w1094:u16)
                  n747 = Equal To 0?(x=w1109) -> (x = 0?=w1107:bool)
                  n748 = Equal To 0?(x=w1108) -> (x = 0?=w1106:bool)
                  n749 = Equal To 0?(x=w1094) -> (x = 0?=w1093:bool)
                  n750 = Compound Arithmetic op=AND(w1107, w1106, w1093) -> (w1099:bool)
                  n751 = And(x=w1099, y=w1100) -> (x .and. y?=w1098:bool)
                  n752 = case shown="True" w1098 {
                    tunnel: w1097 -> [_ w1119]
                    tunnel: w1096 -> [_ w1114]
                    frame False {
                    }
                    frame True {
                      n753 = local read "count_warmup_R"() -> (w1112:u16)
                      n754 = local read "count_warmup_L"() -> (w1117:u16)
                      n755 = Increment(x=w1112) -> (x+1=w1115:u16)
                      n756 = Increment(x=w1117) -> (x+1=w1118:u16)
                      n757 = Select(t=w1115, s=w1114, f=w1112) -> (s? t:f=w1113:u16)
                      n758 = Select(t=w1118, s=w1119, f=w1117) -> (s? t:f=w1116:u16)
                      n759 = local write "count_warmup_R"(w1113) -> ()
                      n760 = local write "count_warmup_L"(w1116) -> ()
                    }
                  }
                  n761 = Select(t=myRIO_BRig_RT__Case_NonExp_stateList."DispenseWater_pre", s=w1099, f=w1103) -> (s? t:f=w1102:T1)
                }
              }
            }
            frame "Cue_LED" {
              # "LED Cue"
              # "lick did not occur or warmupType==1"
              # "lick occurred?"
              n762 = local read "warmupType"() -> (w1132:u8)
              n763 = Greater?(x=w1138, y=w1137) -> (0:w1141:bool)
              n764 = Greater?(x=w1140, y=w1139) -> (0:w1136:bool)
              n765 = Or(x=w1136, y=w1141) -> (x .or. y?=w1130:bool)
              n766 = Equal?(x=w1132, y=u8 1) -> (x = y?=w1126:bool)
              n767 = Not(x=w1130) -> (.not. x?=w1129:bool)
              n768 = Or(x=w1129, y=w1126) -> (x .or. y?=w1127:bool)
              n769 = case shown="True" w1127 {
                tunnel: w1135 -> [w1148 w1168]
                tunnel: [w1147 w1168] -> w1134
                tunnel: w1133 -> [_ w1154]
                tunnel: [myRIO_BRig_RT__Case_NonExp_stateList."Idle" ("t") w1167] -> w1128
                tunnel: w1126 -> [_ w1153]
                tunnel: w1125 -> [_ w1165]
                tunnel: w1124 -> [_ w1164]
                tunnel: w1123 -> [w1142 w1163]
                tunnel: [w1142 w1156] -> w1122
                tunnel: w1121 -> [_ w1151]
                tunnel: w1120 -> [_ w1150]
                frame False {
                  w1143 = u16 0 ("new element/subarray")
                  # "lick occurred and warmupType==2"
                  n770 = call "myRIO_BRig_RT_dataMTrig_Solenoid_N__R.vi"() -> ("output_Solenoid_N__R"=w1144:i32)  [unwired: 11 in]
                  n771 = call "myRIO_BRig_RT_dataMTrig_Solenoid_N__L.vi"() -> ("output_Solenoid_N__L"=w1145:i32)  [unwired: 11 in]
                  n772 = Replace Array Subset(array=w1148, new element #1=w1143, new element #2=w1143, index #2=w1145, new element #3=w1143, index #3=w1144) -> (w1147:u16[])  [unwired: 1 in]
                }
                frame True {
                  w1161 = 0 ("index")
                  n773 = local read "Tcycle_Cue_LED_min"() -> (w1157:u16)
                  n774 = Index Array(array=w1163, index=w1161) -> (element=w1162:u16)
                  n775 = Increment(x=w1162) -> (x+1=w1160:u16)
                  n776 = Multiply(x=w1160, y=u16 5) -> (x*y=w1158:u16)
                  n777 = Replace Array Subset(array=w1163, new element=w1160, index=w1161) -> (w1156:u16[])
                  n778 = Less?(x=w1158, y=w1157) -> (x < y?=w1152:bool)
                  n779 = Not Or(1:w1153, 2:w1152) -> (0:w1166:bool)
                  n780 = case shown="True" w1166 {
                    tunnel: w1165 -> [_ w1176]
                    tunnel: w1164 -> [_ w1171]
                    frame False {
                    }
                    frame True {
                      n781 = local read "count_warmup_R"() -> (w1169:u16)
                      n782 = local read "count_warmup_L"() -> (w1174:u16)
                      n783 = Increment(x=w1169) -> (x+1=w1172:u16)
                      n784 = Increment(x=w1174) -> (x+1=w1175:u16)
                      n785 = Select(t=w1172, s=w1171, f=w1169) -> (s? t:f=w1170:u16)
                      n786 = Select(t=w1175, s=w1176, f=w1174) -> (s? t:f=w1173:u16)
                      n787 = local write "count_warmup_R"(w1170) -> ()
                      n788 = local write "count_warmup_L"(w1173) -> ()
                    }
                  }
                  n789 = Select(t=w1154, s=w1152, f=myRIO_BRig_RT__Case_NonExp_stateList."DispenseWater_pre" ("t")) -> (s? t:f=w1167:T1)
                  n790 = xnode "Read/Write Control"("FPGA VI Reference In"=w1151, "error in"=w1150, "CueLed_Event"=w1152) -> ("error out"=w1149:errorcluster)  [unwired: 1 out]
                  n791 = local write "error out"(w1149) -> ()
                }
              }
            }
            frame "RewardCalibration_pre" {
              (unwired) FALSE
              w1177 = FALSE
              w1188 = u8 0
              w1204 = u8 0
              # "Are we starting a RewardCalibration?\nOr are we stopping a RewardCalibration?\nOr is a RewardCalibration over?"
              # "RewCalib\nOnOff"
              # "N"
              # "Solenoid R"
              # "RewCalib\nOnOff"
              # "N"
              # "Solenoid L"
              n792 = local read "RewCalib_Trig_L"() -> (w1211:bool)
              n793 = local read "RewCalib_Trig_R"() -> (w1180:bool)
              n794 = call "myRIO_BRig_RT_dataMTrig_Solenoid_N__R.vi"() -> ("output_Solenoid_N__R"=w1182:i32)  [unwired: 11 in]
              n795 = call "myRIO_BRig_RT_dataMTrig_Solenoid_RewCalib_OnOff__R.vi"() -> ("output_Solenoid_RewCalib_OnOff__R"=w1179:i32)  [unwired: 11 in]
              n796 = call "myRIO_BRig_RT_dataMTrig_Solenoid_N__L.vi"() -> ("output_Solenoid_N__L"=w1197:i32)  [unwired: 11 in]
              n797 = call "myRIO_BRig_RT_dataMTrig_Solenoid_RewCalib_OnOff__L.vi"() -> ("output_Solenoid_RewCalib_OnOff__L"=w1198:i32)  [unwired: 11 in]
              n798 = Index Array(array=w1181, index #1=w1182, index #2=w1179) -> (element #1=w1192:u16, element #2=w1187:u16)
              n799 = Index Array(array=w1181, index #1=w1197, index #2=w1198) -> (element #1=w1208:u16, element #2=w1203:u16)
              n800 = Equal To 0?(x=w1192) -> (x = 0?=w1193:bool)
              n801 = Not Equal To 0?(x=w1187) -> (x != 0?=w1190:bool)
              n802 = Equal To 0?(x=w1208) -> (x = 0?=w1209:bool)
              n803 = Not Equal To 0?(x=w1203) -> (x != 0?=w1206:bool)
              n804 = local write "MTrig_Solenoid_trig__L"(w1177) -> ()
              n805 = local write "MTrig_Solenoid_trig__R"(w1177) -> ()
              n806 = Select(t=u8 1, s=w1180, f=w1188) -> (s? t:f=w1184:u8)
              n807 = Select(t=u8 1, s=w1211, f=w1204) -> (s? t:f=w1200:u8)
              n808 = Select(t=u8 2, s=w1193, f=w1188) -> (s? t:f=w1185:u8)
              n809 = Select(t=u8 4, s=w1190, f=w1188) -> (s? t:f=w1186:u8)
              n810 = Select(t=u8 2, s=w1209, f=w1204) -> (s? t:f=w1201:u8)
              n811 = Select(t=u8 4, s=w1206, f=w1204) -> (s? t:f=w1202:u8)
              n812 = Compound Arithmetic op=ADD(w1184, w1185, w1186) -> (w1183:u8)
              n813 = Compound Arithmetic op=ADD(w1200, w1201, w1202) -> (w1199:u8)
              n814 = case shown="7" w1199 {
                tunnel: w1181 -> [w1241 w1246 w1248 w1253 w1258 w1260 w1263 w1268]
                tunnel: [w1241 w1247 w1248 w1254 w1259 w1260 w1264 w1269] -> w1196
                tunnel: w1198 -> [_ w1244 _ w1251 w1256 _ w1262 w1267]
                tunnel: w1197 -> [_ w1245 _ w1252 w1257 _ _ _]
                frame 0, Default {
                }
                frame 1 {
                  n815 = Replace Array Subset(array=w1246, new element #1=u16 100 ("new element/subarray"), index #1=w1245, new element #2=u16 1 ("new element/subarray"), index #2=w1244) -> (w1247:u16[])
                }
                frame 2 {
                }
                frame 3 {
                  n816 = Replace Array Subset(array=w1253, new element #1=u16 100 ("new element/subarray"), index #1=w1252, new element #2=u16 1 ("new element/subarray"), index #2=w1251) -> (w1254:u16[])
                }
                frame 4 {
                  w1255 = u16 0 ("new element/subarray")
                  n817 = Replace Array Subset(array=w1258, new element #1=w1255, index #1=w1257, new element #2=w1255, index #2=w1256) -> (w1259:u16[])
                }
                frame 5 {
                }
                frame 6 {
                  n818 = Replace Array Subset(array=w1263, new element=u16 0 ("new element/subarray"), index=w1262) -> (w1264:u16[])
                }
                frame 7 {
                  n819 = local write "RewCalib_Trig_L"(FALSE ("RewCalib_Trig_L")) -> ()
                  n820 = Replace Array Subset(array=w1268, new element=u16 0 ("new element/subarray"), index=w1267) -> (w1269:u16[])
                }
              }
              n821 = case shown="7" w1183 {
                tunnel: w1196 -> [w1212 w1217 w1219 w1224 w1229 w1231 w1234 w1239]
                tunnel: [w1212 w1218 w1219 w1225 w1230 w1231 w1235 w1240] -> w1195
                tunnel: w1179 -> [_ w1215 _ w1222 w1227 _ w1233 w1238]
                tunnel: w1182 -> [_ w1216 _ w1223 w1228 _ _ _]
                frame 0, Default {
                }
                frame 1 {
                  n822 = Replace Array Subset(array=w1217, new element #1=u16 100 ("new element/subarray"), index #1=w1216, new element #2=u16 1 ("new element/subarray"), index #2=w1215) -> (w1218:u16[])
                }
                frame 2 {
                }
                frame 3 {
                  n823 = Replace Array Subset(array=w1224, new element #1=u16 100 ("new element/subarray"), index #1=w1223, new element #2=u16 1 ("new element/subarray"), index #2=w1222) -> (w1225:u16[])
                }
                frame 4 {
                  w1226 = u16 0 ("new element/subarray")
                  n824 = Replace Array Subset(array=w1229, new element #1=w1226, index #1=w1228, new element #2=w1226, index #2=w1227) -> (w1230:u16[])
                }
                frame 5 {
                }
                frame 6 {
                  n825 = Replace Array Subset(array=w1234, new element=u16 0 ("new element/subarray"), index=w1233) -> (w1235:u16[])
                }
                frame 7 {
                  n826 = local write "RewCalib_Trig_R"(FALSE ("RewCalib_Trig_L")) -> ()
                  n827 = Replace Array Subset(array=w1239, new element=u16 0 ("new element/subarray"), index=w1238) -> (w1240:u16[])
                }
              }
            }
            frame "DispenseWater_pre" {
              w1275 = u16 0 ("t")
              w1318 = u16 0 ("new element/subarray")
              # "just trust me on this one"
              # "RewCalib\nOnOff"
              # "RewCalib\nOnOff"
              # "nCycle"
              # "Solenoid__R"
              # "Tdelay"
              # "delay"
              # "nCycle"
              # "Solenoid__L"
              # "Tdelay"
              # "delay"
              # "Solenoid__R"
              # "count"
              # "Solenoid_Tcycle_R"
              # "Solenoid_Tcycle_L"
              # "Solenoid__L"
              # "count"
              n828 = call "myRIO_BRig_RT_dataMTrig_Solenoid_RewCalib_OnOff__L.vi"() -> ("output_Solenoid_RewCalib_OnOff__L"=w1282:i32)  [unwired: 11 in]
              n829 = call "myRIO_BRig_RT_dataMTrig_Solenoid_N__L.vi"() -> ("output_Solenoid_N__L"=w1273:i32)  [unwired: 11 in]
              n830 = call "myRIO_BRig_RT_dataMTrig_Solenoid_delay__L.vi"() -> ("output_Solenoid_delay__L"=w1316:i32)  [unwired: 11 in]
              n831 = call "myRIO_BRig_RT_dataMTrig_Solenoid_Tdelay__L.vi"() -> ("output_Solenoid_Tdelay__L"=w1315:i32)  [unwired: 11 in]
              n832 = call "myRIO_BRig_RT_dataMTrig_Solenoid_N__R.vi"() -> ("output_Solenoid_N__R"=w1271:i32)  [unwired: 11 in]
              n833 = call "myRIO_BRig_RT_dataMTrig_Solenoid_delay__R.vi"() -> ("output_Solenoid_delay__R"=w1305:i32)  [unwired: 11 in]
              n834 = call "myRIO_BRig_RT_dataMTrig_Solenoid_Tdelay__R.vi"() -> ("output_Solenoid_Tdelay__R"=w1304:i32)  [unwired: 11 in]
              n835 = call "myRIO_BRig_RT_dataMTrig_Solenoid_RewCalib_OnOff__R.vi"() -> ("output_Solenoid_RewCalib_OnOff__R"=w1278:i32)  [unwired: 11 in]
              n836 = Index Array(array=w1317, index #1=w1273, index #2=w1316, index #3=w1315, index #4=w1271, index #5=w1305, index #6=w1304, index #7=w1282, index #8=w1278) -> (element #1=w1274:u16, element #2=w1314:u16, element #3=w1309:u16, element #4=w1277:u16, element #5=w1299:u16, element #6=w1298:u16, element #7=w1283:u16, element #8=w1280:u16)
              n837 = Equal To 0?(x=w1314) -> (x = 0?=w1313:bool)
              n838 = Equal To 0?(x=w1299) -> (x = 0?=w1303:bool)
              n839 = local read "RewCalib_Trig_L"() -> (w1294:bool)
              n840 = local read "RewCalib_Trig_R"() -> (w1289:bool)
              n841 = Not Equal To 0?(x=w1274) -> (x != 0?=w1312:bool)
              n842 = Not Equal To 0?(x=w1277) -> (x != 0?=w1302:bool)
              n843 = local read "MTrig_Solenoid_Tcycle__L"() -> (w1311:u16)
              n844 = local read "MTrig_Solenoid_Tcycle__R"() -> (w1297:u16)
              n845 = Not Equal To 0?(x=w1283) -> (x != 0?=w1293:bool)
              n846 = Not Equal To 0?(x=w1280) -> (x != 0?=w1291:bool)
              n847 = Not(x=w1294) -> (.not. x?=w1292:bool)
              n848 = Not(x=w1289) -> (.not. x?=w1290:bool)
              n849 = And(x=w1293, y=w1292) -> (x .and. y?=w1288:bool)
              n850 = And(x=w1291, y=w1290) -> (x .and. y?=w1287:bool)
              n851 = call "myRIO_BRig_RT_dataMTrig_Solenoid_c__L.vi"() -> ("output_Solenoid_c__L"=w1320:i32)  [unwired: 11 in]
              n852 = call "myRIO_BRig_RT_dataMTrig_Solenoid_c__R.vi"() -> ("output_Solenoid_c__R"=w1319:i32)  [unwired: 11 in]
              n853 = Select(t=w1311, s=w1312, f=u16 0) -> (s? t:f=w1308:u16)
              n854 = Or(x=w1288, y=w1287) -> (x .or. y?=w1276:bool)
              n855 = Select(t=w1297, s=w1302, f=u16 0) -> (s? t:f=w1300:u16)
              n856 = Select(t=w1308, s=w1313, f=w1309) -> (s? t:f=w1306:u16)
              n857 = Select(t=w1300, s=w1303, f=w1298) -> (s? t:f=w1295:u16)
              n858 = call "myRIO_BRig_RT_dataMTrig_Solenoid_Tcycle__L.vi"() -> ("output_Solenoid_Tcycle__L"=w1307:i32)  [unwired: 11 in]
              n859 = call "myRIO_BRig_RT_dataMTrig_Solenoid_Tcycle__R.vi"() -> ("output_Solenoid_Tcycle__R"=w1296:i32)  [unwired: 11 in]
              n860 = Select(t=w1275, s=w1276, f=w1274) -> (s? t:f=w1272:u16)
              n861 = Select(t=w1275, s=w1276, f=w1277) -> (s? t:f=w1270:u16)
              n862 = Select(t=myRIO_BRig_RT__Case_NonExp_stateList."Idle" ("Enum"), s=w1276, f=myRIO_BRig_RT__Case_NonExp_stateList."DispenseWater" ("Enum")) -> (s? t:f=w1284:T1)
              n863 = Select(t=w1275, s=w1276, f=w1283) -> (s? t:f=w1281:u16)
              n864 = Select(t=w1275, s=w1276, f=w1280) -> (s? t:f=w1279:u16)
              n865 = Replace Array Subset(array=w1317, new element #1=w1318, index #1=w1320, new element #2=w1318, index #2=w1319, new element #3=w1306, index #3=w1307, new element #4=w1295, index #4=w1296, new element #5=w1281, index #5=w1282, new element #6=w1279, index #6=w1278, new element #7=w1272, index #7=w1273, new element #8=w1270, index #8=w1271) -> (w1321:u16[])
            }
            frame "DispenseWater" {
              # "D"
              # "C"
              # "B"
              # "A"
              # "(A) Add COUNT and INCREMENT\n(B) Is (A) smaller than Tcycle?\n(C) Are we dispensing water or in the delay phase?\n(D) If (A) is smaller than Tcycle   AND   if we are dispensing water\n      then send TRUE to solenoid"
              # "delay"
              # "Tcycle"
              # "Solenoid__R"
              # "count"
              # "delay"
              # "Tcycle"
              # "Solenoid__L"
              # "count"
              n866 = To Unsigned Word Integer(number=w1348) -> (unsigned 16bit integer=w1330:u16)
              n867 = call "myRIO_BRig_RT_dataMTrig_Solenoid_delay__R.vi"() -> ("output_Solenoid_delay__R"=w1334:i32)  [unwired: 11 in]
              n868 = call "myRIO_BRig_RT_dataMTrig_Solenoid_c__R.vi"() -> ("output_Solenoid_c__R"=w1333:i32)  [unwired: 11 in]
              n869 = call "myRIO_BRig_RT_dataMTrig_Solenoid_Tcycle__R.vi"() -> ("output_Solenoid_Tcycle__R"=w1335:i32)  [unwired: 11 in]
              n870 = call "myRIO_BRig_RT_dataMTrig_Solenoid_delay__L.vi"() -> ("output_Solenoid_delay__L"=w1350:i32)  [unwired: 11 in]
              n871 = call "myRIO_BRig_RT_dataMTrig_Solenoid_c__L.vi"() -> ("output_Solenoid_c__L"=w1342:i32)  [unwired: 11 in]
              n872 = call "myRIO_BRig_RT_dataMTrig_Solenoid_Tcycle__L.vi"() -> ("output_Solenoid_Tcycle__L"=w1351:i32)  [unwired: 11 in]
              n873 = Index Array(array=w1344, index #1=w1342, index #2=w1351, index #3=w1350, index #4=w1333, index #5=w1335, index #6=w1334) -> (element #1=w1349:u16, element #2=w1339:u16, element #3=w1347:u16, element #4=w1329:u16, element #5=w1326:u16, element #6=w1325:u16)
              n874 = Add(x=w1349, y=w1330) -> (x+y=w1340:u16)
              n875 = Add(x=w1329, y=w1330) -> (x+y=w1331:u16)
              n876 = Less?(x=w1340, y=w1339) -> (x < y?=w1323:bool)
              n877 = Equal To 0?(x=w1347) -> (x = 0?=w1346:bool)
              n878 = Less?(x=w1331, y=w1326) -> (x < y?=w1324:bool)
              n879 = Equal To 0?(x=w1325) -> (x = 0?=w1332:bool)
              n880 = And(x=w1323, y=w1346) -> (x .and. y?=w1345:bool)
              n881 = Or(x=w1323, y=w1324) -> (x .or. y?=w1322:bool)
              n882 = And(x=w1324, y=w1332) -> (x .and. y?=w1327:bool)
              n883 = Select(t=w1340, s=w1323, f=w1339) -> (s? t:f=w1341:u16)
              n884 = Select(t=w1331, s=w1324, f=w1326) -> (s? t:f=w1328:u16)
              n885 = Replace Array Subset(array=w1344, new element #1=w1341, index #1=w1342, new element #2=w1328, index #2=w1333) -> (w1343:u16[])
              n886 = Select(t=w1338, s=w1322, f=myRIO_BRig_RT__Case_NonExp_stateList."DispenseWater_post" ("Enum")) -> (s? t:f=w1336:T1)
            }
            frame "DispenseWater_post" {
              # "nCycle"
              # "delay"
              # "Solenoid__R"
              # "nCycle"
              # "delay"
              # "Solenoid__L"
              n887 = call "myRIO_BRig_RT_dataMTrig_Solenoid_N__L.vi"() -> ("output_Solenoid_N__L"=w1368:i32)  [unwired: 11 in]
              n888 = call "myRIO_BRig_RT_dataMTrig_Solenoid_delay__L.vi"() -> ("output_Solenoid_delay__L"=w1367:i32)  [unwired: 11 in]
              n889 = call "myRIO_BRig_RT_dataMTrig_Solenoid_N__R.vi"() -> ("output_Solenoid_N__R"=w1364:i32)  [unwired: 11 in]
              n890 = call "myRIO_BRig_RT_dataMTrig_Solenoid_delay__R.vi"() -> ("output_Solenoid_delay__R"=w1363:i32)  [unwired: 11 in]
              n891 = Index Array(array=w1370, index #1=w1368, index #2=w1367, index #3=w1364, index #4=w1363) -> (element #1=w1372:u16, element #2=w1371:u16, element #3=w1355:u16, element #4=w1357:u16)
              n892 = Not Equal To 0?(x=w1372) -> (x != 0?=w1373:bool)
              n893 = Not Equal To 0?(x=w1355) -> (x != 0?=w1356:bool)
              n894 = case shown="True" w1356 {
                selector: w1356 -> [_ w1377]
                tunnel: w1355 -> [w1375 w1383]
                tunnel: w1357 -> [_ w1384]
                tunnel: [w1375 w1381] -> w1354
                tunnel: [u16 0 w1380] -> w1353
                tunnel: [_ w1377] -> w1352
                frame False {
                }
                frame True {
                  n895 = Equal To 0?(x=w1384) -> (x = 0?=w1376:bool)
                  n896 = Decrement(x=w1383) -> (x-1=w1382:u16)
                  n897 = Select(t=w1382, s=w1376, f=w1383) -> (s? t:f=w1381:u16)
                  n898 = Select(t=u16 1, s=w1376, f=u16 0) -> (s? t:f=w1380:u16)
                }
              }
              n899 = case shown="True" w1373 {
                selector: w1373 -> [_ w1388]
                tunnel: w1372 -> [w1386 w1394]
                tunnel: w1371 -> [_ w1395]
                tunnel: [w1386 w1392] -> w1366
                tunnel: [u16 0 w1391] -> w1365
                tunnel: [_ w1388] -> w1362
                frame False {
                }
                frame True {
                  n900 = Equal To 0?(x=w1395) -> (x = 0?=w1387:bool)
                  n901 = Decrement(x=w1394) -> (x-1=w1393:u16)
                  n902 = Select(t=w1393, s=w1387, f=w1394) -> (s? t:f=w1392:u16)
                  n903 = Select(t=u16 1, s=w1387, f=u16 0) -> (s? t:f=w1391:u16)
                }
              }
              n904 = Or(x=w1362, y=w1352) -> (x .or. y?=w1361:bool)
              n905 = Replace Array Subset(array=w1370, new element #1=w1366, index #1=w1368, new element #2=w1365, index #2=w1367, new element #3=w1354, index #3=w1364, new element #4=w1353, index #4=w1363) -> (w1369:u16[])
              n906 = Select(t=myRIO_BRig_RT__Case_NonExp_stateList."DispenseWater_pre" ("Enum"), s=w1361, f=myRIO_BRig_RT__Case_NonExp_stateList."Idle" ("Enum")) -> (s? t:f=w1358:T1)
            }
            frame "TestConnection" {
              n907 = local read "Host Password"() -> (w1401:string)
              n908 = local read "Host UserName"() -> (w1402:string)
              n909 = call "myRIO_BRig_RT_comm_webdav_testConnect.vi"("input_password"=w1401, "input_username"=w1402) -> ("output_Iconnected"=w1399:bool)  [unwired: 9 in]
              n910 = Select(t="Connection accepted!" ("message"), s=w1399, f="Error!") -> (s? t:f=w1397:string)
              n911 = One Button Dialog(message=w1397) -> ()  [unwired: 1 in, 1 out]
            }
            frame "SendData" {
              n912 = local read "Data Set Prefix"() -> (w1404:string)
              n913 = local read "Host Password"() -> (w1405:string)
              n914 = local read "Host UserName"() -> (w1406:string)
              n915 = call "myRIO_BRig_RT_comm_webdav_sendData_all.vi"("Host Filename Prefix"=w1404, "Host Password"=w1405, "Host UserName"=w1406) -> ()  [unwired: 9 in]
            }
            frame "Get_FPGA_count_per_ms" {
              # "Used to automatically determine how many FPGA cycles in 1 ms"
              n916 = case shown="False" w1419 {
                selector: w1419 -> [w1421 _]
                tunnel: w1417 -> [_ w1434]
                tunnel: [w1425 w1434] -> w1416
                tunnel: w1415 -> [w1424 w1432]
                tunnel: w1414 -> [w1423 w1431]
                tunnel: [w1422 w1429] -> w1409
                tunnel: [w1421 w1428] -> w1413
                frame False {
                  n917 = Get Date/Time In Seconds() -> (seconds since 1Jan1904=w1426:timestamp)
                  n918 = xnode "Read/Write Control"("FPGA VI Reference In"=w1424, "error in"=w1423, "timeTrial_trig"=TRUE ("timeTrial")) -> ("error out"=w1422:errorcluster)  [unwired: 1 out]
                  n919 = To Double Precision Float(number=w1426) -> (double precision float=w1425:dbl)
                  n920 = local write "get_countPerMS"(w1421) -> ()
                }
                frame True {
                  w1430 = 1.0
                  n921 = Get Date/Time In Seconds() -> (seconds since 1Jan1904=w1435:timestamp)
                  n922 = To Double Precision Float(number=w1435) -> (double precision float=w1436:dbl)
                  n923 = Subtract(x=w1436, y=w1434) -> (x-y=w1433:dbl)
                  n924 = Less Or Equal?(x=w1430, y=w1433) -> (x <= y?=w1428:bool)
                  n925 = case shown="True" w1428 {
                    tunnel: w1432 -> [_ w1449]
                    tunnel: w1431 -> [w1437 w1448]
                    tunnel: w1430 -> [_ w1439]
                    tunnel: [w1437 w1438] -> w1429
                    frame False {
                    }
                    frame True {
                      n926 = xnode "Read/Write Control"("FPGA VI Reference In"=w1449, "error in"=w1448) -> ("FPGA VI Reference Out"=w1446:refnum<k20>, "error out"=w1445:errorcluster, "timeTrial_count"=w1440:u32)
                      n927 = Multiply(x=w1439, y=1000.0) -> (x*y=w1443:dbl)
                      n928 = To Double Precision Float(number=w1440) -> (double precision float=w1442:dbl)
                      n929 = Divide(x=w1442, y=w1443) -> (x/y=w1444:dbl)
                      n930 = local write "FPGA_count2ms"(w1444) -> ()
                      n931 = xnode "Read/Write Control"("FPGA VI Reference In"=w1446, "error in"=w1445, "timeTrial_trig"=FALSE ("timeTrial")) -> ("error out"=w1438:errorcluster)  [unwired: 1 out]
                    }
                  }
                }
              }
              n932 = Select(t=myRIO_BRig_RT__Case_NonExp_stateList."Idle" ("Enum"), s=w1413, f=w1411) -> (s? t:f=w1410:T1)
              n933 = local write "error out"(w1409) -> ()
            }
            frame "End" {
            }
          }
          n934 = local read "MTrig_Audio_trig__R"() -> (w91:bool)
          n935 = local read "MTrig_Audio_trig__L"() -> (w92:bool)
          n936 = local read "MTrig_Laser_trig"() -> (w90:bool)
          n937 = local read "MTrig_CueLed"() -> (w83:bool)
          n938 = Compound Arithmetic op=OR(w92, w91, w90, w83) -> (w89:bool)
          n939 = local read "START"() -> (w115:bool)
          n940 = local read "STOP_abort"() -> (w114:bool)
          n941 = case shown="True" w89 {
            frame False {
            }
            frame True {
              w131 = FALSE
              n942 = local write "MTrig_Audio_trig__R"(w131) -> ()
              n943 = local write "MTrig_Audio_trig__L"(w131) -> ()
              n944 = local write "MTrig_Laser_trig"(w131) -> ()
              n945 = local write "MTrig_CueLed"(w131) -> ()
            }
          }
          n946 = call "myRIO_BRig_RT_dataMTrig_main__NoExp.vi"("input_dataMTrig"=w118, "input_Audio_trig_L"=w92, "input_Audio_trig_R"=w91, "input_Laser_trig"=w90, "input_CueLed"=w83) -> ("output_dataMTrig"=w117:u16[], "output_Audio_L"=w109:bool, "output_Audio_R"=w110:bool, "output_Laser"=w88:bool, "output_CueLed"=w82:bool)  [unwired: 10 in]
          n947 = Or(x=w115, y=w114) -> (x .or. y?=w113:bool)
          n948 = Select(t=myRIO_BRig_RT__Case_NonExp_stateList."End" ("Enum"), s=w113, f=w112) -> (s? t:f=w111:T1)
          n949 = Not(x="MTrig_Laser_Switch") -> (.not. x?=w85:bool)
          n950 = And(x=w88, y=w85) -> (x .and. y?=w86:bool)
          n951 = And(x=w88, y="MTrig_Laser_Switch") -> (x .and. y?=w87:bool)
          n952 = xnode "Read/Write Control"("FPGA VI Reference In"=w98, "error in"=w97, "A1_SR"=w119, "A3_SL"=w120, "audioTrigger_L"=w109, "audioTrigger_R"=w110, "LC_Laser_l1"=w86, "LC_Laser_l2"=w87, "CueLed_Event"=w82) -> ("FPGA VI Reference Out"=w125:refnum<k20>, "error out"=w124:errorcluster)
          n953 = node-c288() -> ()  [unwired: 1 in, 1 out]
          "cState_NonExp" <- w123
        }
        n954 = node-c288(w70) -> ()  [unwired: 1 out]
        n955 = flat-sequence {
          tunnel: w63 -> [w81]
          tunnel: [w81] -> w62
          tunnel: w61 -> [w80]
          tunnel: [w80] -> w60
          frame #0 {
            w79 = FALSE
            n956 = local write "STOP_endBlock"(w79) -> ()
            n957 = local write "STOP_endTrial"(w79) -> ()
          }
        }
      }
      frame True {
        w1462 = u16 0
        w1479 = u16 0 ("idxDataBlock")
        w1481 = u16 100 ("new element/subarray")
        w1482 = u16 100 ("new element/subarray")
        w1502 = T6 refnum items=["Session NI_WebDAV"] ("output_hSession")
        w1511 = FALSE
        # "dummyState counter"
        # "audio__L\naudio__R"
        # "Audio params"
        # "nRewards"
        # "idxDataBlock"
        # "Solenoid_Tdelay_R"
        # "Solenoid_Tdelay_L"
        # "RewCalib_N__R"
        # "RewCalib_N__L"
        # "Save dataLick to file\nSend file to Host\nSave dataMTrig\nSend file to Host\nDisconnect"
        # "dataTrial"
        # "dataTrial"
        # "Solenoid_Tcycle_R"
        # "Solenoid_Tcycle_L"
        # "Laser_Tcycle"
        # "Audio_Tcycle_R"
        # "Audio_Tcycle_L"
        # "dataLick"
        # "dataLC"
        # "dataLC"
        # "dataBlock"
        # "dataBlock"
        # "dataMTrig"
        # "dataMTrig"
        # "dataExp"
        # "dataCurrent"
        # "dataExp"
        # "dataCurrent"
        # "spout"
        # "state"
        n958 = call "myRIO_BRig_RT_dataMTrig_Solenoid_Tcycle__L.vi"() -> ("output_Solenoid_Tcycle__L"=w1508:i32)  [unwired: 11 in]
        n959 = call "myRIO_BRig_RT_dataMTrig_Solenoid_Tcycle__R.vi"() -> ("output_Solenoid_Tcycle__R"=w1507:i32)  [unwired: 11 in]
        n960 = call "myRIO_BRig_RT_dataMTrig_Audio_Tcycle__L.vi"() -> ("output_Audio_Tcycle__L"=w1506:i32)  [unwired: 11 in]
        n961 = call "myRIO_BRig_RT_dataMTrig_Audio_Tcycle__R.vi"() -> ("output_Audio_Tcycle__R"=w1505:i32)  [unwired: 11 in]
        n962 = call "myRIO_BRig_RT_dataMTrig_Laser_Tcycle.vi"() -> ("output_Laser_Tcycle"=w1504:i32)  [unwired: 11 in]
        n963 = local read "Tcycle_Reward_min_L"() -> (w1483:u16)
        n964 = local read "Tcycle_Reward_min_R"() -> (w1484:u16)
        n965 = local read "MTrig_Solenoid_Tcycle__L"() -> (w1487:u16)
        n966 = local read "MTrig_Solenoid_Tcycle__R"() -> (w1486:u16)
        n967 = local read "MTrig_Laser_Tcycle"() -> (w1485:u16)
        n968 = call "myRIO_BRig_RT_dataMTrig_Solenoid_RewCalib_nCycle__L.vi"() -> ("output_Solenoid_RewCalib_nCycle__L"=w1490:i32)  [unwired: 11 in]
        n969 = call "myRIO_BRig_RT_dataMTrig_Solenoid_Tdelay__L.vi"() -> ("output_Solenoid_Tdelay__L"=w1492:i32)  [unwired: 11 in]
        n970 = call "myRIO_BRig_RT_dataMTrig_Solenoid_RewCalib_nCycle__R.vi"() -> ("output_Solenoid_RewCalib_nCycle__R"=w1491:i32)  [unwired: 11 in]
        n971 = call "myRIO_BRig_RT_dataMTrig_Solenoid_Tdelay__R.vi"() -> ("output_Solenoid_Tdelay__R"=w1493:i32)  [unwired: 11 in]
        n972 = case shown="False" w1472 {
          selector: w1472 -> [_ w1533]
          tunnel: w1471 -> [w1530 w1535]
          tunnel: [w1531 w1535] -> w1467
          tunnel: w1470 -> [_ w1534]
          tunnel: [w1532 w1534] -> w1468
          tunnel: [w1529 w1533] -> w1466
          frame False {
            n973 = call "myRIO__TCP_connect_forWriting.vi"("input_error"=w1530) -> ("output_error"=w1531:errorcluster, "output_connected"=w1529:bool, "output_hTCP"=w1532:refnum<k5>)  [unwired: 8 in]
          }
          frame True {
          }
        }
        n974 = call "myRIO_BRig_RT_dataLick_init.vi"() -> ("output_dataLick"=w1513:u16[][])  [unwired: 11 in]
        n975 = call "myRIO_BRig_RT_dataCurrent_init.vi"() -> ("output_dataCurrent"=w1520:u16[])  [unwired: 11 in]
        n976 = call "myRIO_BRig_RT_dataExp_init.vi"() -> ("output_dataExp"=w1519:u16[])  [unwired: 11 in]
        n977 = call "myRIO_BRig_RT_dataMTrig_init.vi"() -> ("output_dataMTrig"=w1510:u16[])  [unwired: 5 in]
        n978 = call "myRIO_BRig_RT_dataLC_init.vi"() -> ("output_dataLC"=w1517:u16[])  [unwired: 11 in]
        n979 = call "myRIO_BRig_RT_dataBlock_init.vi"() -> ("output_dataBlock"=w1518:u16[][])  [unwired: 11 in]
        n980 = call "myRIO_BRig_RT_dataTrial_init.vi"() -> ("output_dataTrial"=w1503:u16[][])  [unwired: 11 in]
        n981 = local write "I_connect_TCP"(w1466) -> ()
        n982 = Replace Array Subset(array=w1510, new element #1=w1482, index #1=w1490, new element #2=w1482, index #2=w1491, new element #3=w1481, index #3=w1492, new element #4=w1481, index #4=w1493, new element #5=w1487, index #5=w1508, new element #6=w1486, index #6=w1507, new element #7=w1483, index #7=w1506, new element #8=w1484, index #8=w1505, new element #9=w1485, index #9=w1504) -> (w1509:u16[])
        n983 = call "myRIO_BRig_RT_dataAnalog_init.vi"() -> ("output_dataAnalog"=w1477:u16[][])  [unwired: 11 in]
        n984 = call "myRIO_BRig_RT_TCP__start_exp.vi"("input_hTCP"=w1468, "input_I_connected_TCP"=w1466, "input_error"=w1467) -> ("output_hTCP"=w1465:refnum<k5>, "output_error"=w1464:errorcluster)  [unwired: 11 in]
        n985 = Get Date/Time In Seconds() -> (seconds since 1Jan1904=w1489:timestamp)
        n986 = call "myRIO_BRig_RT_arrTrig_init.vi"() -> ("output_arrTrig"=w1461:bool[])  [unwired: 11 in]
        n987 = To Double Precision Float(number=w1489) -> (double precision float=w1488:dbl)
        n988 = node-c288() -> (w1528:T3)  [unwired: 4 in]
        n989 = timed-loop {
          timing: w1528 -> [_]
          timing-out: [_] -> w1527
          shift-right: [w1662] -> _
          shift-left: myRIO_BRig_RT__Case_Exp_stateList."Start1" ("Enum") -> [w1586]
          shift-right: [w1620] -> _
          shift-left: enum16{"Left", "Right"}."Left" -> [w1702]
          tunnel: w1460 -> [w1700]
          tunnel: w1459 -> [w1592]
          shift-right: [w1695] -> _
          shift-left: w1525 -> [w1699]
          shift-right: [w1694] -> _
          shift-left: w1524 -> [w1698]
          tunnel: [w1678] -> w1522
          tunnel: [w1679] -> w1523
          shift-right: [w1680] -> w1494
          shift-left: w1520 -> [w1581]
          shift-right: [w1693] -> _
          shift-left: w1519 -> [w1653]
          shift-right: [w1674] -> w1498
          shift-left: w1509 -> [w1675]
          shift-right: [w1691] -> _
          shift-left: w1518 -> [w1692]
          shift-right: [w1689] -> _
          shift-left: w1517 -> [w1690]
          shift-right: [w1681] -> w1500
          shift-left: w1513 -> [w1682]
          shift-right: [w1651] -> _
          shift-left: w1511 -> [w1676]
          shift-right: [w1652] -> _
          shift-left: w1511 -> [w1677]
          shift-right: [w1660] -> _
          shift-left: w1503 -> [w1661]
          shift-right: [w1659] -> w1496
          shift-left: w1502 -> [w1657]
          shift-right: [w1658] -> w1497
          shift-left: FALSE ("output_Iconnected") -> [w1656]
          tunnel: "Data Set Prefix" -> [w1655]
          tunnel: [w1655] -> w1495
          tunnel: w1488 -> [w1654]
          shift-right: [w1649] -> _
          shift-left: 0 ("idxDataBlock") -> [w1650]
          shift-right: [w1646] -> _
          shift-left: w1479 -> [w1648]
          shift-right: [w1645] -> _
          shift-left: w1479 -> [w1647]
          shift-right: [w1639] -> w1475
          shift-left: 0 -> [w1625]
          shift-right: [w1621] -> _
          shift-left: w1462 -> [w1634]
          shift-right: [w1622] -> _
          shift-left: w1462 -> [w1631]
          shift-right: [w1630] -> _
          shift-left: w1462 -> [w1637]
          shift-right: [w1640] -> w1476
          shift-left: w1477 -> [w1641]
          tunnel: w1465 -> [w1629]
          tunnel: [w1628] -> w1474
          tunnel: w1466 -> [w1626]
          tunnel: [w1626] -> w1473
          tunnel: w1464 -> [w1627]
          tunnel: [w1589] -> w1469
          shift-right: [w1618] -> _
          shift-left: u16 0 -> [w1619]
          shift-right: [w1616] -> _
          shift-left: w1462 -> [w1617]
          shift-right: [w1613] -> _
          shift-left: w1461 -> [w1614]
          shift-right: [w1584] -> _
          shift-left: FALSE -> [w1587]
          stop <- w1688 stop-if-true
          # "arrTrig"
          # "arrTrig"
          # "LC_Laser_l2"
          # "LC_Event_l2"
          # "LC_Laser_l1"
          # "LC_Event_l1"
          # "CueLed"
          # "LC_Laser_l2"
          # "LC_Event_l2"
          # "LC_Laser_l1"
          # "LC_Event_l1"
          # "solenoid__R"
          # "solenoid__L"
          # "spout"
          # "iState"
          # "dataAnalog"
          # "index"
          # "iEvent"
          # "iBlock"
          # "iTrial"
          # "Laser"
          # "Audio R"
          # "Audio L"
          # "Solenoid R"
          # "Solenoid L"
          # "manual triggering"
          # "dataTrial"
          # "dataBlock"
          # "nRewards"
          # "dataExp"
          # "dataCurrent"
          # "audio__L\naudio__R"
          # "time stamp"
          # "nRewards"
          # "idxDataBlock"
          # "idxDataBlock"
          # "audio__L\naudio__R"
          # "dataLC"
          # "solenoid__R"
          # "solenoid__L"
          # "Did a lick occur?"
          # "Update lick counter"
          # "spout"
          # "spout"
          # "state"
          # "state"
          n990 = node-c288() -> ()  [unwired: 1 in, 1 out]
          n991 = flat-sequence {
            tunnel: w1592 -> [w1703]
            tunnel: [w1703] -> _
            tunnel: [w1704] -> w1588
            tunnel: [w1703] -> w1591
            frame #0 {
              n992 = Get Date/Time In Seconds() -> (seconds since 1Jan1904=w1704:timestamp)
            }
          }
          n993 = xnode "Read/Write Control"("FPGA VI Reference In"=w1700, "error in"=w1591) -> ("FPGA VI Reference Out"=w1644:refnum<k20>, "error out"=w1643:errorcluster, "A2_LickL"=w1695:u32, "A4_LickR"=w1694:u32)
          "A2" <- w1695
          "A4" <- w1694
          n994 = Greater?(x=w1695, y=w1699) -> (0:w1697:bool)
          n995 = Greater?(x=w1694, y=w1698) -> (0:w1696:bool)
          n996 = call "myRIO_BRig_RT_dataCurrent_IallReward_L.vi"() -> ("output_IallReward_L"=w1582:i32)  [unwired: 11 in]
          n997 = call "myRIO_BRig_RT_dataCurrent_IallReward_R.vi"() -> ("output_IallReward_R"=w1583:i32)  [unwired: 11 in]
          n998 = Or(x=w1697, y=w1696) -> (x .or. y?=w1701:bool)
          n999 = local read "MTrig_Solenoid_trig__L"() -> (w1672:bool)
          n1000 = local read "MTrig_Solenoid_trig__R"() -> (w1671:bool)
          n1001 = local read "MTrig_Audio_trig__L"() -> (w1670:bool)
          n1002 = local read "MTrig_Audio_trig__R"() -> (w1669:bool)
          n1003 = local read "MTrig_Laser_trig"() -> (w1668:bool)
          n1004 = Index Array(array=w1581, index #1=w1582, index #2=w1583) -> (element #1=w1579:u16, element #2=w1580:u16)
          n1005 = Not Equal To 0?(x=w1579) -> (x != 0?=→"allReward_L":bool)
          n1006 = Not Equal To 0?(x=w1580) -> (x != 0?=→"allReward_R":bool)
          n1007 = case shown="\"saveSettings1\"" w1586 {
            selector: w1586 -> [_ _ _ _ _ _ _ _ _ _ _ _ _ _ _ _ _ _ _ _ _ _ _ _ _ w2671 _ w2714 _ _ _ _ _ w2811 _ w2871 _ _ _ _ _ w2974 _ w3025 _ w3081 _ w3121 _ _ w3179 _ _ _ _ _ w3326 _ _ _ _ _ _ _ _ _ _ _ _ w3559 w3588]
            tunnel: [myRIO_BRig_RT__Case_Exp_stateList."Start2" ("Enum") myRIO_BRig_RT__Case_Exp_stateList."Start3" ("Enum") myRIO_BRig_RT__Case_Exp_stateList."saveSettings1" ("Enum") myRIO_BRig_RT__Case_Exp_stateList."saveSettings2" ("Enum") myRIO_BRig_RT__Case_Exp_stateList."saveSettings3" ("Enum") myRIO_BRig_RT__Case_Exp_stateList."saveSettings4" ("Enum") myRIO_BRig_RT__Case_Exp_stateList."saveSettings_LC_ENL_l1" ("Enum") myRIO_BRig_RT__Case_Exp_stateList."saveSettings_LC_ENL_l2" ("Enum") myRIO_BRig_RT__Case_Exp_stateList."saveSettings_LC_Cue_l1" ("Enum") myRIO_BRig_RT__Case_Exp_stateList."saveSettings_LC_Cue_l2" ("Enum") myRIO_BRig_RT__Case_Exp_stateList."saveSettings6_LC_l1_Other" ("Enum") myRIO_BRig_RT__Case_Exp_stateList."SaveSettings6_LC_l2_Other" ("Enum") myRIO_BRig_RT__Case_Exp_stateList."setSettings_Audio" ("Enum") myRIO_BRig_RT__Case_Exp_stateList."setSettings_Laser" ("Enum") myRIO_BRig_RT__Case_Exp_stateList."commConnect" ("Enum") w2428 myRIO_BRig_RT__Case_Exp_stateList."initTrial" ("Enum") w2482 myRIO_BRig_RT__Case_Exp_stateList."initTrial3" ("Enum") myRIO_BRig_RT__Case_Exp_stateList."initTrial_LC_ENL1" ("Enum") myRIO_BRig_RT__Case_Exp_stateList."ENL1_pre" ("Enum") myRIO_BRig_RT__Case_Exp_stateList."initTrial_LC_Cue1" ("Enum") myRIO_BRig_RT__Case_Exp_stateList."initTrial_LC_Sel" ("Enum") myRIO_BRig_RT__Case_Exp_stateList."initTrial4" ("Enum") w2646 w2668 myRIO_BRig_RT__Case_Exp_stateList."ENL1Penalty" ("Enum") w2715 myRIO_BRig_RT__Case_Exp_stateList."endExp" ("Enum") myRIO_BRig_RT__Case_Exp_stateList."endExp" ("Enum") myRIO_BRig_RT__Case_Exp_stateList."endExp" ("Enum") myRIO_BRig_RT__Case_Exp_stateList."endExp" ("Enum") w2788 w2805 myRIO_BRig_RT__Case_Exp_stateList."Cue1Penalty" ("Enum") w2869 myRIO_BRig_RT__Case_Exp_stateList."endExp" ("Enum") myRIO_BRig_RT__Case_Exp_stateList."endExp" ("Enum") myRIO_BRig_RT__Case_Exp_stateList."endExp" ("Enum") myRIO_BRig_RT__Case_Exp_stateList."endExp" ("Enum") w2947 w2973 myRIO_BRig_RT__Case_Exp_stateList."SelectReward" ("Enum") w3026 myRIO_BRig_RT__Case_Exp_stateList."SelectRewardPost" ("Enum") w3082 myRIO_BRig_RT__Case_Exp_stateList."SelectWrong" ("Enum") w3117 myRIO_BRig_RT__Case_Exp_stateList."endTrial1" ("Enum") myRIO_BRig_RT__Case_Exp_stateList."SelectTimeout" ("Enum") w3181 myRIO_BRig_RT__Case_Exp_stateList."endTrial1" ("Enum") myRIO_BRig_RT__Case_Exp_stateList."endTrial2" ("Enum") myRIO_BRig_RT__Case_Exp_stateList."endTrial3" ("Enum") w3251 w3309 w3326 myRIO_BRig_RT__Case_Exp_stateList."initBlock" ("Enum") w3349 myRIO_BRig_RT__Case_Exp_stateList."commUpload_dataExp" ("Enum") myRIO_BRig_RT__Case_Exp_stateList."endBlock" ("Enum") myRIO_BRig_RT__Case_Exp_stateList."commUpload_dataLC" ("Enum") myRIO_BRig_RT__Case_Exp_stateList."commUpload_dataTrial" ("Enum") myRIO_BRig_RT__Case_Exp_stateList."commUpload_dataCurrent" ("Enum") myRIO_BRig_RT__Case_Exp_stateList."saveData_dataCurrent" ("Enum") myRIO_BRig_RT__Case_Exp_stateList."saveData_dataExp" ("Enum") myRIO_BRig_RT__Case_Exp_stateList."saveData_dataLC" ("Enum") myRIO_BRig_RT__Case_Exp_stateList."saveData_dataTrial" ("Enum") myRIO_BRig_RT__Case_Exp_stateList."commUpload_pre" ("Enum") w3558 w3587] -> w1662
            tunnel: [w1733 w1748 w1766 w1829 w1887 w1949 w2008 w2068 w2128 w2188 w2248 w2287 w2327 w2356 w2419 w2427 w2452 w2469 w2499 w2541 w2569 w2590 w2609 w2632 w2656 w2680 w2701 w2719 w2731 w2749 w2764 w2779 w2787 w2827 w2851 w2868 w2885 w2902 w2917 w2932 w2956 w2988 w3009 w3023 w3037 w3079 w3099 w3127 w3144 w3160 w3187 w3206 w3218 w3234 w3271 w3286 w3325 w3338 w3352 w3378 w3395 w3412 w3429 w3446 w3470 w3486 w3509 w3525 w3545 w3575 w3604] -> w1620
            tunnel: w1702 -> [w1733 w1748 w1766 w1829 w1887 w1949 w2008 w2068 w2128 w2188 w2248 w2287 w2327 w2356 w2419 w2429 w2452 w2469 w2499 w2541 w2569 w2590 w2609 w2632 w2656 w2680 w2701 w2719 w2731 w2749 w2764 w2779 w2787 w2827 w2851 w2868 w2885 w2902 w2917 w2932 w2956 w2988 w3009 w3023 w3037 w3079 w3099 w3127 w3144 w3160 w3187 w3206 w3218 w3234 w3271 w3286 w3325 w3338 w3352 w3378 w3395 w3412 w3429 w3446 w3470 w3486 w3509 w3525 w3545 w3575 w3604]
            tunnel: w1701 -> [w1736 w1751 w1763 w1832 w1890 w1952 w2011 w2071 w2131 w2191 w2251 w2290 w2330 w2359 w2422 w2444 w2459 w2483 w2518 w2552 w2579 w2598 w2618 w2641 w2647 w2667 w2704 w2722 w2737 w2752 w2767 w2782 w2791 w2810 w2857 w2875 w2890 w2905 w2920 w2935 w2955 w2987 w3014 w3033 w3064 w3087 w3110 w3130 w3143 w3172 w3192 w3203 w3222 w3233 w3278 w3308 w3329 w3335 w3357 w3381 w3398 w3415 w3432 w3449 w3473 w3489 w3512 w3528 w3548 w3578 w3607]
            tunnel: w1697 -> [w1735 w1750 w1764 w1831 w1889 w1951 w2010 w2070 w2130 w2190 w2250 w2289 w2329 w2358 w2421 w2443 w2458 w2484 w2517 w2553 w2580 w2599 w2619 w2642 w2660 w2682 w2703 w2721 w2736 w2751 w2766 w2781 w2801 w2828 w2856 w2874 w2889 w2904 w2919 w2934 w2937 w2963 w3013 w3032 w3063 w3086 w3109 w3129 w3142 w3171 w3191 w3204 w3223 w3232 w3277 w3307 w3328 w3336 w3358 w3380 w3397 w3414 w3431 w3448 w3472 w3488 w3511 w3527 w3547 w3577 w3606]
            tunnel: w1696 -> [w1734 w1749 w1765 w1830 w1888 w1950 w2009 w2069 w2129 w2189 w2249 w2288 w2328 w2357 w2420 w2442 w2457 w2485 w2516 w2554 w2581 w2600 w2620 w2643 w2659 w2681 w2702 w2720 w2735 w2750 w2765 w2780 w2800 w2829 w2855 w2873 w2888 w2903 w2918 w2933 w2936 w2962 w3012 w3031 w3062 w3085 w3108 w3128 w3141 w3170 w3190 w3205 w3224 w3231 w3276 w3306 w3327 w3337 w3359 w3379 w3396 w3413 w3430 w3447 w3471 w3487 w3510 w3526 w3546 w3576 w3605]
            tunnel: [w1736 w1751 w1763 w1832 w1890 w1952 w2011 w2071 w2131 w2191 w2251 w2290 w2330 w2359 w2422 w2444 w2459 w2483 w2518 w2552 w2579 w2598 w2618 w2641 w2647 w2667 w2704 w2722 w2737 w2752 w2767 w2782 w2791 w2810 w2857 w2875 w2890 w2905 w2920 w2935 w2955 w2987 w3014 w3033 w3064 w3087 w3110 w3130 w3143 w3172 w3192 w3203 w3222 w3233 w3278 w3308 w3329 w3335 w3357 w3381 w3398 w3415 w3432 w3449 w3473 w3489 w3512 w3528 w3548 w3578 w3607] -> w1685
            tunnel: [w1735 w1750 w1764 w1831 w1889 w1951 w2010 w2070 w2130 w2190 w2250 w2289 w2329 w2358 w2421 w2443 w2458 w2484 w2517 w2553 w2580 w2599 w2619 w2642 w2660 w2682 w2703 w2721 w2736 w2751 w2766 w2781 w2801 w2828 w2856 w2874 w2889 w2904 w2919 w2934 w2937 w2963 w3013 w3032 w3063 w3086 w3109 w3129 w3142 w3171 w3191 w3204 w3223 w3232 w3277 w3307 w3328 w3336 w3358 w3380 w3397 w3414 w3431 w3448 w3472 w3488 w3511 w3527 w3547 w3577 w3606] -> w1684
            tunnel: [w1734 w1749 w1765 w1830 w1888 w1950 w2009 w2069 w2129 w2189 w2249 w2288 w2328 w2357 w2420 w2442 w2457 w2485 w2516 w2554 w2581 w2600 w2620 w2643 w2659 w2681 w2702 w2720 w2735 w2750 w2765 w2780 w2800 w2829 w2855 w2873 w2888 w2903 w2918 w2933 w2936 w2962 w3012 w3031 w3062 w3085 w3108 w3128 w3141 w3170 w3190 w3205 w3224 w3231 w3276 w3306 w3327 w3337 w3359 w3379 w3396 w3413 w3430 w3447 w3471 w3487 w3510 w3526 w3546 w3576 w3605] -> w1683
            tunnel: w1581 -> [w1732 w1747 w1762 w1796 w1872 w1891 w1953 w2067 w2127 w2187 w2247 w2286 w2326 w2354 w2373 w2435 w2451 w2481 w2488 w2530 w2568 w2589 w2608 w2631 w2648 w2670 w2695 w2718 w2732 w2748 w2763 w2778 w2790 w2812 w2850 w2872 w2886 w2901 w2916 w2931 w2949 w2976 w2989 w3028 w3039 w3084 w3100 w3126 w3140 w3161 w3189 w3202 w3215 w3236 w3253 w3284 w3324 w3339 w3360 w3375 w3392 w3409 w3426 w3437 w3463 w3478 w3498 w3522 w3538 w3557 w3586]
            tunnel: w1653 -> [w1731 w1746 w1761 w1827 w1885 w1946 w2005 w2065 w2125 w2185 w2245 w2284 w2324 w2347 w2365 w2432 w2456 w2480 w2486 w2525 w2571 w2582 w2612 w2635 w2658 w2679 w2694 w2716 w2734 w2747 w2762 w2777 w2786 w2826 w2848 w2867 w2887 w2900 w2915 w2930 w2939 w2964 w3010 w3030 w3056 w3080 w3101 w3124 w3139 w3163 w3186 w3201 w3221 w3225 w3252 w3299 w3323 w3340 w3361 w3374 w3391 w3408 w3425 w3438 w3467 w3483 w3494 w3521 w3542 w3572 w3601]
            tunnel: [w1732 w1747 w1762 w1796 w1872 w1891 w1953 w2067 w2127 w2187 w2247 w2286 w2326 w2354 w2372 w2434 w2451 w2474 w2487 w2529 w2568 w2588 w2607 w2630 w2645 w2669 w2696 w2717 w2732 w2748 w2763 w2778 w2789 w2806 w2849 w2870 w2886 w2901 w2916 w2931 w2948 w2975 w3011 w3027 w3057 w3083 w3102 w3125 w3140 w3164 w3188 w3202 w3214 w3235 w3253 w3282 w3324 w3339 w3360 w3375 w3392 w3409 w3426 w3437 w3463 w3478 w3498 w3522 w3538 w3557 w3586] -> w1594
            tunnel: [w1731 w1746 w1761 w1826 w1884 w1941 w2004 w2065 w2125 w2185 w2245 w2284 w2324 w2347 w2364 w2433 w2456 w2479 w2486 w2525 w2571 w2582 w2612 w2635 w2658 w2679 w2694 w2716 w2734 w2747 w2762 w2777 w2786 w2826 w2848 w2867 w2887 w2900 w2915 w2930 w2939 w2964 w3010 w3030 w3056 w3080 w3101 w3124 w3139 w3163 w3186 w3201 w3221 w3225 w3252 w3299 w3323 w3340 w3361 w3374 w3391 w3408 w3425 w3438 w3467 w3483 w3497 w3521 w3542 w3572 w3601] -> w1693
            tunnel: [_ _ _ _ _ _ _ _ _ _ _ _ _ _ _ _ _ _ _ _ _ _ _ _ _ _ _ _ _ _ _ _ _ _ _ _ _ _ _ _ _ _ _ w3021 _ _ _ _ _ _ _ _ _ _ _ _ _ _ _ _ _ _ _ _ _ _ _ _ _ _ _] -> w1611
            tunnel: [_ _ _ _ _ _ _ _ _ _ _ _ _ _ _ _ _ _ _ _ _ _ _ _ _ _ _ _ _ _ _ _ _ _ _ _ _ _ _ _ _ _ _ w3022 _ _ _ _ _ _ _ _ _ _ _ _ _ _ _ _ _ _ _ _ _ _ _ _ _ _ _] -> w1665
            tunnel: w1692 -> [w1729 w1744 w1759 w1798 w1874 w1947 w2006 w2066 w2126 w2186 w2246 w2285 w2325 w2352 w2416 w2424 w2453 w2464 w2509 w2550 w2577 w2585 w2604 w2627 w2657 w2678 w2691 w2712 w2733 w2745 w2760 w2775 w2799 w2825 w2847 w2865 w2883 w2898 w2913 w2928 w2961 w2985 w3007 w3029 w3041 w3077 w3098 w3122 w3137 w3162 w3185 w3199 w3217 w3240 w3274 w3295 w3321 w3342 w3363 w3372 w3389 w3406 w3423 w3443 w3457 w3480 w3504 w3519 w3540 w3570 w3599]
            tunnel: [w1729 w1744 w1759 w1798 w1874 w1947 w2006 w2066 w2126 w2186 w2246 w2285 w2325 w2352 w2416 w2423 w2450 w2464 w2509 w2550 w2577 w2585 w2604 w2627 w2657 w2678 w2691 w2712 w2733 w2745 w2760 w2775 w2799 w2825 w2847 w2865 w2883 w2898 w2913 w2928 w2961 w2985 w3007 w3029 w3040 w3077 w3098 w3122 w3137 w3162 w3185 w3199 w3216 w3240 w3274 w3295 w3321 w3342 w3363 w3372 w3389 w3406 w3423 w3443 w3457 w3480 w3504 w3519 w3540 w3570 w3599] -> w1691
            tunnel: w1690 -> [w1730 w1745 w1760 w1797 w1873 w1948 w2007 w2063 w2123 w2183 w2243 w2282 w2322 w2353 w2417 w2445 w2455 w2478 w2498 w2551 w2578 w2591 w2610 w2633 w2655 w2666 w2692 w2713 w2730 w2746 w2761 w2776 w2798 w2814 w2846 w2866 w2884 w2899 w2914 w2929 w2960 w2986 w3008 w3024 w3054 w3078 w3097 w3123 w3138 w3159 w3184 w3200 w3220 w3239 w3275 w3298 w3322 w3341 w3362 w3373 w3390 w3407 w3424 w3444 w3466 w3482 w3506 w3517 w3541 w3571 w3600]
            tunnel: [w1730 w1745 w1760 w1797 w1873 w1948 w2007 w2064 w2124 w2184 w2244 w2283 w2323 w2353 w2417 w2445 w2455 w2478 w2498 w2551 w2578 w2591 w2610 w2633 w2655 w2666 w2692 w2713 w2730 w2746 w2761 w2776 w2798 w2814 w2846 w2866 w2884 w2899 w2914 w2929 w2960 w2986 w3008 w3024 w3054 w3078 w3097 w3123 w3138 w3159 w3184 w3200 w3220 w3239 w3275 w3298 w3322 w3341 w3362 w3373 w3390 w3407 w3424 w3444 w3466 w3482 w3506 w3517 w3541 w3571 w3600] -> w1689
            tunnel: [_ _ _ _ _ _ _ _ _ _ _ _ _ _ _ _ _ _ _ _ _ _ _ _ _ _ _ _ _ _ _ _ _ _ _ _ _ _ _ _ _ _ _ _ _ _ _ _ _ _ _ _ _ _ _ _ TRUE _ _ _ _ _ _ _ _ _ _ _ _ _ _] -> w1686
            tunnel: w1677 -> [_ _ _ _ _ _ _ _ _ _ _ _ _ _ _ _ _ _ _ _ _ _ _ _ _ _ _ _ _ _ _ _ _ w2824 _ _ _ _ _ _ _ _ _ _ _ _ _ _ _ _ _ _ _ _ _ _ _ _ _ _ _ _ _ _ _ _ _ _ _ _ _]
            tunnel: w1676 -> [_ _ _ _ _ _ _ _ _ _ _ _ _ _ _ _ _ _ _ _ _ _ _ _ _ _ _ _ _ _ _ _ _ w2823 _ _ _ _ _ _ _ _ _ _ _ _ _ _ _ _ _ _ _ _ _ _ _ _ _ _ _ _ _ _ _ _ _ _ _ _ _]
            tunnel: [_ _ _ _ _ _ _ _ _ _ _ _ _ _ _ _ _ _ _ _ _ _ _ _ _ _ _ _ _ _ _ _ w2785 w2824 _ _ _ _ _ _ _ _ _ _ _ _ _ _ _ _ _ _ _ _ _ _ _ _ _ _ _ _ _ _ _ _ _ _ _ _ _] -> w1652
            tunnel: [_ _ _ _ _ _ _ _ _ _ _ _ _ _ _ _ _ _ _ _ _ _ _ _ _ _ _ _ _ _ _ _ w2784 w2823 _ _ _ _ _ _ _ _ _ _ _ _ _ _ _ _ _ _ _ _ _ _ _ _ _ _ _ _ _ _ _ _ _ _ _ _ _] -> w1651
            tunnel: w1661 -> [w1727 w1742 w1757 w1788 w1870 w1936 w2003 w2050 w2115 w2170 w2230 w2257 w2307 w2346 w2415 w2441 w2454 w2477 w2501 w2543 w2567 w2587 w2606 w2629 w2654 w2677 w2689 w2711 w2728 w2743 w2758 w2773 w2797 w2822 w2844 w2864 w2881 w2896 w2911 w2926 w2959 w2984 w2997 w3020 w3052 w3076 w3093 w3116 w3136 w3155 w3178 w3198 w3213 w3238 w3267 w3294 w3319 w3343 w3364 w3371 w3388 w3405 w3422 w3442 w3465 w3481 w3505 w3520 w3535 w3569 w3598]
            tunnel: [w1727 w1742 w1757 w1788 w1870 w1936 w2003 w2050 w2115 w2170 w2230 w2257 w2307 w2346 w2415 w2441 w2454 w2477 w2500 w2542 w2560 w2586 w2605 w2628 w2654 w2677 w2689 w2711 w2728 w2743 w2758 w2773 w2797 w2822 w2844 w2864 w2881 w2896 w2911 w2926 w2959 w2984 w2997 w3020 w3052 w3076 w3093 w3116 w3136 w3155 w3178 w3198 w3213 w3237 w3267 w3294 w3319 w3343 w3364 w3371 w3388 w3405 w3422 w3442 w3465 w3481 w3505 w3520 w3535 w3569 w3598] -> w1660
            tunnel: [w1726 w1741 w1756 w1787 w1869 w1935 w2002 w2049 w2114 w2169 w2229 w2256 w2306 w2345 w2414 w2440 w2461 w2476 w2511 w2549 w2576 w2597 w2617 w2640 w2653 w2676 w2688 w2710 w2727 w2742 w2757 w2772 w2796 w2821 w2843 w2863 w2880 w2895 w2910 w2925 w2958 w2983 w2996 w3019 w3051 w3075 w3092 w3115 w3135 w3154 w3177 w3197 w3212 w3230 w3273 w3293 w3317 w3344 w3354 w3370 w3387 w3404 w3421 w3441 w3469 w3485 w3508 w3524 w3544 w3574 w3603] -> w1659
            tunnel: [w1725 w1740 w1755 w1786 w1868 w1934 w2001 w2048 w2113 w2168 w2228 w2255 w2305 w2344 w2413 w2439 w2460 w2475 w2510 w2548 w2575 w2596 w2616 w2639 w2652 w2675 w2687 w2709 w2726 w2741 w2756 w2771 w2795 w2820 w2842 w2862 w2879 w2894 w2909 w2924 w2957 w2982 w2995 w3018 w3050 w3074 w3091 w3114 w3134 w3153 w3176 w3196 w3211 w3229 w3272 w3292 w3318 w3330 w3351 w3376 w3393 w3410 w3427 w3445 w3468 w3484 w3507 w3523 w3543 w3573 w3602] -> w1658
            tunnel: w1657 -> [w1726 w1741 w1756 w1787 w1869 w1935 w2002 w2049 w2114 w2169 w2229 w2256 w2306 w2345 w2414 w2440 w2461 w2476 w2511 w2549 w2576 w2597 w2617 w2640 w2653 w2676 w2688 w2710 w2727 w2742 w2757 w2772 w2796 w2821 w2843 w2863 w2880 w2895 w2910 w2925 w2958 w2983 w2996 w3019 w3051 w3075 w3092 w3115 w3135 w3154 w3177 w3197 w3212 w3230 w3273 w3293 w3317 _ w3354 w3370 w3387 w3404 w3421 w3441 w3469 w3485 w3508 w3524 w3544 w3574 w3603]
            tunnel: w1656 -> [w1725 w1740 w1755 w1786 w1868 w1934 w2001 w2048 w2113 w2168 w2228 w2255 w2305 w2344 w2413 w2439 w2460 w2475 w2510 w2548 w2575 w2596 w2616 w2639 w2652 w2675 w2687 w2709 w2726 w2741 w2756 w2771 w2795 w2820 w2842 w2862 w2879 w2894 w2909 w2924 w2957 w2982 w2995 w3018 w3050 w3074 w3091 w3114 w3134 w3153 w3176 w3196 w3211 w3229 w3272 w3292 w3318 _ w3351 w3376 w3393 w3410 w3427 w3445 w3468 w3484 w3507 w3523 w3543 w3573 w3602]
            tunnel: w1655 -> [_ _ _ _ _ _ _ _ _ _ _ _ _ _ _ _ _ _ _ _ _ _ _ _ _ _ _ _ _ _ _ _ _ _ _ _ _ _ _ _ _ _ _ _ _ _ _ _ _ _ _ _ _ _ _ _ _ _ _ w3368 w3385 w3402 w3419 w3439 _ _ _ _ _ _ _]
            tunnel: w1654 -> [_ _ _ _ _ _ _ _ _ _ _ _ _ _ _ _ _ _ _ _ _ _ _ _ _ _ _ _ _ _ _ _ _ _ _ _ _ _ _ _ _ _ _ _ _ _ _ _ _ _ _ _ _ _ _ _ _ _ _ _ _ _ _ _ _ _ w3499 _ _ _ _]
            tunnel: [w1724 w1739 w1754 w1785 w1867 w1933 w2000 w2047 w2112 w2167 w2227 w2254 w2304 w2343 w2412 w2430 w2448 w2473 w2512 w2547 w2574 w2595 w2615 w2638 w2651 w2674 w2686 w2708 w2725 w2740 w2755 w2770 w2794 w2819 w2841 w2861 w2878 w2893 w2908 w2923 w2954 w2981 w2994 w3017 w3035 w3073 w3090 w3113 w3133 w3152 w3175 w3195 w3210 w3228 w3270 w3279 w3316 w3333 w3353 w3367 w3384 w3401 w3418 w3436 w3452 w3477 w3493 w3516 w3533 w3568 w3597] -> w1649
            tunnel: w1650 -> [w1724 w1739 w1754 w1785 w1867 w1933 w2000 w2047 w2112 w2167 w2227 w2254 w2304 w2343 w2412 _ _ w2473 w2512 w2547 w2574 w2595 w2615 w2638 w2651 w2674 w2686 w2708 w2725 w2740 w2755 w2770 w2794 w2819 w2841 w2861 w2878 w2893 w2908 w2923 w2954 w2981 w2994 w3017 w3035 w3073 w3090 w3113 w3133 w3152 w3175 w3195 w3210 w3228 w3270 w3280 w3316 w3333 w3353 w3367 w3384 w3401 w3418 w3436 w3452 w3477 w3493 w3516 w3533 w3568 w3597]
            tunnel: w1648 -> [w1723 w1738 w1753 w1784 w1866 w1932 w1999 w2046 w2111 w2166 w2226 w2253 w2303 w2342 w2411 w2438 w2447 w2472 w2508 w2546 w2573 w2594 w2614 w2637 w2650 w2673 w2685 w2707 w2724 w2739 w2754 w2769 w2793 w2818 w2840 w2860 w2877 w2892 w2907 w2922 w2953 w2980 w2993 w3016 w3049 w3072 w3089 w3112 w3132 w3151 w3174 w3194 w3209 w3227 w3269 w3291 w3315 w3332 w3356 w3366 w3383 w3400 w3417 w3435 w3451 w3476 w3492 w3515 w3532 w3567 w3596]
            tunnel: w1647 -> [w1722 w1737 w1752 w1783 w1865 w1931 w1998 w2045 w2110 w2165 w2225 w2252 w2302 w2341 w2410 w2437 w2446 w2471 w2507 w2545 w2572 w2593 w2613 w2636 w2649 w2672 w2684 w2706 w2723 w2738 w2753 w2768 w2792 w2817 w2839 w2859 w2876 w2891 w2906 w2921 w2952 w2979 w2992 w3015 w3046 w3071 w3088 w3111 w3131 w3150 w3173 w3193 w3208 w3226 w3268 w3290 w3314 w3331 w3355 w3365 w3382 w3399 w3416 w3434 w3450 w3475 w3491 w3514 w3531 w3566 w3595]
            tunnel: [w1723 w1738 w1753 w1784 w1866 w1932 w1999 w2046 w2111 w2166 w2226 w2253 w2303 w2342 w2411 w2438 w2447 w2472 w2508 w2546 w2573 w2594 w2614 w2637 w2650 w2673 w2685 w2707 w2724 w2739 w2754 w2769 w2793 w2818 w2840 w2860 w2877 w2892 w2907 w2922 w2953 w2980 w2993 w3016 w3048 w3072 w3089 w3112 w3132 w3151 w3174 w3194 w3209 w3227 w3269 w3291 w3315 w3332 w3356 w3366 w3383 w3400 w3417 w3435 w3451 w3476 w3492 w3515 w3532 w3567 w3596] -> w1646
            tunnel: [w1722 w1737 w1752 w1783 w1865 w1931 w1998 w2045 w2110 w2165 w2225 w2252 w2302 w2341 w2410 w2437 w2446 w2471 w2507 w2545 w2572 w2593 w2613 w2636 w2649 w2672 w2684 w2706 w2723 w2738 w2753 w2768 w2792 w2817 w2839 w2859 w2876 w2891 w2906 w2921 w2952 w2979 w2992 w3015 w3047 w3071 w3088 w3111 w3131 w3150 w3173 w3193 w3208 w3226 w3268 w3290 w3314 w3331 w3355 w3365 w3382 w3399 w3416 w3434 w3450 w3475 w3491 w3514 w3531 w3566 w3595] -> w1645
            tunnel: w1644 -> [w1721 _ _ _ _ _ _ _ _ _ _ _ _ w2338 w2407 _ _ w2468 w2515 w2537 w2558 _ _ w2623 _ _ _ _ _ _ _ _ _ w2816 _ _ _ _ _ _ w2950 w2978 _ _ _ _ _ _ _ w3149 _ _ _ _ w3249 _ w3312 _ _ _ _ _ _ _ _ _ _ _ _ _ _]
            tunnel: w1643 -> [w1720 _ _ _ _ _ _ _ _ _ _ _ _ w2337 w2408 _ _ w2467 w2514 w2536 w2557 _ _ w2622 _ _ _ _ _ _ _ _ _ w2815 _ _ _ _ _ _ w2951 w2977 _ _ _ _ _ _ _ w3148 _ _ _ _ w3248 _ w3311 _ _ _ _ _ _ _ _ _ _ _ _ _ _]
            tunnel: [_ _ _ _ _ _ _ _ _ _ _ _ _ _ _ _ _ _ _ _ _ _ _ _ _ w2664 _ _ _ _ _ _ _ w2802 _ _ _ _ _ _ w2943 w2969 _ _ _ _ _ _ _ _ _ _ _ _ _ _ _ _ _ _ _ _ _ _ _ _ _ _ _ _ _] -> w1602
            tunnel: [_ _ _ _ _ _ _ _ _ _ _ _ _ _ _ _ _ _ _ _ _ _ _ _ _ w2663 _ _ _ _ _ _ _ w2803 _ _ _ _ _ _ w2942 w2968 _ _ _ _ _ _ _ _ _ _ _ _ _ _ _ _ _ _ _ _ _ _ _ _ _ _ _ _ _] -> w1601
            tunnel: [_ _ _ _ _ _ _ _ _ _ _ _ _ _ _ _ _ _ _ _ _ _ TRUE ("Recording") _ _ _ _ _ _ _ _ _ _ _ _ _ _ _ _ _ _ _ _ _ _ _ _ _ _ _ _ _ _ _ _ _ _ _ _ _ _ _ _ _ _ _ _ _ _ _ _] -> w1638
            tunnel: [_ _ _ _ _ _ _ _ _ _ _ _ _ _ _ TRUE _ _ _ _ _ _ _ _ _ _ _ _ _ _ _ _ _ _ _ _ _ _ _ _ _ _ _ _ _ _ _ _ _ _ _ _ _ _ _ _ _ _ _ _ _ _ _ _ _ _ _ _ _ _ _] -> w1635
            tunnel: [_ _ _ _ _ _ _ _ _ _ _ _ _ _ _ _ _ TRUE _ _ _ _ _ _ _ _ _ _ _ _ _ _ _ _ _ _ _ _ _ _ _ _ _ _ _ _ _ _ _ _ _ _ _ _ _ _ _ _ _ _ _ _ _ _ _ _ _ _ _ _ _] -> w1633
            tunnel: [_ _ _ _ _ _ _ _ _ _ _ _ _ _ _ _ _ w2463 _ _ _ _ _ _ _ _ _ _ _ _ _ _ _ _ _ _ _ _ _ _ _ _ _ _ _ _ _ _ _ _ _ _ _ _ _ _ _ _ _ _ _ _ _ _ _ _ _ _ _ _ _] -> w1632
            tunnel: w1619 -> [_ _ _ _ _ _ _ _ _ _ _ _ _ _ _ _ _ _ _ _ _ _ _ _ _ _ _ _ _ _ _ _ _ _ _ _ _ _ _ _ _ _ _ _ _ _ _ _ _ _ _ _ _ _ _ _ _ _ _ _ _ _ _ _ _ _ _ _ _ w3564 w3593]
            tunnel: [_ _ _ _ _ _ _ _ _ _ _ _ _ _ _ _ _ _ _ _ _ _ _ _ _ _ _ _ _ _ _ _ _ _ _ _ _ _ _ _ _ _ _ _ _ _ _ _ _ _ _ _ _ _ _ _ _ _ _ _ _ _ _ _ _ _ _ _ _ w3562 w3591] -> w1618
            tunnel: w1614 -> [_ _ _ _ _ _ _ _ _ _ _ _ _ _ _ _ _ _ _ _ w2559 w2584 w2603 w2626 w2644 w2665 w2683 w2705 _ _ _ _ w2783 w2813 w2838 w2858 _ _ _ _ w2944 w2970 _ _ _ _ _ _ _ _ _ _ _ _ _ _ _ _ _ _ _ _ _ _ _ _ _ _ _ _ _]
            tunnel: [_ _ _ _ _ _ _ _ _ _ _ _ _ _ _ _ _ _ _ w2527 w2559 w2583 w2602 w2625 w2644 w2665 w2683 w2705 _ _ _ _ w2783 w2813 w2838 w2858 _ _ _ _ w2944 w2970 _ _ _ _ _ _ _ _ _ _ _ _ _ _ _ _ _ _ _ _ _ _ _ _ _ _ _ _ _] -> w1613
            tunnel: [_ _ _ _ _ _ _ _ _ _ _ _ _ _ _ _ _ _ _ _ _ _ _ _ _ w2662 _ _ _ _ _ _ _ w2807 _ _ _ _ _ _ w2941 w2967 _ _ _ _ _ _ _ _ _ _ _ _ _ _ _ _ _ _ _ _ _ _ _ _ _ _ _ _ _] -> w1606
            tunnel: [_ _ _ _ _ _ _ _ _ _ _ _ _ _ _ _ _ _ _ _ _ _ _ _ _ w2661 _ _ _ _ _ _ _ w2808 _ _ _ _ _ _ w2940 w2966 _ _ _ _ _ _ _ _ _ _ _ _ _ _ _ _ _ _ _ _ _ _ _ _ _ _ _ _ _] -> w1604
            tunnel: [_ _ _ _ _ _ _ _ _ _ _ _ _ _ _ _ _ _ _ _ _ _ _ _ _ _ _ _ _ _ _ _ _ w2809 _ _ _ _ _ _ _ _ _ _ _ _ _ _ _ _ _ _ _ _ _ _ _ _ _ _ _ _ _ _ _ _ _ _ _ _ _] -> w1610
            tunnel: [_ _ _ _ _ _ _ _ _ _ _ _ _ _ _ w2425 _ _ _ _ _ _ _ _ _ _ _ _ _ _ _ _ _ _ _ _ _ _ _ _ _ _ _ _ _ _ _ _ _ _ _ _ _ _ _ _ _ _ _ _ _ _ _ _ _ _ _ _ _ _ _] -> w1593
            frame "Start1", Default {
              w1719 = FALSE ("SelectionState")
              n1008 = local read "CueLed_baseline"() -> (w1718:bool)
              n1009 = local read "Laser2_baseline"() -> (w1717:bool)
              n1010 = local read "Laser1_baseline"() -> (w1716:bool)
              n1011 = xnode "Read/Write Control"("FPGA VI Reference In"=w1721, "error in"=w1720, "SelectionState"=w1719, "LR_reward_Laser_l1"=w1719, "LR_wrong_Laser_l1"=w1719, "LR_reward_Event_l1"=w1719, "LR_wrong_Event_l1"=w1719, "Left(F)_or_Right(T)"=w1719, "ignoreWrong"=w1719, "SelectionState"=w1719, "LR_reward_Laser_l2"=w1719, "LR_wrong_laser_l2"=w1719, "LR_reward_Event_l2"=w1719, "LR_wrong_Event_l2"=w1719, "LC_Event_l1"=w1719, "LC_Laser_l1"=w1719, "LC_Laser_l2"=w1719, "LC_Event_l2"=w1719, "CueLed_Event"=w1719, "I_allReward"=w1719, "CueLed_Baseline"=w1718, "L2Led_Baseline"=w1717, "L1Led_Baseline"=w1716) -> ()  [unwired: 2 out]
            }
            frame "Start2" {
            }
            frame "Start3" {
            }
            frame "saveSettings1" {
              n1012 = call "myRIO_BRig_RT_dataExp_Tcycle_Reward_min_L.vi"() -> ("output_Tcycle_Reward_min_L"=w1772:i32)  [unwired: 11 in]
              n1013 = local read "Tcycle_Reward_min_L"() -> (w1771:u16)
              n1014 = call "myRIO_BRig_RT_dataExp_Audio_freq__L.vi"() -> ("output_Audio_freq__L"=w1804:i32)  [unwired: 11 in]
              n1015 = call "myRIO_BRig_RT_dataExp_Audio_freq__R.vi"() -> ("output_Audio_freq__R"=w1803:i32)  [unwired: 11 in]
              n1016 = call "myRIO_BRig_RT_dataExp_Audio_amp__L.vi"() -> ("output_Audio_amp__L"=w1802:i32)  [unwired: 11 in]
              n1017 = call "myRIO_BRig_RT_dataExp_Audio_amp__R.vi"() -> ("output_Audio_amp__R"=w1800:i32)  [unwired: 11 in]
              n1018 = call "myRIO_BRig_RT_dataExp_TPB_min__L.vi"() -> ("output_TPB_min__L"=w1812:i32)  [unwired: 11 in]
              n1019 = call "myRIO_BRig_RT_dataExp_TPB_min__R.vi"() -> ("output_TPB_min__R"=w1810:i32)  [unwired: 11 in]
              n1020 = call "myRIO_BRig_RT_dataExp_TPB_max__L.vi"() -> ("output_TPB_max__L"=w1808:i32)  [unwired: 11 in]
              n1021 = call "myRIO_BRig_RT_dataExp_TPB_max__R.vi"() -> ("output_TPB_max__R"=w1806:i32)  [unwired: 11 in]
              n1022 = call "myRIO_BRig_RT_dataExp_Cue1Param_AudioLed_Count_Switch.vi"() -> ("output_Cue1Param_AudioLed_Count_Switch"=w1778:i32)  [unwired: 11 in]
              n1023 = call "myRIO_BRig_RT_dataExp_Cue1Param_AudioLed_Probability_Switch.vi"() -> ("output_Cue1Param_AudioLed_Probability_Switch"=w1776:i32)  [unwired: 11 in]
              n1024 = call "myRIO_BRig_RT_dataExp_Cue1Param_CueType_Switch.vi"() -> ("output_Cue1Param_CueType_Switch"=w1774:i32)  [unwired: 11 in]
              n1025 = call "myRIO_BRig_RT_dataExp_ItrialUntilReward.vi"() -> ("output_I_trialUntilReward"=w1825:i32)  [unwired: 11 in]
              n1026 = call "myRIO_BRig_RT_dataExp_IblockUntilReward.vi"() -> ("output_I_blockUntilReward"=w1821:i32)  [unwired: 11 in]
              n1027 = call "myRIO_BRig_RT_dataExp_CueCycles.vi"() -> ("output_CueCycles"=w1820:i32)  [unwired: 11 in]
              n1028 = call "myRIO_BRig_RT_dataExp_ENL_min.vi"() -> ("output_ENL_min"=w1818:i32)  [unwired: 11 in]
              n1029 = call "myRIO_BRig_RT_dataExp_ENL_max.vi"() -> ("output_ENL_max"=w1816:i32)  [unwired: 11 in]
              n1030 = call "myRIO_BRig_RT_dataExp_ENL_penalty.vi"() -> ("output_ENL_penalty"=w1814:i32)  [unwired: 11 in]
              n1031 = local read "Audio_Freq__L"() -> (w1782:u8)
              n1032 = local read "Audio_Freq__R"() -> (w1780:u8)
              n1033 = local read "Audio_Amp__L"() -> (w1801:u16)
              n1034 = local read "TpB_Min_L"() -> (w1811:u16)
              n1035 = local read "TpB_Min_R"() -> (w1809:u16)
              n1036 = local read "TpB_Max_L"() -> (w1807:u16)
              n1037 = local read "TpB_Max_R"() -> (w1805:u16)
              n1038 = local read "Audio_Amp__R"() -> (w1799:u16)
              n1039 = local read "TrialUntilReward"() -> (w1824:bool)
              n1040 = local read "CueCycles"() -> (w1819:u16)
              n1041 = local read "Tcycle_ENL_min"() -> (w1817:u16)
              n1042 = local read "Tcycle_ENL_max"() -> (w1815:u16)
              n1043 = local read "Tcycle_ENLPenalty"() -> (w1813:u16)
              n1044 = local read "Cue1Param_AudioLed_Count_Switch"() -> (w1777:u16)
              n1045 = local read "Cue1Param_AudioLed_Probability_Switch"() -> (w1775:u16)
              n1046 = local read "Cue1Param_CueType_Switch"() -> (w1773:u16)
              n1047 = local read "Tcycle_Reward_max_L"() -> (w1769:u16)
              n1048 = call "myRIO_BRig_RT_dataExp_Tcycle_Reward_max_L.vi"() -> ("output_Tcycle_Reward_max_L"=w1770:i32)  [unwired: 11 in]
              n1049 = To Unsigned Word Integer(number=w1780) -> (unsigned 16bit integer=w1779:u16)
              n1050 = To Unsigned Word Integer(number=w1782) -> (unsigned 16bit integer=w1781:u16)
              n1051 = Boolean To (0,1)(Boolean=w1824) -> (0, 1=w1823:i16)
              n1052 = To Unsigned Word Integer(number=w1823) -> (unsigned 16bit integer=w1822:u16)
              n1053 = call "myRIO_BRig_RT_dataExp_Tcycle_Reward_step_L.vi"() -> ("output_Tcycle_Reward_step_L"=w1768:i32)  [unwired: 11 in]
              n1054 = local read "Tcycle_Reward_step_L"() -> (w1767:u16)
              n1055 = local read "BUR_min"() -> (w1793:u16)
              n1056 = local read "BUR_max"() -> (w1794:u16)
              n1057 = Not Equal To 0?(x=w1793) -> (x != 0?=w1792:bool)
              n1058 = Not Equal To 0?(x=w1794) -> (x != 0?=w1791:bool)
              n1059 = And(x=w1792, y=w1791) -> (x .and. y?=w1790:bool)
              n1060 = Boolean To (0,1)(Boolean=w1790) -> (0, 1=w1795:i16)
              n1061 = To Unsigned Word Integer(number=w1795) -> (unsigned 16bit integer=w1789:u16)
              n1062 = Replace Array Subset(array=w1827, new element #1=w1822, index #1=w1825, new element #2=w1789, index #2=w1821, new element #3=w1819, index #3=w1820, new element #4=w1817, index #4=w1818, new element #5=w1815, index #5=w1816, new element #6=w1813, index #6=w1814, new element #7=w1811, index #7=w1812, new element #8=w1809, index #8=w1810, new element #9=w1807, index #9=w1808, new element #10=w1805, index #10=w1806, new element #11=w1781, index #11=w1804, new element #12=w1779, index #12=w1803, new element #13=w1801, index #13=w1802, new element #14=w1799, index #14=w1800, new element #15=w1777, index #15=w1778, new element #16=w1775, index #16=w1776, new element #17=w1773, index #17=w1774, new element #18=w1771, index #18=w1772, new element #19=w1769, index #19=w1770, new element #20=w1767, index #20=w1768) -> (w1826:u16[])
            }
            frame "saveSettings2" {
              n1063 = call "myRIO_BRig_RT_dataExp_Tcycle_Reward_min_R.vi"() -> ("output_Tcycle_Reward_min_R"=w1846:i32)  [unwired: 11 in]
              n1064 = local read "Tcycle_Reward_min_R"() -> (w1845:u16)
              n1065 = call "myRIO_BRig_RT_dataExp_Tcycle_Cue1_Audio_min.vi"() -> ("output_Tcycle_Cue1_Audio_min"=w1877:i32)  [unwired: 11 in]
              n1066 = call "myRIO_BRig_RT_dataExp_Tcycle_Cue1_Audio_max.vi"() -> ("output_Tcycle_Cue1_Audio_max"=w1876:i32)  [unwired: 11 in]
              n1067 = call "myRIO_BRig_RT_dataExp_Tcycle_Cue1Penalty_Audio.vi"() -> ("output_Tcycle_Cue1Penalty_Audio"=w1875:i32)  [unwired: 11 in]
              n1068 = call "myRIO_BRig_RT_dataExp_Tcycle_RewardPost.vi"() -> ("output_Tcycle_RewardPost"=w1883:i32)  [unwired: 11 in]
              n1069 = call "myRIO_BRig_RT_dataExp_Tcycle_Wrong.vi"() -> ("output_Tcycle_Wrong"=w1881:i32)  [unwired: 11 in]
              n1070 = call "myRIO_BRig_RT_dataExp_Tcycle_Timeout.vi"() -> ("output_Tcycle_Timeout"=w1879:i32)  [unwired: 11 in]
              n1071 = call "myRIO_BRig_RT_dataExp_Tcycle_Cue1_LED_min.vi"() -> ("output_Tcycle_Cue1_LED_min"=w1852:i32)  [unwired: 11 in]
              n1072 = call "myRIO_BRig_RT_dataExp_Tcycle_Cue1_LED_max.vi"() -> ("output_Tcycle_Cue1_LED_max"=w1851:i32)  [unwired: 11 in]
              n1073 = call "myRIO_BRig_RT_dataExp_Tcycle_Cue1Penalty_LED.vi"() -> ("output_Tcycle_Cue1Penalty_LED"=w1850:i32)  [unwired: 11 in]
              n1074 = call "myRIO_BRig_RT_dataExp_SolenoidProbability_L.vi"() -> ("output_SolenoidProbability_L"=w1862:i32)  [unwired: 11 in]
              n1075 = call "myRIO_BRig_RT_dataExp_SolenoidProbability_R.vi"() -> ("output_SolenoidProbability_R"=w1861:i32)  [unwired: 11 in]
              n1076 = call "myRIO_BRig_RT_dataExp_Cue1Param_AudioLed_Count_NS.vi"() -> ("output_Cue1Param_AudioLed_Count_NS"=w1858:i32)  [unwired: 11 in]
              n1077 = call "myRIO_BRig_RT_dataExp_Cue1Param_AudioLed_Probability_NS.vi"() -> ("output_Cue1Param_AudioLed_Probability_NS"=w1856:i32)  [unwired: 11 in]
              n1078 = call "myRIO_BRig_RT_dataExp_Cue1Param_CueType_NS.vi"() -> ("output_Cue1Param_CueType_NS"=w1854:i32)  [unwired: 11 in]
              n1079 = call "myRIO_BRig_RT_dataExp_nBlock.vi"() -> ("output_nBlock"=w1833:i32)  [unwired: 11 in]
              n1080 = call "myRIO_BRig_RT_dataExp_nTrial.vi"() -> ("output_nTrial"=w1835:i32)  [unwired: 11 in]
              n1081 = call "myRIO_BRig_RT_dataExp_runTime_seconds.vi"() -> ("output_RunTime_minutes"=w1838:i32)  [unwired: 11 in]
              n1082 = call "myRIO_BRig_RT_dataExp_Tcycle_Selection.vi"() -> ("output_Tcycle_Selection"=w1840:i32)  [unwired: 11 in]
              n1083 = local read "Tcycle_CuePenalty_Audio"() -> (w1871:u16)
              n1084 = local read "Tcycle_Cue_Audio_max"() -> (w1863:u16)
              n1085 = local read "Tcycle_Cue_Audio_min"() -> (w1864:u16)
              n1086 = local read "Tcycle_RewardPost"() -> (w1882:u16)
              n1087 = local read "Tcycle_Wrong"() -> (w1880:u16)
              n1088 = local read "Tcycle_Timeout"() -> (w1878:u16)
              n1089 = local read "Tcycle_Selection"() -> (w1839:u16)
              n1090 = local read "Cue1Param_AudioLed_Count_NS"() -> (w1857:u16)
              n1091 = local read "Cue1Param_AudioLed_Probability_NS"() -> (w1855:u16)
              n1092 = local read "Cue1Param_CueType_NS"() -> (w1853:u16)
              n1093 = local read "Tcycle_CuePenalty_LED"() -> (w1847:u16)
              n1094 = local read "SolenoidProbability_R"() -> (w1859:u16)
              n1095 = local read "SolenoidProbability_L"() -> (w1860:u16)
              n1096 = local read "Tcycle_Cue_LED_min"() -> (w1849:u16)
              n1097 = local read "Tcycle_Cue_LED_max"() -> (w1848:u16)
              n1098 = local read "Tcycle_Reward_max_R"() -> (w1843:u16)
              n1099 = call "myRIO_BRig_RT_dataExp_Tcycle_Reward_max_R.vi"() -> ("output_Tcycle_Reward_max_R"=w1844:i32)  [unwired: 11 in]
              n1100 = call "myRIO_BRig_RT_dataExp_Tcycle_Reward_step_R.vi"() -> ("output_Tcycle_Reward_step_R"=w1842:i32)  [unwired: 11 in]
              n1101 = local read "Tcycle_Reward_step_R"() -> (w1841:u16)
              n1102 = Replace Array Subset(array=w1885, new element #1=u16 0, index #1=w1833, new element #2=u16 0, index #2=w1835, new element #3=u16 0, index #3=w1838, new element #4=w1839, index #4=w1840, new element #5=w1882, index #5=w1883, new element #6=w1880, index #6=w1881, new element #7=w1878, index #7=w1879, new element #8=w1864, index #8=w1877, new element #9=w1863, index #9=w1876, new element #10=w1871, index #10=w1875, new element #11=w1860, index #11=w1862, new element #12=w1859, index #12=w1861, new element #13=w1857, index #13=w1858, new element #14=w1855, index #14=w1856, new element #15=w1853, index #15=w1854, new element #16=w1849, index #16=w1852, new element #17=w1848, index #17=w1851, new element #18=w1847, index #18=w1850, new element #19=w1845, index #19=w1846, new element #20=w1843, index #20=w1844, new element #21=w1841, index #21=w1842) -> (w1884:u16[])
            }
            frame "saveSettings3" {
              w1897 = 100.0 ("y")
              n1103 = call "myRIO_BRig_RT_dataExp_laser1_Freq.vi"() -> ("output_laser1_Freq"=w1930:i32)  [unwired: 11 in]
              n1104 = call "myRIO_BRig_RT_dataExp_laser1_Tpeak.vi"() -> ("output_laser1_Tpeak"=w1925:i32)  [unwired: 11 in]
              n1105 = call "myRIO_BRig_RT_dataExp_laser1_Tshutter.vi"() -> ("output_laser1_Tshutter"=w1920:i32)  [unwired: 11 in]
              n1106 = call "myRIO_BRig_RT_dataExp_FPGA_f_count2ms.vi"() -> ("output_FPGA_f_count2ms"=w1915:i32)  [unwired: 11 in]
              n1107 = call "myRIO_BRig_RT_dataExp_laser1_Power_min.vi"() -> ("output_laser1_Power_min"=w1910:i32)  [unwired: 11 in]
              n1108 = call "myRIO_BRig_RT_dataExp_laser1_Power_max.vi"() -> ("output_laser1_Power_max"=w1903:i32)  [unwired: 11 in]
              n1109 = call "myRIO_BRig_RT_dataExp_laser1_Power_step.vi"() -> ("output_laser1_Power_step"=w1902:i32)  [unwired: 11 in]
              n1110 = call "myRIO_BRig_RT_dataExp_laser1_duration.vi"() -> ("output_laser1_duration"=w1905:i32)  [unwired: 11 in]
              n1111 = local read "Laser_Tshutter_l1"() -> (w1917:dbl)
              n1112 = local read "Laser_Tpeak_l1"() -> (w1922:dbl)
              n1113 = local read "Laser_power_max_l1"() -> (w1896:dbl)
              n1114 = local read "Laser_power_step_l1"() -> (w1895:dbl)
              n1115 = local read "Laser_power_min_l1"() -> (w1907:dbl)
              n1116 = local read "Laser_Freq_l1"() -> (w1929:dbl)
              n1117 = call "myRIO_BRig_RT_dataExp_BUR_min.vi"() -> ("output_BUR_min"=w1945:i32)  [unwired: 11 in]
              n1118 = call "myRIO_BRig_RT_dataExp_BUR_max.vi"() -> ("output_BUR_max"=w1943:i32)  [unwired: 11 in]
              n1119 = call "myRIO_BRig_RT_dataExp_Audio_sp__L.vi"() -> ("output_Audio_sp__L"=w1940:i32)  [unwired: 11 in]
              n1120 = call "myRIO_BRig_RT_dataExp_Audio_sp__R.vi"() -> ("output_Audio_sp__R"=w1939:i32)  [unwired: 11 in]
              n1121 = local read "FPGA_count2ms"() -> (w1912:dbl)
              n1122 = local read "sp_LeftSpout"() -> (w1938:u16)
              n1123 = local read "BUR_max"() -> (w1942:u16)
              n1124 = local read "sp_RightSpout"() -> (w1937:u16)
              n1125 = local read "BUR_min"() -> (w1944:u16)
              n1126 = Multiply(x=w1929, y=w1897) -> (x*y=w1928:dbl)
              n1127 = Multiply(x=w1922, y=w1897) -> (x*y=w1924:dbl)
              n1128 = Multiply(x=w1917, y=w1897) -> (x*y=w1919:dbl)
              n1129 = Multiply(x=w1912, y=w1897) -> (x*y=w1914:dbl)
              n1130 = Multiply(x=w1907, y=w1897) -> (x*y=w1909:dbl)
              n1131 = Multiply(x=w1896, y=w1897) -> (x*y=w1901:dbl)
              n1132 = Multiply(x=w1895, y=w1897) -> (x*y=w1899:dbl)
              n1133 = Round To Nearest(number=w1928) -> (nearest integer value=w1927:dbl)
              n1134 = Round To Nearest(number=w1924) -> (nearest integer value=w1923:dbl)
              n1135 = Round To Nearest(number=w1919) -> (nearest integer value=w1918:dbl)
              n1136 = Round To Nearest(number=w1914) -> (nearest integer value=w1913:dbl)
              n1137 = Round To Nearest(number=w1909) -> (nearest integer value=w1908:dbl)
              n1138 = Round To Nearest(number=w1901) -> (nearest integer value=w1900:dbl)
              n1139 = Round To Nearest(number=w1899) -> (nearest integer value=w1898:dbl)
              n1140 = To Unsigned Word Integer(number=w1927) -> (unsigned 16bit integer=w1926:u16)
              n1141 = To Unsigned Word Integer(number=w1923) -> (unsigned 16bit integer=w1921:u16)
              n1142 = To Unsigned Word Integer(number=w1918) -> (unsigned 16bit integer=w1916:u16)
              n1143 = To Unsigned Word Integer(number=w1913) -> (unsigned 16bit integer=w1911:u16)
              n1144 = To Unsigned Word Integer(number=w1908) -> (unsigned 16bit integer=w1906:u16)
              n1145 = To Unsigned Word Integer(number=w1900) -> (unsigned 16bit integer=w1894:u16)
              n1146 = To Unsigned Word Integer(number=w1898) -> (unsigned 16bit integer=w1893:u16)
              n1147 = local read "Laser_duration_l1"() -> (w1904:u16)
              n1148 = Replace Array Subset(array=w1946, new element #1=w1944, index #1=w1945, new element #2=w1942, index #2=w1943, new element #3=w1938, index #3=w1940, new element #4=w1937, index #4=w1939, new element #5=w1926, index #5=w1930, new element #6=w1921, index #6=w1925, new element #7=w1916, index #7=w1920, new element #8=w1911, index #8=w1915, new element #9=w1906, index #9=w1910, new element #10=w1894, index #10=w1903, new element #11=w1893, index #11=w1902, new element #12=w1904, index #12=w1905) -> (w1941:u16[])
            }
            frame "saveSettings4" {
              w1966 = 100.0 ("y")
              n1149 = call "myRIO_BRig_RT_dataExp_laser2_Freq.vi"() -> ("output_laser2_Freq"=w1955:i32)  [unwired: 11 in]
              n1150 = call "myRIO_BRig_RT_dataExp_laser2_Tpeak.vi"() -> ("output_laser2_Tpeak"=w1957:i32)  [unwired: 11 in]
              n1151 = call "myRIO_BRig_RT_dataExp_laser2_Tshutter.vi"() -> ("output_laser2_Tshutter"=w1959:i32)  [unwired: 11 in]
              n1152 = call "myRIO_BRig_RT_dataExp_laser2_Power_min.vi"() -> ("output_laser2_Power_min"=w1974:i32)  [unwired: 11 in]
              n1153 = call "myRIO_BRig_RT_dataExp_laser2_Power_max.vi"() -> ("output_laser2_Power_max"=w1973:i32)  [unwired: 11 in]
              n1154 = call "myRIO_BRig_RT_dataExp_laser2_Power_step.vi"() -> ("output_laser2_Power_step"=w1972:i32)  [unwired: 11 in]
              n1155 = call "myRIO_BRig_RT_dataExp_laser2_duration.vi"() -> ("output_laser2_duration"=w1971:i32)  [unwired: 11 in]
              n1156 = call "myRIO_BRig_RT_dataExp_CueLed_Freq.vi"() -> ("output_CueLed_Freq"=w1963:i32)  [unwired: 11 in]
              n1157 = call "myRIO_BRig_RT_dataExp_CueLed_Tpeak.vi"() -> ("output_CueLed_Tpeak"=w1962:i32)  [unwired: 11 in]
              n1158 = local read "Laser_Tshutter_l2"() -> (w1989:dbl)
              n1159 = local read "Laser_Tpeak_l2"() -> (w1992:dbl)
              n1160 = local read "Laser_power_max_l2"() -> (w1979:dbl)
              n1161 = local read "Laser_power_step_l2"() -> (w1978:dbl)
              n1162 = local read "Laser_power_min_l2"() -> (w1986:dbl)
              n1163 = local read "Laser_Freq_l2"() -> (w1997:dbl)
              n1164 = local read "CueLed_Tpeak"() -> (w1964:dbl)
              n1165 = local read "CueLed_Freq"() -> (w1965:dbl)
              n1166 = Multiply(x=w1997, y=w1966) -> (x*y=w1996:dbl)
              n1167 = Multiply(x=w1992, y=w1966) -> (x*y=w1994:dbl)
              n1168 = Multiply(x=w1989, y=w1966) -> (x*y=w1991:dbl)
              n1169 = Multiply(x=w1986, y=w1966) -> (x*y=w1988:dbl)
              n1170 = Multiply(x=w1979, y=w1966) -> (x*y=w1983:dbl)
              n1171 = Multiply(x=w1978, y=w1966) -> (x*y=w1981:dbl)
              n1172 = Multiply(x=w1965, y=w1966) -> (x*y=w1967:dbl)
              n1173 = Multiply(x=w1964, y=w1966) -> (x*y=w1968:dbl)
              n1174 = Round To Nearest(number=w1996) -> (nearest integer value=w1995:dbl)
              n1175 = Round To Nearest(number=w1994) -> (nearest integer value=w1993:dbl)
              n1176 = Round To Nearest(number=w1991) -> (nearest integer value=w1990:dbl)
              n1177 = Round To Nearest(number=w1988) -> (nearest integer value=w1987:dbl)
              n1178 = Round To Nearest(number=w1983) -> (nearest integer value=w1982:dbl)
              n1179 = Round To Nearest(number=w1981) -> (nearest integer value=w1980:dbl)
              n1180 = Round To Nearest(number=w1967) -> (nearest integer value=w1970:dbl)
              n1181 = Round To Nearest(number=w1968) -> (nearest integer value=w1969:dbl)
              n1182 = To Unsigned Word Integer(number=w1995) -> (unsigned 16bit integer=w1954:u16)
              n1183 = To Unsigned Word Integer(number=w1993) -> (unsigned 16bit integer=w1956:u16)
              n1184 = To Unsigned Word Integer(number=w1990) -> (unsigned 16bit integer=w1958:u16)
              n1185 = To Unsigned Word Integer(number=w1987) -> (unsigned 16bit integer=w1985:u16)
              n1186 = To Unsigned Word Integer(number=w1982) -> (unsigned 16bit integer=w1977:u16)
              n1187 = To Unsigned Word Integer(number=w1980) -> (unsigned 16bit integer=w1976:u16)
              n1188 = To Unsigned Word Integer(number=w1970) -> (unsigned 16bit integer=w1961:u16)
              n1189 = To Unsigned Word Integer(number=w1969) -> (unsigned 16bit integer=w1960:u16)
              n1190 = local read "Laser_duration_l2"() -> (w1984:u16)
              n1191 = Replace Array Subset(array=w2005, new element #1=w1954, index #1=w1955, new element #2=w1956, index #2=w1957, new element #3=w1958, index #3=w1959, new element #4=w1985, index #4=w1974, new element #5=w1977, index #5=w1973, new element #6=w1976, index #6=w1972, new element #7=w1984, index #7=w1971, new element #8=w1961, index #8=w1963, new element #9=w1960, index #9=w1962) -> (w2004:u16[])
            }
            frame "saveSettings_LC_ENL_l1" {
              # "Selection First"
              # "Count"
              # "Tdelay"
              # "Probability"
              # "OnOff"
              # "Block"
              # "delayOpt"
              # "Count"
              # "Tdelay"
              # "Probability"
              # "OnOff"
              # "Block"
              # "ENL1 All"
              # "delayOpt"
              # "Count"
              # "Tdelay"
              # "Probability"
              # "OnOff"
              # "Block"
              # "ENL1 First"
              n1192 = local read "LC_ENL1_delayOpt_Switch_l1"() -> (w2043:bool)
              n1193 = call "myRIO_BRig_RT_dataLC_ENL1_Block_NS_l1.vi"() -> ("output_ENL1_All_Block"=w2040:i32)  [unwired: 11 in]
              n1194 = call "myRIO_BRig_RT_dataLC_ENL1_OnOff_NS_l1.vi"() -> ("output_ENL1_OnOff_NS_l1"=w2030:i32)  [unwired: 11 in]
              n1195 = call "myRIO_BRig_RT_dataLC_ENL1_Probability_NS_l1.vi"() -> ("output_ENL1_Probability_NS_l1"=w2029:i32)  [unwired: 11 in]
              n1196 = call "myRIO_BRig_RT_dataLC_ENL1_Tdelay_NS_l1.vi"() -> ("output_ENL1_Tdelay_NS_l1"=w2028:i32)  [unwired: 11 in]
              n1197 = call "myRIO_BRig_RT_dataLC_ENL1_Count_NS_l1.vi"() -> ("output_ENL1_Count_NS_l1"=w2027:i32)  [unwired: 11 in]
              n1198 = call "myRIO_BRig_RT_dataLC_ENL1_delayOpt_NS_l1.vi"() -> ("output_ENL1_delayOpt_NS_l1"=w2026:i32)  [unwired: 11 in]
              n1199 = call "myRIO_BRig_RT_dataLC_ENL1_Block_Switch_l1.vi"() -> ("output_ENL1_Block_Switch_l1"=w2062:i32)  [unwired: 11 in]
              n1200 = call "myRIO_BRig_RT_dataLC_ENL1_OnOff_Switch_l1.vi"() -> ("output_ENL1_OnOff_Switch_l1"=w2060:i32)  [unwired: 11 in]
              n1201 = call "myRIO_BRig_RT_dataLC_ENL1_Probability_Switch_l1.vi"() -> ("output_ENL1_Probability_Switch_l1"=w2056:i32)  [unwired: 11 in]
              n1202 = call "myRIO_BRig_RT_dataLC_ENL1_Tdelay_Switch_l1.vi"() -> ("output_ENL1_Tdelay_Switch_l1"=w2054:i32)  [unwired: 11 in]
              n1203 = call "myRIO_BRig_RT_dataLC_ENL1_Count_Switch_l1.vi"() -> ("output_ENL1_Count_Switch_l1"=w2052:i32)  [unwired: 11 in]
              n1204 = call "myRIO_BRig_RT_dataLC_ENL1_delayOpt_Switch_l1.vi"() -> ("output_ENL1_delayOpt_Switch_l1"=w2042:i32)  [unwired: 11 in]
              n1205 = local read "LC_ENL1_Count_Switch_l1"() -> (w2051:u16)
              n1206 = local read "LC_ENL1_Probability_Switch_l1"() -> (w2055:u16)
              n1207 = local read "LC_ENL1_Block_Switch_l1"() -> (w2061:u16)
              n1208 = local read "LC_ENL1_Tdelay_Switch_l1"() -> (w2053:u16)
              n1209 = local read "LC_ENL1_OnOff_Switch_l1"() -> (w2059:bool)
              n1210 = call "myRIO_BRig_RT_dataLC_Selection_Block_Switch_l1.vi"() -> ("output_Selection_Block_Switch_l1"=w2024:i32)  [unwired: 11 in]
              n1211 = call "myRIO_BRig_RT_dataLC_Selection_OnOff_Switch_l1.vi"() -> ("output_Selection_OnOff_Switch_l1"=w2023:i32)  [unwired: 11 in]
              n1212 = call "myRIO_BRig_RT_dataLC_Selection_Probability_Switch_l1.vi"() -> ("output_Selection_Probability_Switch_l1"=w2022:i32)  [unwired: 11 in]
              n1213 = call "myRIO_BRig_RT_dataLC_Selection_Tdelay_Switch_l1.vi"() -> ("output_Selection_Tdelay_Switch_l1"=w2021:i32)  [unwired: 11 in]
              n1214 = call "myRIO_BRig_RT_dataLC_Selection_Count_Switch_l1.vi"() -> ("output_Selection_Count_Switch_l1"=w2020:i32)  [unwired: 11 in]
              n1215 = local read "LC_ENL1_OnOff_NS_l1"() -> (w2036:bool)
              n1216 = local read "LC_ENL1_Probability_NS_l1"() -> (w2034:u16)
              n1217 = local read "LC_ENL1_delayOpt_NS_l1"() -> (w2032:bool)
              n1218 = local read "LC_Sel_Probability_Switch_l1"() -> (w2015:u16)
              n1219 = local read "LC_ENL1_Tdelay_NS_l1"() -> (w2025:u16)
              n1220 = local read "LC_ENL1_Block_NS_l1"() -> (w2037:u16)
              n1221 = local read "LC_ENL1_Count_NS_l1"() -> (w2033:u16)
              n1222 = local read "LC_Sel_Tdelay_Switch_l1"() -> (w2014:u16)
              n1223 = local read "LC_Sel_OnOff_Switch_l1"() -> (w2018:bool)
              n1224 = local read "LC_Sel_Count_Switch_l1"() -> (w2013:u16)
              n1225 = local read "LC_Sel_Block_Switch_l1"() -> (w2017:u16)
              n1226 = Boolean To (0,1)(Boolean=w2043) -> (0, 1=w2044:i16)
              n1227 = Boolean To (0,1)(Boolean=w2059) -> (0, 1=w2058:i16)
              n1228 = Boolean To (0,1)(Boolean=w2036) -> (0, 1=w2039:i16)
              n1229 = To Unsigned Word Integer(number=w2044) -> (unsigned 16bit integer=w2041:u16)
              n1230 = To Unsigned Word Integer(number=w2058) -> (unsigned 16bit integer=w2057:u16)
              n1231 = Boolean To (0,1)(Boolean=w2032) -> (0, 1=w2038:i16)
              n1232 = To Unsigned Word Integer(number=w2039) -> (unsigned 16bit integer=w2035:u16)
              n1233 = Boolean To (0,1)(Boolean=w2018) -> (0, 1=w2019:i16)
              n1234 = To Unsigned Word Integer(number=w2038) -> (unsigned 16bit integer=w2031:u16)
              n1235 = To Unsigned Word Integer(number=w2019) -> (unsigned 16bit integer=w2016:u16)
              n1236 = Replace Array Subset(array=w2063, new element #1=w2061, index #1=w2062, new element #2=w2057, index #2=w2060, new element #3=w2055, index #3=w2056, new element #4=w2053, index #4=w2054, new element #5=w2051, index #5=w2052, new element #6=w2041, index #6=w2042, new element #7=w2037, index #7=w2040, new element #8=w2035, index #8=w2030, new element #9=w2034, index #9=w2029, new element #10=w2025, index #10=w2028, new element #11=w2033, index #11=w2027, new element #12=w2031, index #12=w2026, new element #13=w2017, index #13=w2024, new element #14=w2016, index #14=w2023, new element #15=w2015, index #15=w2022, new element #16=w2014, index #16=w2021, new element #17=w2013, index #17=w2020) -> (w2064:u16[])
            }
            frame "saveSettings_LC_ENL_l2" {
              # "Selection First"
              # "Count"
              # "Tdelay"
              # "Probability"
              # "OnOff"
              # "Block"
              # "delayOpt"
              # "Count"
              # "Tdelay"
              # "Probability"
              # "OnOff"
              # "Block"
              # "ENL1 All"
              # "delayOpt"
              # "Count"
              # "Tdelay"
              # "Probability"
              # "OnOff"
              # "Block"
              # "ENL1 First"
              n1237 = call "myRIO_BRig_RT_dataLC_ENL1_Block_Switch_l2.vi"() -> ("output_ENL1_Block_Switch_l2"=w2083:i32)  [unwired: 11 in]
              n1238 = call "myRIO_BRig_RT_dataLC_ENL1_OnOff_Switch_l2.vi"() -> ("output_ENL1_OnOff_Switch_l2"=w2084:i32)  [unwired: 11 in]
              n1239 = call "myRIO_BRig_RT_dataLC_ENL1_Probability_Switch_l2.vi"() -> ("output_ENL1_Probability_Switch_l2"=w2085:i32)  [unwired: 11 in]
              n1240 = call "myRIO_BRig_RT_dataLC_ENL1_Tdelay_Switch_l2.vi"() -> ("output_ENL1_Tdelay_Switch_l2"=w2086:i32)  [unwired: 11 in]
              n1241 = call "myRIO_BRig_RT_dataLC_ENL1_Count_Switch_l2.vi"() -> ("output_ENL1_Count_Switch_l2"=w2087:i32)  [unwired: 11 in]
              n1242 = call "myRIO_BRig_RT_dataLC_ENL1_delayOpt_Switch_l2.vi"() -> ("output_ENL1_delayOpt_Switch_l2"=w2088:i32)  [unwired: 11 in]
              n1243 = local read "LC_ENL1_delayOpt_Switch_l2"() -> (w2108:bool)
              n1244 = call "myRIO_BRig_RT_dataLC_ENL1_Block_NS_l2.vi"() -> ("output_ENL1_Block_NS_l2"=w2077:i32)  [unwired: 11 in]
              n1245 = call "myRIO_BRig_RT_dataLC_ENL1_OnOff_NS_l2.vi"() -> ("output_ENL1_OnOff_NS_l2"=w2078:i32)  [unwired: 11 in]
              n1246 = call "myRIO_BRig_RT_dataLC_ENL1_Probability_NS_l2.vi"() -> ("output_ENL1_Probability_NS_l2"=w2079:i32)  [unwired: 11 in]
              n1247 = call "myRIO_BRig_RT_dataLC_ENL1_Tdelay_NS_l2.vi"() -> ("output_ENL1_Tdelay_NS_l2"=w2080:i32)  [unwired: 11 in]
              n1248 = call "myRIO_BRig_RT_dataLC_ENL1_Count_NS_l2.vi"() -> ("output_ENL1_Count_NS_l2"=w2081:i32)  [unwired: 11 in]
              n1249 = call "myRIO_BRig_RT_dataLC_ENL1_delayOpt_NS_l2.vi"() -> ("output_ENL1_delayOpt_NS_l2"=w2082:i32)  [unwired: 11 in]
              n1250 = local read "LC_ENL1_Count_Switch_l2"() -> (w2116:u16)
              n1251 = local read "LC_ENL1_Probability_Switch_l2"() -> (w2118:u16)
              n1252 = local read "LC_ENL1_Block_Switch_l2"() -> (w2122:u16)
              n1253 = local read "LC_ENL1_Tdelay_Switch_l2"() -> (w2117:u16)
              n1254 = local read "LC_ENL1_OnOff_Switch_l2"() -> (w2121:bool)
              n1255 = call "myRIO_BRig_RT_dataLC_Selection_Block_Switch_l2.vi"() -> ("output_Selection_Block_Switch_l2"=w2076:i32)  [unwired: 11 in]
              n1256 = call "myRIO_BRig_RT_dataLC_Selection_OnOff_Switch_l2.vi"() -> ("output_Selection_OnOff_Switch_l2"=w2075:i32)  [unwired: 11 in]
              n1257 = call "myRIO_BRig_RT_dataLC_Selection_Probability_Switch_l2.vi"() -> ("output_Selection_Probability_Switch_l1"=w2074:i32)  [unwired: 11 in]
              n1258 = call "myRIO_BRig_RT_dataLC_Selection_Tdelay_Switch_l2.vi"() -> ("output_Selection_Tdelay_Switch_l2"=w2073:i32)  [unwired: 11 in]
              n1259 = call "myRIO_BRig_RT_dataLC_Selection_Count_Switch_l2.vi"() -> ("output_Selection_Count_Switch_l2"=w2072:i32)  [unwired: 11 in]
              n1260 = local read "LC_ENL1_OnOff_NS_l2"() -> (w2103:bool)
              n1261 = local read "LC_ENL1_Probability_NS_l2"() -> (w2101:u16)
              n1262 = local read "LC_ENL1_delayOpt_NS_l2"() -> (w2099:bool)
              n1263 = local read "LC_Sel_Probability_Switch_l2"() -> (w2092:u16)
              n1264 = local read "LC_ENL1_Tdelay_NS_l2"() -> (w2097:u16)
              n1265 = local read "LC_ENL1_Block_NS_l2"() -> (w2104:u16)
              n1266 = local read "LC_ENL1_Count_NS_l2"() -> (w2100:u16)
              n1267 = local read "LC_Sel_Tdelay_Switch_l2"() -> (w2091:u16)
              n1268 = local read "LC_Sel_OnOff_Switch_l2"() -> (w2095:bool)
              n1269 = local read "LC_Sel_Count_Switch_l2"() -> (w2090:u16)
              n1270 = local read "LC_Sel_Block_Switch_l2"() -> (w2094:u16)
              n1271 = Boolean To (0,1)(Boolean=w2108) -> (0, 1=w2109:i16)
              n1272 = Boolean To (0,1)(Boolean=w2121) -> (0, 1=w2120:i16)
              n1273 = Boolean To (0,1)(Boolean=w2103) -> (0, 1=w2106:i16)
              n1274 = To Unsigned Word Integer(number=w2109) -> (unsigned 16bit integer=w2107:u16)
              n1275 = To Unsigned Word Integer(number=w2120) -> (unsigned 16bit integer=w2119:u16)
              n1276 = Boolean To (0,1)(Boolean=w2099) -> (0, 1=w2105:i16)
              n1277 = To Unsigned Word Integer(number=w2106) -> (unsigned 16bit integer=w2102:u16)
              n1278 = Boolean To (0,1)(Boolean=w2095) -> (0, 1=w2096:i16)
              n1279 = To Unsigned Word Integer(number=w2105) -> (unsigned 16bit integer=w2098:u16)
              n1280 = To Unsigned Word Integer(number=w2096) -> (unsigned 16bit integer=w2093:u16)
              n1281 = Replace Array Subset(array=w2123, new element #1=w2122, index #1=w2083, new element #2=w2119, index #2=w2084, new element #3=w2118, index #3=w2085, new element #4=w2117, index #4=w2086, new element #5=w2116, index #5=w2087, new element #6=w2107, index #6=w2088, new element #7=w2104, index #7=w2077, new element #8=w2102, index #8=w2078, new element #9=w2101, index #9=w2079, new element #10=w2097, index #10=w2080, new element #11=w2100, index #11=w2081, new element #12=w2098, index #12=w2082, new element #13=w2094, index #13=w2076, new element #14=w2093, index #14=w2075, new element #15=w2092, index #15=w2074, new element #16=w2091, index #16=w2073, new element #17=w2090, index #17=w2072) -> (w2124:u16[])
            }
            frame "saveSettings_LC_Cue_l1" {
              # "Selection All"
              # "Count"
              # "Tdelay"
              # "Probability"
              # "OnOff"
              # "Block"
              # "delayOpt"
              # "Count"
              # "Tdelay"
              # "Probability"
              # "OnOff"
              # "Block"
              # "Cue1 All"
              # "delayOpt"
              # "Count"
              # "Tdelay"
              # "Probability"
              # "OnOff"
              # "Block"
              # "Cue1 First"
              n1282 = call "myRIO_BRig_RT_dataLC_Cue1_delayOpt_Switch_l1.vi"() -> ("output_Cue1_delayOpt_Switch_l1"=w2163:i32)  [unwired: 11 in]
              n1283 = call "myRIO_BRig_RT_dataLC_Cue1_Block_Switch_l1.vi"() -> ("output_Cue1_Block_Switch_l1"=w2182:i32)  [unwired: 11 in]
              n1284 = call "myRIO_BRig_RT_dataLC_Cue1_OnOff_Switch_l1.vi"() -> ("output_Cue1_OnOff_Switch_l1"=w2180:i32)  [unwired: 11 in]
              n1285 = call "myRIO_BRig_RT_dataLC_Cue1_Probability_Switch_l1.vi"() -> ("output_Cue1_Probability_Switch_l1"=w2176:i32)  [unwired: 11 in]
              n1286 = call "myRIO_BRig_RT_dataLC_Cue1_Tdelay_Switch_l1.vi"() -> ("output_Cue1_Tdelay_Switch_l1"=w2174:i32)  [unwired: 11 in]
              n1287 = call "myRIO_BRig_RT_dataLC_Cue1_Count_Switch_l1.vi"() -> ("output_Cue1_Count_Switch_l1"=w2172:i32)  [unwired: 11 in]
              n1288 = local read "LC_Cue1_delayOpt_Switch_l1"() -> (w2162:bool)
              n1289 = call "myRIO_BRig_RT_dataLC_Cue1_Block_NS_l1.vi"() -> ("output_Cue1_Block_NS_l1"=w2160:i32)  [unwired: 11 in]
              n1290 = call "myRIO_BRig_RT_dataLC_Cue1_OnOff_NS_l1.vi"() -> ("output_Cue1_OnOff_NS_l1"=w2159:i32)  [unwired: 11 in]
              n1291 = call "myRIO_BRig_RT_dataLC_Cue1_Probability_NS_l1.vi"() -> ("output_Cue1_l1_All_Probability"=w2158:i32)  [unwired: 11 in]
              n1292 = call "myRIO_BRig_RT_dataLC_Cue1_Tdelay_NS_l1.vi"() -> ("output_Cue1_Tdelay_NS_l1"=w2157:i32)  [unwired: 11 in]
              n1293 = call "myRIO_BRig_RT_dataLC_Cue1_Count_NS_l1.vi"() -> ("output_Cue1_Count_NS_l1"=w2156:i32)  [unwired: 11 in]
              n1294 = call "myRIO_BRig_RT_dataLC_Cue1_delayOpt_NS_l1.vi"() -> ("output_Cue1_delayOpt_NS_l1"=w2155:i32)  [unwired: 11 in]
              n1295 = local read "LC_Cue1_Count_Switch_l1"() -> (w2171:u16)
              n1296 = local read "LC_Cue1_Probability_Switch_l1"() -> (w2175:u16)
              n1297 = local read "LC_Cue1_Block_Switch_l1"() -> (w2181:u16)
              n1298 = local read "LC_Cue1_Tdelay_Switch_l1"() -> (w2173:u16)
              n1299 = local read "LC_Cue1_OnOff_Switch_l1"() -> (w2179:bool)
              n1300 = local read "LC_Cue1_OnOff_NS_l1"() -> (w2151:bool)
              n1301 = call "myRIO_BRig_RT_dataLC_Selection_Block_NS_l1.vi"() -> ("output_Selection_Block_NS_l1"=w2144:i32)  [unwired: 11 in]
              n1302 = call "myRIO_BRig_RT_dataLC_Selection_OnOff_NS_l1.vi"() -> ("output_Selection_OnOff_NS_l1"=w2143:i32)  [unwired: 11 in]
              n1303 = call "myRIO_BRig_RT_dataLC_Selection_Probability_NS_l1.vi"() -> ("output_Selection_Probability_NS_l1"=w2142:i32)  [unwired: 11 in]
              n1304 = call "myRIO_BRig_RT_dataLC_Selection_Tdelay_NS_l1.vi"() -> ("output_Selection_Tdelay_NS_l1"=w2141:i32)  [unwired: 11 in]
              n1305 = call "myRIO_BRig_RT_dataLC_Selection_Count_NS_l1.vi"() -> ("output_Selection_Count_NS_l1"=w2134:i32)  [unwired: 11 in]
              n1306 = local read "LC_Cue1_delayOpt_NS_l1"() -> (w2152:bool)
              n1307 = local read "LC_Cue1_Probability_NS_l1"() -> (w2148:u16)
              n1308 = local read "LC_Cue1_Tdelay_NS_l1"() -> (w2147:u16)
              n1309 = local read "LC_Cue1_Count_NS_l1"() -> (w2146:u16)
              n1310 = local read "LC_Cue1_Block_NS_l1"() -> (w2150:u16)
              n1311 = local read "LC_Sel_Probability_NS_l1"() -> (w2136:u16)
              n1312 = local read "LC_Sel_Tdelay_NS_l1"() -> (w2135:u16)
              n1313 = local read "LC_Sel_OnOff_NS_l1"() -> (w2138:bool)
              n1314 = local read "LC_Sel_Count_NS_l1"() -> (w2133:u16)
              n1315 = local read "LC_Sel_Block_NS_l1"() -> (w2140:u16)
              n1316 = Boolean To (0,1)(Boolean=w2162) -> (0, 1=w2164:i16)
              n1317 = Boolean To (0,1)(Boolean=w2179) -> (0, 1=w2178:i16)
              n1318 = Boolean To (0,1)(Boolean=w2151) -> (0, 1=w2154:i16)
              n1319 = To Unsigned Word Integer(number=w2164) -> (unsigned 16bit integer=w2161:u16)
              n1320 = To Unsigned Word Integer(number=w2178) -> (unsigned 16bit integer=w2177:u16)
              n1321 = To Unsigned Word Integer(number=w2154) -> (unsigned 16bit integer=w2149:u16)
              n1322 = Boolean To (0,1)(Boolean=w2152) -> (0, 1=w2153:i16)
              n1323 = Boolean To (0,1)(Boolean=w2138) -> (0, 1=w2139:i16)
              n1324 = To Unsigned Word Integer(number=w2153) -> (unsigned 16bit integer=w2145:u16)
              n1325 = To Unsigned Word Integer(number=w2139) -> (unsigned 16bit integer=w2137:u16)
              n1326 = Replace Array Subset(array=w2183, new element #1=w2181, index #1=w2182, new element #2=w2177, index #2=w2180, new element #3=w2175, index #3=w2176, new element #4=w2173, index #4=w2174, new element #5=w2171, index #5=w2172, new element #6=w2161, index #6=w2163, new element #7=w2150, index #7=w2160, new element #8=w2149, index #8=w2159, new element #9=w2148, index #9=w2158, new element #10=w2147, index #10=w2157, new element #11=w2146, index #11=w2156, new element #12=w2145, index #12=w2155, new element #13=w2140, index #13=w2144, new element #14=w2137, index #14=w2143, new element #15=w2136, index #15=w2142, new element #16=w2135, index #16=w2141, new element #17=w2133, index #17=w2134) -> (w2184:u16[])
            }
            frame "saveSettings_LC_Cue_l2" {
              # "Selection All"
              # "Count"
              # "Tdelay"
              # "Probability"
              # "OnOff"
              # "Block"
              # "delayOpt"
              # "Count"
              # "Tdelay"
              # "Probability"
              # "OnOff"
              # "Block"
              # "Cue1 All"
              # "delayOpt"
              # "Count"
              # "Tdelay"
              # "Probability"
              # "OnOff"
              # "Block"
              # "Cue1 First"
              n1327 = call "myRIO_BRig_RT_dataLC_Cue1_delayOpt_Switch_l2.vi"() -> ("output_Cue1_delayOpt_Switch_l2"=w2223:i32)  [unwired: 11 in]
              n1328 = call "myRIO_BRig_RT_dataLC_Cue1_Block_Switch_l2.vi"() -> ("output_Cue1_Block_Switch_l2"=w2242:i32)  [unwired: 11 in]
              n1329 = call "myRIO_BRig_RT_dataLC_Cue1_OnOff_Switch_l2.vi"() -> ("output_Cue1_OnOff_Switch_l2"=w2240:i32)  [unwired: 11 in]
              n1330 = call "myRIO_BRig_RT_dataLC_Cue1_Probability_Switch_l2.vi"() -> ("output_Cue1_l2_First_Probability"=w2236:i32)  [unwired: 11 in]
              n1331 = call "myRIO_BRig_RT_dataLC_Cue1_Tdelay_Switch_l2.vi"() -> ("output_Cue1_Tdelay_Switch_l2"=w2234:i32)  [unwired: 11 in]
              n1332 = call "myRIO_BRig_RT_dataLC_Cue1_Count_Switch_l2.vi"() -> ("output_Cue1_Count_Switch_l2"=w2232:i32)  [unwired: 11 in]
              n1333 = local read "LC_Cue1_delayOpt_Switch_l2"() -> (w2222:bool)
              n1334 = call "myRIO_BRig_RT_dataLC_Cue1_Block_NS_l2.vi"() -> ("output_Cue1_Block_NS_l2"=w2220:i32)  [unwired: 11 in]
              n1335 = call "myRIO_BRig_RT_dataLC_Cue1_OnOff_NS_l2.vi"() -> ("output_Cue1_OnOff_NS_l2"=w2219:i32)  [unwired: 11 in]
              n1336 = call "myRIO_BRig_RT_dataLC_Cue1_Probability_NS_l2.vi"() -> ("output_Cue1_l2_All_Probability"=w2218:i32)  [unwired: 11 in]
              n1337 = call "myRIO_BRig_RT_dataLC_Cue1_Tdelay_NS_l2.vi"() -> ("output_Cue1_Tdelay_NS_l2"=w2217:i32)  [unwired: 11 in]
              n1338 = call "myRIO_BRig_RT_dataLC_Cue1_Count_NS_l2.vi"() -> ("output_Cue1_Count_NS_l2"=w2216:i32)  [unwired: 11 in]
              n1339 = call "myRIO_BRig_RT_dataLC_Cue1_delayOpt_NS_l2.vi"() -> ("output_Cue1_delayOpt_NS_l2"=w2215:i32)  [unwired: 11 in]
              n1340 = local read "LC_Cue1_Count_Switch_l2"() -> (w2231:u16)
              n1341 = local read "LC_Cue1_Probability_Switch_l2"() -> (w2235:u16)
              n1342 = local read "LC_Cue1_Block_Switch_l2"() -> (w2241:u16)
              n1343 = local read "LC_Cue1_Tdelay_Switch_l2"() -> (w2233:u16)
              n1344 = local read "LC_Cue1_OnOff_Switch_l2"() -> (w2239:bool)
              n1345 = local read "LC_Cue1_OnOff_NS_l2"() -> (w2211:bool)
              n1346 = call "myRIO_BRig_RT_dataLC_Selection_Block_NS_l2.vi"() -> ("output_Selection_Block_NS_l2"=w2196:i32)  [unwired: 11 in]
              n1347 = call "myRIO_BRig_RT_dataLC_Selection_OnOff_NS_l2.vi"() -> ("output_Selection_OnOff_NS_l2"=w2195:i32)  [unwired: 11 in]
              n1348 = call "myRIO_BRig_RT_dataLC_Selection_Probability_NS_l2.vi"() -> ("output_Selection_Probability_NS_l2"=w2194:i32)  [unwired: 11 in]
              n1349 = call "myRIO_BRig_RT_dataLC_Selection_Tdelay_NS_l2.vi"() -> ("output_Selection_Tdelay_NS_l2"=w2193:i32)  [unwired: 11 in]
              n1350 = call "myRIO_BRig_RT_dataLC_Selection_Count_NS_l2.vi"() -> ("output_Selection_Count_NS_l2"=w2192:i32)  [unwired: 11 in]
              n1351 = local read "LC_Cue1_delayOpt_NS_l2"() -> (w2212:bool)
              n1352 = local read "LC_Cue1_Probability_NS_l2"() -> (w2208:u16)
              n1353 = local read "LC_Cue1_Tdelay_NS_l2"() -> (w2207:u16)
              n1354 = local read "LC_Cue1_Count_NS_l2"() -> (w2206:u16)
              n1355 = local read "LC_Cue1_Block_NS_l2"() -> (w2210:u16)
              n1356 = local read "LC_Sel_Probability_NS_l2"() -> (w2200:u16)
              n1357 = local read "LC_Sel_Tdelay_NS_l2"() -> (w2199:u16)
              n1358 = local read "LC_Sel_OnOff_NS_l2"() -> (w2202:bool)
              n1359 = local read "LC_Sel_Count_NS_l2"() -> (w2198:u16)
              n1360 = local read "LC_Sel_Block_NS_l2"() -> (w2204:u16)
              n1361 = Boolean To (0,1)(Boolean=w2222) -> (0, 1=w2224:i16)
              n1362 = Boolean To (0,1)(Boolean=w2239) -> (0, 1=w2238:i16)
              n1363 = Boolean To (0,1)(Boolean=w2211) -> (0, 1=w2214:i16)
              n1364 = To Unsigned Word Integer(number=w2224) -> (unsigned 16bit integer=w2221:u16)
              n1365 = To Unsigned Word Integer(number=w2238) -> (unsigned 16bit integer=w2237:u16)
              n1366 = To Unsigned Word Integer(number=w2214) -> (unsigned 16bit integer=w2209:u16)
              n1367 = Boolean To (0,1)(Boolean=w2212) -> (0, 1=w2213:i16)
              n1368 = Boolean To (0,1)(Boolean=w2202) -> (0, 1=w2203:i16)
              n1369 = To Unsigned Word Integer(number=w2213) -> (unsigned 16bit integer=w2205:u16)
              n1370 = To Unsigned Word Integer(number=w2203) -> (unsigned 16bit integer=w2201:u16)
              n1371 = Replace Array Subset(array=w2243, new element #1=w2241, index #1=w2242, new element #2=w2237, index #2=w2240, new element #3=w2235, index #3=w2236, new element #4=w2233, index #4=w2234, new element #5=w2231, index #5=w2232, new element #6=w2221, index #6=w2223, new element #7=w2210, index #7=w2220, new element #8=w2209, index #8=w2219, new element #9=w2208, index #9=w2218, new element #10=w2207, index #10=w2217, new element #11=w2206, index #11=w2216, new element #12=w2205, index #12=w2215, new element #13=w2204, index #13=w2196, new element #14=w2201, index #14=w2195, new element #15=w2200, index #15=w2194, new element #16=w2199, index #16=w2193, new element #17=w2198, index #17=w2192) -> (w2244:u16[])
            }
            frame "saveSettings6_LC_l1_Other" {
              # "Trial"
              # "Tdelay"
              # "Probability"
              # "OnOff"
              # "Block"
              # "Wrong"
              # "Trial"
              # "Tdelay"
              # "Probability"
              # "OnOff"
              # "Block"
              # "Reward"
              n1372 = call "myRIO_BRig_RT_dataLC_Wrong_Block_l1.vi"() -> ("output_Wrong_Block_l1"=w2269:i32)  [unwired: 11 in]
              n1373 = call "myRIO_BRig_RT_dataLC_Wrong_OnOff_l1.vi"() -> ("output_Wrong_OnOff_l1"=w2268:i32)  [unwired: 11 in]
              n1374 = call "myRIO_BRig_RT_dataLC_Wrong_Probability_l1.vi"() -> ("output_Wrong_Probability_l1"=w2267:i32)  [unwired: 11 in]
              n1375 = call "myRIO_BRig_RT_dataLC_Wrong_Tdelay_l1.vi"() -> ("output_Wrong_Tdelay_l1"=w2266:i32)  [unwired: 11 in]
              n1376 = call "myRIO_BRig_RT_dataLC_Wrong_Trial_l1.vi"() -> ("output_Wrong_Trial_l1"=w2265:i32)  [unwired: 11 in]
              n1377 = call "myRIO_BRig_RT_dataLC_Reward_Block_l1.vi"() -> ("output_Reward_Block_l1"=w2281:i32)  [unwired: 11 in]
              n1378 = call "myRIO_BRig_RT_dataLC_Reward_OnOff_l1.vi"() -> ("output_Reward_OnOff_l1"=w2279:i32)  [unwired: 11 in]
              n1379 = call "myRIO_BRig_RT_dataLC_Reward_Probability_l1.vi"() -> ("output_Reward_Probability_l1"=w2275:i32)  [unwired: 11 in]
              n1380 = call "myRIO_BRig_RT_dataLC_Reward_Tdelay_l1.vi"() -> ("output_Reward_Tdelay_l1"=w2273:i32)  [unwired: 11 in]
              n1381 = call "myRIO_BRig_RT_dataLC_Reward_Trial_l1.vi"() -> ("output_Reward_Trial_l1"=w2271:i32)  [unwired: 11 in]
              n1382 = local read "LC_Wrong_OnOff_l1"() -> (w2263:bool)
              n1383 = local read "LC_Wrong_Probability_l1"() -> (w2260:u16)
              n1384 = local read "LC_Wrong_Block_l1"() -> (w2262:u16)
              n1385 = local read "LC_Wrong_Tdelay_l1"() -> (w2259:u16)
              n1386 = local read "LC_Wrong_Trial_l1"() -> (w2258:u16)
              n1387 = local read "LC_Reward_Probability_l1"() -> (w2274:u16)
              n1388 = local read "LC_Reward_Block_l1"() -> (w2280:u16)
              n1389 = local read "LC_Reward_Tdelay_l1"() -> (w2272:u16)
              n1390 = local read "LC_Reward_OnOff_l1"() -> (w2278:bool)
              n1391 = local read "LC_Reward_Trial_l1"() -> (w2270:u16)
              n1392 = Boolean To (0,1)(Boolean=w2263) -> (0, 1=w2264:i16)
              n1393 = Boolean To (0,1)(Boolean=w2278) -> (0, 1=w2277:i16)
              n1394 = To Unsigned Word Integer(number=w2264) -> (unsigned 16bit integer=w2261:u16)
              n1395 = To Unsigned Word Integer(number=w2277) -> (unsigned 16bit integer=w2276:u16)
              n1396 = Replace Array Subset(array=w2282, new element #1=w2280, index #1=w2281, new element #2=w2276, index #2=w2279, new element #3=w2274, index #3=w2275, new element #4=w2272, index #4=w2273, new element #5=w2270, index #5=w2271, new element #6=w2262, index #6=w2269, new element #7=w2261, index #7=w2268, new element #8=w2260, index #8=w2267, new element #9=w2259, index #9=w2266, new element #10=w2258, index #10=w2265) -> (w2283:u16[])
            }
            frame "SaveSettings6_LC_l2_Other" {
              # "Trial"
              # "Tdelay"
              # "Probability"
              # "OnOff"
              # "Block"
              # "Wrong"
              # "Trial"
              # "Tdelay"
              # "Probability"
              # "OnOff"
              # "Block"
              # "Reward"
              n1397 = call "myRIO_BRig_RT_dataLC_Wrong_Block_l2.vi"() -> ("output_Wrong_Block_l2"=w2292:i32)  [unwired: 11 in]
              n1398 = call "myRIO_BRig_RT_dataLC_Wrong_OnOff_l2.vi"() -> ("output_Wrong_OnOff_l2"=w2293:i32)  [unwired: 11 in]
              n1399 = call "myRIO_BRig_RT_dataLC_Wrong_Probability_l2.vi"() -> ("output_Wrong_Probability_l2"=w2294:i32)  [unwired: 11 in]
              n1400 = call "myRIO_BRig_RT_dataLC_Wrong_Tdelay_l2.vi"() -> ("output_Wrong_Tdelay_l2"=w2295:i32)  [unwired: 11 in]
              n1401 = call "myRIO_BRig_RT_dataLC_Wrong_Trial_l2.vi"() -> ("output_Wrong_Trial_l2"=w2296:i32)  [unwired: 11 in]
              n1402 = call "myRIO_BRig_RT_dataLC_Reward_Block_l2.vi"() -> ("output_Reward_Block_l2"=w2297:i32)  [unwired: 11 in]
              n1403 = call "myRIO_BRig_RT_dataLC_Reward_OnOff_l2.vi"() -> ("output_Reward_OnOff_l2"=w2298:i32)  [unwired: 11 in]
              n1404 = call "myRIO_BRig_RT_dataLC_Reward_Probability_l2.vi"() -> ("output_Reward_Probability_l2"=w2299:i32)  [unwired: 11 in]
              n1405 = call "myRIO_BRig_RT_dataLC_Reward_Tdelay_l2.vi"() -> ("output_Reward_Tdelay_l2"=w2300:i32)  [unwired: 11 in]
              n1406 = call "myRIO_BRig_RT_dataLC_Reward_Trial_l2.vi"() -> ("output_Reward_Trial_l2"=w2301:i32)  [unwired: 11 in]
              n1407 = local read "LC_Wrong_OnOff_l2"() -> (w2313:bool)
              n1408 = local read "LC_Wrong_Probability_l2"() -> (w2310:u16)
              n1409 = local read "LC_Wrong_Block_l2"() -> (w2312:u16)
              n1410 = local read "LC_Wrong_Tdelay_l2"() -> (w2309:u16)
              n1411 = local read "LC_Wrong_Trial_l2"() -> (w2308:u16)
              n1412 = local read "LC_Reward_Probability_l2"() -> (w2317:u16)
              n1413 = local read "LC_Reward_Block_l2"() -> (w2321:u16)
              n1414 = local read "LC_Reward_Tdelay_l2"() -> (w2316:u16)
              n1415 = local read "LC_Reward_OnOff_l2"() -> (w2320:bool)
              n1416 = local read "LC_Reward_Trial_l2"() -> (w2315:u16)
              n1417 = Boolean To (0,1)(Boolean=w2313) -> (0, 1=w2314:i16)
              n1418 = Boolean To (0,1)(Boolean=w2320) -> (0, 1=w2319:i16)
              n1419 = To Unsigned Word Integer(number=w2314) -> (unsigned 16bit integer=w2311:u16)
              n1420 = To Unsigned Word Integer(number=w2319) -> (unsigned 16bit integer=w2318:u16)
              n1421 = Replace Array Subset(array=w2322, new element #1=w2321, index #1=w2297, new element #2=w2318, index #2=w2298, new element #3=w2317, index #3=w2299, new element #4=w2316, index #4=w2300, new element #5=w2315, index #5=w2301, new element #6=w2312, index #6=w2292, new element #7=w2311, index #7=w2293, new element #8=w2310, index #8=w2294, new element #9=w2309, index #9=w2295, new element #10=w2308, index #10=w2296) -> (w2323:u16[])
            }
            frame "setSettings_Audio" {
              # "amp_L"
              # "amp_R"
              # "freq_L"
              # "freq_R"
              n1422 = call "myRIO_BRig_RT_dataExp_Audio_amp__L.vi"() -> ("output_Audio_amp__L"=w2351:i32)  [unwired: 11 in]
              n1423 = call "myRIO_BRig_RT_dataExp_Audio_amp__R.vi"() -> ("output_Audio_amp__R"=w2350:i32)  [unwired: 11 in]
              n1424 = call "myRIO_BRig_RT_dataExp_Audio_freq__L.vi"() -> ("output_Audio_freq__L"=w2349:i32)  [unwired: 11 in]
              n1425 = call "myRIO_BRig_RT_dataExp_Audio_freq__R.vi"() -> ("output_Audio_freq__R"=w2348:i32)  [unwired: 11 in]
              n1426 = Index Array(array=w2347, index #1=w2351, index #2=w2350, index #3=w2349, index #4=w2348) -> (element #1=w2336:u16, element #2=w2335:u16, element #3=w2340:u16, element #4=w2339:u16)
              n1427 = To Unsigned Byte Integer(number=w2340) -> (unsigned 8bit integer=w2334:u8)
              n1428 = To Unsigned Byte Integer(number=w2339) -> (unsigned 8bit integer=w2333:u8)
              n1429 = xnode "Read/Write Control"("FPGA VI Reference In"=w2338, "error in"=w2337, "audioAmp_L"=w2336, "audioAmp_R"=w2335, "audioFreq_L_kHz"=w2334, "audioFreq_R_kHz"=w2333) -> ("error out"=w2332:errorcluster)  [unwired: 1 out]
              n1430 = local write "error out"(w2332) -> ()
            }
            frame "setSettings_Laser" {
              w2382 = u32 0 ("laser2_selRew_Ndelay")
              # "tDelay"
              # "Wrong l1"
              # "Reward l1"
              n1431 = call "myRIO_BRig_RT_dataExp_IallReward.vi"() -> ("output_I_allReward"=w2363:i32)  [unwired: 11 in]
              n1432 = local read "Laser_Tpeak_l1"() -> (w2393:dbl)
              n1433 = local read "Laser_Tshutter_l1"() -> (w2391:dbl)
              n1434 = local read "Laser_Freq_l1"() -> (w2392:dbl)
              n1435 = local read "Laser_duration_l1"() -> (w2367:u16)
              n1436 = local read "Laser_Tpeak_l2"() -> (w2389:dbl)
              n1437 = local read "Laser_Tshutter_l2"() -> (w2387:dbl)
              n1438 = local read "Laser_Freq_l2"() -> (w2388:dbl)
              n1439 = local read "Laser_duration_l2"() -> (w2366:u16)
              n1440 = local read "CueLed_Freq"() -> (w2376:dbl)
              n1441 = local read "CueLed_Tpeak"() -> (w2377:dbl)
              n1442 = local read "I_allReward"() -> (w2362:bool)
              n1443 = call "myRIO_BRig_RT_dataLC_Reward_Tdelay_l1.vi"() -> ("output_Reward_Tdelay_l1"=w2405:i32)  [unwired: 11 in]
              n1444 = call "myRIO_BRig_RT_dataLC_Wrong_Tdelay_l1.vi"() -> ("output_Wrong_Tdelay_l1"=w2406:i32)  [unwired: 11 in]
              n1445 = local read "FPGA_count2ms"() -> (w2378:dbl)
              n1446 = Index Array(array=w2373, index #1=w2405, index #2=w2406) -> (element #1=w2404:u16, element #2=w2403:u16)
              n1447 = To Double Precision Float(number=w2404) -> (double precision float=w2400:dbl)
              n1448 = To Double Precision Float(number=w2403) -> (double precision float=w2397:dbl)
              n1449 = Boolean To (0,1)(Boolean=w2362) -> (0, 1=w2361:i16)
              n1450 = To Unsigned Word Integer(number=w2361) -> (unsigned 16bit integer=w2360:u16)
              n1451 = Replace Array Subset(array=w2365, new element=w2360, index=w2363) -> (w2364:u16[])
              n1452 = To Unsigned Word Integer(number=w2378) -> (unsigned 16bit integer=w2394:u16)
              n1453 = call "myRIO_BRig_RT__calc_laser_FPGA_N.vi"("input_FPGA_ms2count"=w2378, "input_Tpeak"=w2393, "input_Freq"=w2392, "input_Tshutter"=w2391, "input_duration"=w2367) -> ("output_laser_Npeak"=w2381:u32, "output_laser_Nvalley"=w2380:u32, "output_laser_Nshutter"=w2379:u32, "output_laser_Nduration"=w2390:u32, "output_laser_Tduration"=w2371:u16)  [unwired: 6 in]
              n1454 = Multiply(x=w2378, y=w2400) -> (x*y=w2401:dbl)
              n1455 = Multiply(x=w2378, y=w2397) -> (x*y=w2398:dbl)
              n1456 = call "myRIO_BRig_RT__calc_laser_FPGA_N__CueLed.vi"("input_FPGA_ms2count"=w2378, "input_Tpeak"=w2377, "input_Freq"=w2376) -> ("output_laser_Npeak"=w2375:u32, "output_laser_Nvalley"=w2374:u32)  [unwired: 11 in]
              n1457 = call "myRIO_BRig_RT__calc_laser_FPGA_N.vi"("input_FPGA_ms2count"=w2378, "input_Tpeak"=w2389, "input_Freq"=w2388, "input_Tshutter"=w2387, "input_duration"=w2366) -> ("output_laser_Npeak"=w2386:u32, "output_laser_Nvalley"=w2385:u32, "output_laser_Nshutter"=w2384:u32, "output_laser_Nduration"=w2383:u32, "output_laser_Tduration"=w2370:u16)  [unwired: 6 in]
              n1458 = Round Toward +Infinity(x=w2401) -> (ceil(x): smallest int >= x=w2402:dbl)
              n1459 = Round Toward +Infinity(x=w2398) -> (ceil(x): smallest int >= x=w2399:dbl)
              n1460 = To Unsigned Long Integer(number=w2402) -> (unsigned 32bit integer=w2396:u32)
              n1461 = To Unsigned Long Integer(number=w2399) -> (unsigned 32bit integer=w2395:u32)
              n1462 = xnode "Read/Write Control"("FPGA VI Reference In"=w2407, "error in"=w2408, "I_allReward"=w2362, "LC_nPeak_l1"=w2381, "LC_nValley_l1"=w2380, "LC_nShutter_l1"=w2379, "LR_reward_nDelay_l1"=w2396, "LR_wrong_nDelay_l1"=w2395, "LR_reward_nTotal_l1"=w2390, "LR_wrong_nTotal_l1"=w2390, "k1__counter_per_ms"=w2394, "LC_nPeak_l2"=w2386, "LC_nValley_l2"=w2385, "LC_nShutter_l2"=w2384, "LR_reward_nDelay_l2"=w2382, "LR_wrong_nDelay_l2"=w2382, "LR_reward_nTotal_l2"=w2383, "LR_wrong_nTotal_l2"=w2383, "CueLed_nPeak"=w2375, "CueLed_nValley"=w2374) -> ("error out"=→"error out":errorcluster)  [unwired: 1 out]
              n1463 = call "myRIO_BRig_RT_dataCurrent_laser1_pulse_duration.vi"() -> ("output_laser1_pulse_duration"=w2369:i32)  [unwired: 11 in]
              n1464 = call "myRIO_BRig_RT_dataCurrent_laser2_pulse_duration.vi"() -> ("output_laser2_pulse_duration"=w2368:i32)  [unwired: 11 in]
              n1465 = Replace Array Subset(array=w2373, new element #1=w2371, index #1=w2369, new element #2=w2370, index #2=w2368) -> (w2372:u16[])
            }
            frame "initBlock" {
              n1466 = local write "nRewards_cur"(u16 0 ("nRewards_cur")) -> ()
              n1467 = call "myRIO_Brig_RT__Case_Exp_State_initBlock__v2.vi"("input_spout"=w2429, "input_dataCurrent"=w2435, "input_dataExp"=w2432, "input_dataBlock"=w2424) -> ("output_state"=w2428:T2, "output_spout"=w2427:enum16{"Left", "Right"}, "idxDataBlock"=w2430:i32, "output_dataCurrent"=w2434:u16[], "output_dataExp"=w2433:u16[], "output_TpB_target"=→"TpB_target":u16, "output_iBlock"=w2425:u16, "output_dataBlock"=w2423:u16[][])  [unwired: 4 in]
              "iBlock" <- w2425
              "cSpout" <- w2427
            }
            frame "initBlock2" {
              n1468 = call "myRIO_BRig_RT__Case_Exp_State_initBlock2.vi"("input_spout"=w2452, "input_dataBlock"=w2453, "input_dataCurrent"=w2451) -> ("idxDataBlock"=w2448:i32, "output_dataBlock"=w2450:u16[][])  [unwired: 7 in]
            }
            frame "initTrial" {
              n1469 = xnode "Read/Write Control"("FPGA VI Reference In"=w2468, "error in"=w2467, "SelectionState"=FALSE) -> ("error out"=w2466:errorcluster)  [unwired: 1 out]
              n1470 = call "myRIO_Brig_RT__Case_Exp_State_initTrial__v2.vi"("input_spout"=w2469, "input_dataBlock"=w2464, "input_dataExp"=w2480, "input_dataCurrent"=w2481) -> ("output_state"=w2482:T2, "output_dataExp"=w2479:u16[], "output_dataCurrent"=w2474:u16[], "output_iTrial"=w2463:u16, "output_SolenoidReward"=→"SolenoidReward":bool)  [unwired: 3 in]
              "iTrial" <- w2463
              n1471 = local write "error out"(w2466) -> ()
            }
            frame "initTrial2" {
              # "trialUntilReward"
              n1472 = call "myRIO_BRig_RT__Case_Exp_subState_LC__initTrial__v4.vi"("input_dataCurrent"=w2488, "input_dataExp"=w2486, "input_dataLC"=w2498, "input_spout"=w2499, "input_dataTrial"=w2501) -> ("output_dataTrial"=w2500:u16[][], "output_LR_Wrong_Laser_l2"=w2490:bool, "output_dataCurrent"=w2487:u16[], "output_LR_Reward_Laser_l2"=w2491:bool, "output_LR_Reward_Event_l1"=w2497:bool, "output_LR_Wrong_Event_l1"=w2496:bool, "output_LR_Reward_Laser_l1"=w2495:bool, "output_LR_Wrong_Laser_l1"=w2494:bool, "output_LR_Reward_Event_l2"=w2493:bool, "output_LR_Wrong_Event_l2"=w2492:bool)  [unwired: 5 in]
              n1473 = call "myRIO_BRig_RT_dataExp_ItrialUntilReward.vi"() -> ("output_I_trialUntilReward"=w2505:i32)  [unwired: 11 in]
              n1474 = Index Array(array=w2486, index=w2505) -> (element=w2504:u16)
              n1475 = Equal?(x=w2499, y=enum16{"Left", "Right"}."Right") -> (x = y?=w2503:bool)
              n1476 = Not Equal To 0?(x=w2504) -> (x != 0?=w2502:bool)
              n1477 = xnode "Read/Write Control"("FPGA VI Reference In"=w2515, "error in"=w2514, "Left(F)_or_Right(T)"=w2503, "ignoreWrong"=w2502, "LR_reward_Event_l1"=w2497, "LR_wrong_Event_l1"=w2496, "LR_reward_Laser_l1"=w2495, "LR_wrong_Laser_l1"=w2494, "LR_reward_Event_l2"=w2493, "LR_wrong_Event_l2"=w2492, "LR_reward_Laser_l2"=w2491, "LR_wrong_laser_l2"=w2490) -> ("error out"=w2489:errorcluster)  [unwired: 1 out]
              n1478 = local write "error out"(w2489) -> ()
            }
            frame "initTrial3" {
              # "Cue1_CueType"
              n1479 = call "myRIO_BRig_RT_dataExp_CueLed.vi"() -> ("output_CueLed"=w2524:i32)  [unwired: 11 in]
              n1480 = call "myRIO_BRig_RT_arrTrig_init.vi"() -> ("output_arrTrig"=w2528:bool[])  [unwired: 11 in]
              n1481 = Index Array(array=w2525, index=w2524) -> (element=w2523:u16)
              n1482 = call "myRIO_BRig_RT_arrTrig_Cue1_CueType_AudioLed.vi"() -> ("output_arrTrig_Cue1_CueType_AudioLed"=w2526:i32)  [unwired: 11 in]
              n1483 = Not Equal To 0?(x=w2523) -> (x != 0?=w2522:bool)
              n1484 = call "myRIO_BRig_RT__Case_Exp_State_initTrial_dataTrial.vi"("input_spout"=w2541, "input_dataCurrent"=w2530, "input_dataExp"=w2525, "input_dataTrial"=w2543) -> ("output_laserPower_l2"=w2531:u16, "output_dataCurrent"=w2529:u16[], "output_dataTrial"=w2542:u16[][], "output_laserPower_l1"=w2538:u16)  [unwired: 4 in]
              n1485 = To Double Precision Float(number=w2538) -> (double precision float=w2540:dbl)
              n1486 = To Double Precision Float(number=w2531) -> (double precision float=w2534:dbl)
              n1487 = Replace Array Subset(array=w2528, new element=w2522, index=w2526) -> (w2527:bool[])
              n1488 = Divide(x=w2540, y=100.0 ("x")) -> (x/y=w2535:dbl)
              "power_l1" <- w2535
              n1489 = Divide(x=w2534, y=100.0 ("x")) -> (x/y=w2532:dbl)
              "power_l2" <- w2532
              n1490 = call "myRIO__convert__Voltage_to_FPGAvalue.vi"("input_voltage"=w2535) -> ("output_PortA"=w2520:u16)  [unwired: 9 in, 1 out]
              n1491 = call "myRIO__convert__Voltage_to_FPGAvalue.vi"("input_voltage"=w2532) -> ("output_PortA"=w2519:u16)  [unwired: 9 in, 1 out]
              n1492 = xnode "Read/Write Control"("FPGA VI Reference In"=w2537, "error in"=w2536, "AnaOut_0"=w2520, "AnaOut_1"=w2519) -> ("error out"=w2521:errorcluster)  [unwired: 1 out]
              n1493 = local write "error out"(w2521) -> ()
            }
            frame "initTrial4" {
              n1494 = call "myRIO_BRig_RT_dataTrial_activeRecording.vi"() -> ("output_activeRecording"=w2563:i32)  [unwired: 11 in]
              n1495 = call "myRIO_BRig_RT_dataCurrent_idxDataTrial.vi"() -> ("output_idxDataTrial"=w2566:i32)  [unwired: 11 in]
              n1496 = Index Array(array=w2568, index=w2566) -> (element=w2565:u16)
              n1497 = xnode "Read/Write Control"("FPGA VI Reference In"=w2558, "error in"=w2557, "A6_Act"="Recording") -> ("error out"=w2555:errorcluster)  [unwired: 1 out]
              n1498 = Boolean To (0,1)(Boolean="Recording") -> (0, 1=w2562:i16)
              n1499 = To Long Integer(number=w2565) -> (32bit integer=w2564:i32)
              n1500 = To Unsigned Word Integer(number=w2562) -> (unsigned 16bit integer=w2561:u16)
              n1501 = local write "error out"(w2555) -> ()
              n1502 = Replace Array Subset(array=w2567, new element=w2561, index (row)=w2564, index (col)=w2563) -> (w2560:u16[][])
            }
            frame "initTrial_LC_ENL1" {
              n1503 = call "myRIO_BRig_RT__Case_Exp_State_initTrial_LC_ENL1__v4.vi"("input_dataTrial"=w2587, "input_spout"=w2590, "input_arrTrig"=w2584, "input_dataBlock"=w2585, "input_dataLC"=w2591, "input_dataCurrent"=w2589) -> ("output_arrTrig"=w2583:bool[], "output_dataTrial"=w2586:u16[][], "output_dataCurrent"=w2588:u16[])  [unwired: 3 in]
            }
            frame "initTrial_LC_Cue1" {
              n1504 = call "myRIO_BRig_RT__Case_Exp_State_initTrial_LC_Cue1__v4.vi"("input_dataTrial"=w2606, "input_spout"=w2609, "input_arrTrig"=w2603, "input_dataBlock"=w2604, "input_dataLC"=w2610, "input_dataCurrent"=w2608) -> ("output_arrTrig"=w2602:bool[], "output_dataTrial"=w2605:u16[][], "output_dataCurrent"=w2607:u16[])  [unwired: 3 in]
            }
            frame "initTrial_LC_Sel" {
              n1505 = xnode "Read/Write Control"("FPGA VI Reference In"=w2623, "error in"=w2622, "A6_Act"=FALSE) -> ("error out"=w2624:errorcluster)  [unwired: 1 out]
              n1506 = local write "error out"(w2624) -> ()
              n1507 = call "myRIO_BRig_RT__Case_Exp_State_initTrial_LC_Sel__v4.vi"("input_dataTrial"=w2629, "input_spout"=w2632, "input_arrTrig"=w2626, "input_dataBlock"=w2627, "input_dataLC"=w2633, "input_dataCurrent"=w2631) -> ("output_arrTrig"=w2625:bool[], "output_dataTrial"=w2628:u16[][], "output_dataCurrent"=w2630:u16[])  [unwired: 3 in]
            }
            frame "ENL1_pre" {
              n1508 = call "myRIO_BRig_RT__Case_Exp_State_Enl1Pre__v3.vi"("input_I_lick"=w2647, "input_arrTrig"=w2644, "input_dataCurrent"=w2648) -> ("output_dataCurrent"=w2645:u16[], "output_state"=w2646:T2)  [unwired: 3 in, 4 out]
            }
            frame "ENL1" {
              n1509 = call "myRIO_BRig_RT__Case_Exp_State_ENL1__v3.vi"("I_lick"=w2667, "input_arrTrig"=w2665, "input_state"=w2671, "input_dataCurrent"=w2670) -> ("output_l1_laserOn"=w2663:bool, "output_l1_laserEvent"=w2664:bool, "output_state"=w2668:T2, "output_dataCurrent"=w2669:u16[], "output_l2_laserEvent"=w2662:bool, "output_l2_laserOn"=w2661:bool)  [unwired: 2 in]
            }
            frame "ENL1Penalty_pre" {
              # "Tcycle"
              # "counter"
              n1510 = call "myRIO_BRig_RT_dataCurrent_Tcycle_generic.vi"() -> ("output_Tcycle_generic"=w2698:i32)  [unwired: 11 in]
              n1511 = call "myRIO_BRig_RT_dataCurrent_count_generic.vi"() -> ("output_count_generic"=w2700:i32)  [unwired: 11 in]
              n1512 = call "myRIO_BRig_RT_dataExp_ENL_penalty.vi"() -> ("output_ENL_penalty"=w2693:i32)  [unwired: 11 in]
              n1513 = Index Array(array=w2694, index=w2693) -> (element=w2697:u16)
              n1514 = Replace Array Subset(array=w2695, new element #1=u16 0 ("new element/subarray"), index #1=w2700, new element #2=w2697, index #2=w2698) -> (w2696:u16[])
            }
            frame "ENL1Penalty" {
              n1515 = call "myRIO_BRig_RT__Case_Exp_State_ENL1Penalty.vi"("input_state"=w2714, "input_dataCurrent"=w2718) -> ("output_state"=w2715:T2, "output_dataCurrent"=w2717:u16[])  [unwired: 8 in]
            }
            frame "ENL2_pre" {
            }
            frame "ENL2" {
            }
            frame "ENL2Penalty_pre" {
            }
            frame "ENL2Penalty" {
            }
            frame "Cue1_pre" {
              n1516 = call "myRIO_BRig_RT__Case_Exp_State_Cue1Pre__v3.vi"("input_dataCurrent"=w2790, "input_dataExp"=w2786, "input_arrTrig"=w2783, "input_spout"=w2787) -> ("output_audioR"=w2784:bool, "output_audioL"=w2785:bool, "output_state"=w2788:T2, "output_dataCurrent"=w2789:u16[])  [unwired: 7 in, 5 out]
            }
            frame "Cue1" {
              n1517 = call "myRIO_BRig_RT__Case_Exp_State_Cue1__v4.vi"("input_state"=w2811, "input_dataCurrent"=w2812, "I_lick"=w2810, "input_arrTrig"=w2813) -> ("output_SelectionState"=w2804:bool, "output_CueLed_Event"=w2809:bool, "output_state"=w2805:T2, "output_dataCurrent"=w2806:u16[], "output_l1_laserEvent"=w2802:bool, "output_l1_laserOn"=w2803:bool, "output_l2_laserEvent"=w2807:bool, "output_l2_laserOn"=w2808:bool)  [unwired: 8 in]
              n1518 = xnode "Read/Write Control"("FPGA VI Reference In"=w2816, "error in"=w2815, "SelectionState"=w2804) -> ()  [unwired: 2 out]
            }
            frame "Cue1Penalty_pre" {
              # "Tcycle"
              # "counter"
              n1519 = call "myRIO_BRig_RT_dataCurrent_Tcycle_generic.vi"() -> ("output_Tcycle_generic"=w2852:i32)  [unwired: 11 in]
              n1520 = call "myRIO_BRig_RT_dataCurrent_count_generic.vi"() -> ("output_count_generic"=w2854:i32)  [unwired: 11 in]
              n1521 = call "myRIO_BRig_RT_dataExp_CueLed.vi"() -> ("output_CueLed"=w2836:i32)  [unwired: 11 in]
              n1522 = call "myRIO_BRig_RT_dataExp_Tcycle_Cue1Penalty_Audio.vi"() -> ("output_Tcycle_Cue1Penalty_Audio"=w2837:i32)  [unwired: 11 in]
              n1523 = call "myRIO_BRig_RT_dataExp_Tcycle_Cue1Penalty_LED.vi"() -> ("output_Tcycle_Cue1Penalty_LED"=w2835:i32)  [unwired: 11 in]
              n1524 = Index Array(array=w2848, index #1=w2836, index #2=w2837, index #3=w2835) -> (element #1=w2834:u16, element #2=w2832:u16, element #3=w2831:u16)
              n1525 = Equal To 0?(x=w2834) -> (x = 0?=w2833:bool)
              n1526 = Select(t=w2832, s=w2833, f=w2831) -> (s? t:f=w2830:u16)
              n1527 = Replace Array Subset(array=w2850, new element #1=u16 0 ("new element/subarray"), index #1=w2854, new element #2=w2830, index #2=w2852) -> (w2849:u16[])
            }
            frame "Cue1Penalty" {
              n1528 = call "myRIO_BRig_RT__Case_Exp_State_Cue1Penalty.vi"("input_state"=w2871, "input_dataCurrent"=w2872) -> ("output_state"=w2869:T2, "output_dataCurrent"=w2870:u16[])  [unwired: 8 in]
            }
            frame "Cue2_pre" {
            }
            frame "Cue2" {
            }
            frame "Cue2Penalty_pre" {
            }
            frame "Cue2Penalty" {
            }
            frame "Selection_pre" {
              n1529 = xnode "Read/Write Control"("FPGA VI Reference In"=w2950, "error in"=w2951) -> ("error out"=w2938:errorcluster, "SelectReward"=w2945:bool, "SelectWrong"=w2946:bool)  [unwired: 1 out]
              n1530 = local write "error out"(w2938) -> ()
              n1531 = call "myRIO_BRig_RT__Case_Exp_State_SelectPre__v4.vi"("input_dataCurrent"=w2949, "input_SelectWrong"=w2946, "input_SelectReward"=w2945, "input_dataExp"=w2939, "input_LickL"=w2937, "input_LickR"=w2936, "input_arrTrig"=w2944) -> ("output_state"=w2947:T2, "output_dataCurrent"=w2948:u16[], "output_l1_laserEvent"=w2943:bool, "output_l1_laserOn"=w2942:bool, "output_l2_laserOn"=w2940:bool, "output_l2_laserEvent"=w2941:bool)  [unwired: 3 in]
            }
            frame "Selection" {
              n1532 = xnode "Read/Write Control"("FPGA VI Reference In"=w2978, "error in"=w2977) -> ("error out"=w2965:errorcluster, "SelectReward"=w2972:bool, "SelectWrong"=w2971:bool)  [unwired: 1 out]
              n1533 = local write "error out"(w2965) -> ()
              n1534 = call "myRIO_BRig_RT__Case_Exp_State_Selection__v4.vi"("input_dataCurrent"=w2976, "input_state"=w2974, "input_dataExp"=w2964, "input_LickL"=w2963, "input_FPGA_SelectReward"=w2972, "input_FPGA_SelectWrong"=w2971, "input_LickR"=w2962, "input_arrTrig"=w2970) -> ("output_state"=w2973:T2, "output_dataCurrent"=w2975:u16[], "output_LC_Event_l1"=w2969:bool, "output_LC_Laser_l2"=w2966:bool, "output_LC_Event_l2"=w2967:bool, "output_LC_Laser_l1"=w2968:bool)  [unwired: 2 in]
            }
            frame "SelectReward_pre" {
              # "iState"
              # "nRewTrials"
              # "Tcycle\nGeneric"
              # "counter"
              n1535 = call "myRIO_BRig_RT_dataCurrent_nRewTrials.vi"() -> ("output_nRewTrials"=w3002:i32)  [unwired: 11 in]
              n1536 = call "myRIO_BRig_RT_dataCurrent_Tcycle_reward.vi"() -> ("output_Tcycle_reward"=w2991:i32)  [unwired: 11 in]
              n1537 = Index Array(array=w2989, index #1=w3002, index #2=w2991) -> (element #1=w3001:u16, element #2=w2990:u16)
              n1538 = Increment(x=w3001) -> (x+1=w3000:u16)
              n1539 = call "myRIO_BRig_RT__Case_Exp_subState_LC__Reward.vi"("input_spout"=w3009, "input_dataCurrent"=w2989, "input_dataLC"=w3008) -> ()  [unwired: 6 in, 2 out]
              n1540 = call "myRIO_BRig_RT_dataCurrent_count_generic.vi"() -> ("output_count_generic"=w3004:i32)  [unwired: 11 in]
              n1541 = call "myRIO_BRig_RT_dataCurrent_Tcycle_generic.vi"() -> ("output_Tcycle_generic"=w3005:i32)  [unwired: 11 in]
              n1542 = call "myRIO_BRig_RT_dataCurrent_iState.vi"() -> ("output_iState"=w2999:i32)  [unwired: 11 in]
              n1543 = Replace Array Subset(array=w2989, new element #1=w3000, index #1=w3002, new element #2=u16 0 ("new element/subarray"), index #2=w3004, new element #3=w2990, index #3=w3005, new element #4=u16 1 ("new element/subarray"), index #4=w2999) -> (w3011:u16[])
            }
            frame "SelectReward" {
              n1544 = call "myRIO_BRig_RT__Case_Exp_State_Reward.vi"("input_dataCurrent"=w3028, "input_state"=w3025, "input_spout"=w3023) -> ("output_dataCurrent"=w3027:u16[], "output_state"=w3026:T2, "output__L"=w3021:bool, "output__R"=w3022:bool)  [unwired: 9 in]
            }
            frame "SelectRewardPost_pre" {
              # "nRewards"
              # "nRewTrials"
              # "Tcycle"
              # "counter"
              n1545 = call "myRIO_BRig_RT_dataBlock_nRewards__L.vi"() -> ("output_nRewards__L"=w3044:i32)  [unwired: 11 in]
              n1546 = call "myRIO_BRig_RT_dataBlock_nRewards__R.vi"() -> ("output_nRewards__R"=w3043:i32)  [unwired: 11 in]
              n1547 = call "myRIO_BRig_RT_dataCurrent_Tcycle_generic.vi"() -> ("output_Tcycle_generic"=w3059:i32)  [unwired: 11 in]
              n1548 = call "myRIO_BRig_RT_dataCurrent_count_generic.vi"() -> ("output_count_generic"=w3061:i32)  [unwired: 11 in]
              n1549 = case shown="\"Left\", Default" w3037 {
                tunnel: w3049 -> [w3066 w3070]
                tunnel: [w3065 w3070] -> w3048
                tunnel: [w3067 w3068] -> w3047
                tunnel: w3046 -> [w3067 w3069]
                frame "Left", Default {
                  n1550 = Increment(x=w3066) -> (x+1=w3065:u16)
                }
                frame "Right" {
                  n1551 = Increment(x=w3069) -> (x+1=w3068:u16)
                }
              }
              "nRewards_Left" <- w3048
              "nRewards_Right" <- w3047
              n1552 = Equal?(x=w3037, y=enum16{"Left", "Right"}."Left") -> (x = y?=w3036:bool)
              n1553 = Select(t=w3044, s=w3036, f=w3043) -> (s? t:f=w3042:i32)
              n1554 = call "myRIO_BRig_RT_dataExp_Tcycle_RewardPost.vi"() -> ("output_Tcycle_RewardPost"=w3055:i32)  [unwired: 11 in]
              n1555 = call "myRIO_BRig_RT_dataCurrent_nRewTrials.vi"() -> ("output_nRewTrials"=w3045:i32)  [unwired: 11 in]
              n1556 = Index Array(array=w3056, index=w3055) -> (element=w3058:u16)
              n1557 = Index Array(array=w3039, index=w3045) -> (element=w3034:u16)
              n1558 = Replace Array Subset(array=w3039, new element #1=u16 0 ("new element/subarray"), index #1=w3061, new element #2=w3058, index #2=w3059) -> (w3057:u16[])
              n1559 = Replace Array Subset(array=w3041, new element=w3034, index (row)=w3035, index (col)=w3042) -> (w3040:u16[][])
              n1560 = local write "nRewards_cur"(w3034) -> ()
            }
            frame "SelectRewardPost" {
              n1561 = call "myRIO_BRig_RT__Case_Exp_State_RewardPost.vi"("input_state"=w3081, "input_dataCurrent"=w3084) -> ("output_state"=w3082:T2, "output_dataCurrent"=w3083:u16[])  [unwired: 8 in]
            }
            frame "SelectWrong_pre" {
              # "iState"
              # "Tcycle"
              # "counter"
              n1562 = call "myRIO_BRig_RT_dataCurrent_Tcycle_generic.vi"() -> ("output_Tcycle_generic"=w3105:i32)  [unwired: 11 in]
              n1563 = call "myRIO_BRig_RT_dataCurrent_count_generic.vi"() -> ("output_count_generic"=w3107:i32)  [unwired: 11 in]
              n1564 = call "myRIO_BRig_RT_dataExp_Tcycle_Wrong.vi"() -> ("output_Tcycle_Wrong"=w3103:i32)  [unwired: 11 in]
              n1565 = call "myRIO_BRig_RT__Case_Exp_subState_LC__Wrong.vi"("input_spout"=w3099, "input_dataCurrent"=w3100, "input_dataLC"=w3097) -> ()  [unwired: 6 in, 2 out]
              n1566 = Index Array(array=w3101, index=w3103) -> (element=w3104:u16)
              n1567 = call "myRIO_BRig_RT_dataCurrent_iState.vi"() -> ("output_iState"=w3095:i32)  [unwired: 11 in]
              n1568 = Replace Array Subset(array=w3100, new element #1=u16 0 ("new element/subarray"), index #1=w3107, new element #2=w3104, index #2=w3105, new element #3=u16 2 ("new element/subarray"), index #3=w3095) -> (w3102:u16[])
            }
            frame "SelectWrong" {
              n1569 = call "myRIO_BRig_RT__Case_Exp_State_Wrong.vi"("input_state"=w3121, "input_dataCurrent"=w3126) -> ("output_state"=w3118:T2, "output_dataCurrent"=w3125:u16[])  [unwired: 8 in]
              n1570 = Not Equal?(x=w3121, y=w3118) -> (x != y?=w3120:bool)
              n1571 = Select(t=myRIO_BRig_RT__Case_Exp_stateList."SelectWrong_post" ("Enum"), s=w3120, f=w3118) -> (s? t:f=w3117:T2)
            }
            frame "SelectWrong_post" {
            }
            frame "SelectTimeout_pre" {
              # "iState"
              # "Tcycle"
              # "counter"
              n1572 = xnode "Read/Write Control"("FPGA VI Reference In"=w3149, "error in"=w3148, "SelectionState"=FALSE) -> ("error out"=w3146:errorcluster)  [unwired: 1 out]
              n1573 = call "myRIO_BRig_RT_dataCurrent_Tcycle_generic.vi"() -> ("output_Tcycle_generic"=w3167:i32)  [unwired: 11 in]
              n1574 = call "myRIO_BRig_RT_dataCurrent_count_generic.vi"() -> ("output_count_generic"=w3165:i32)  [unwired: 11 in]
              n1575 = call "myRIO_BRig_RT_dataExp_Tcycle_Timeout.vi"() -> ("output_Tcycle_Timeout"=w3169:i32)  [unwired: 11 in]
              n1576 = local write "error out"(w3146) -> ()
              n1577 = call "myRIO_BRig_RT__Case_Exp_subState_LC__Timeout.vi"("input_spout"=w3160, "input_dataCurrent"=w3161, "input_dataLC"=w3159) -> ()  [unwired: 6 in, 2 out]
              n1578 = Index Array(array=w3163, index=w3169) -> (element=w3168:u16)
              n1579 = call "myRIO_BRig_RT_dataCurrent_iState.vi"() -> ("output_iState"=w3157:i32)  [unwired: 11 in]
              n1580 = Replace Array Subset(array=w3161, new element #1=u16 0 ("new element/subarray"), index #1=w3165, new element #2=w3168, index #2=w3167, new element #3=u16 3 ("new element/subarray"), index #3=w3157) -> (w3164:u16[])
            }
            frame "SelectTimeout" {
              n1581 = call "myRIO_BRig_RT__Case_Exp_State_Timeout.vi"("input_dataLC"=w3184, "input_state"=w3179, "input_dataCurrent"=w3189) -> ("output_state"=w3180:T2, "output_dataCurrent"=w3188:u16[])  [unwired: 6 in, 1 out]
              n1582 = Not Equal?(x=w3179, y=w3180) -> (x != y?=w3183:bool)
              n1583 = Select(t=myRIO_BRig_RT__Case_Exp_stateList."SelectTimeout_post" ("Enum"), s=w3183, f=w3180) -> (s? t:f=w3181:T2)
            }
            frame "SelectTimeout_post" {
            }
            frame "endTrial1" {
              # "Update dataBlock"
              n1584 = call "myRIO_BRig_RT__Case_Exp_State_endTrial1.vi"("input_spout"=w3218, "input_dataBlock"=w3217, "input_dataCurrent"=w3215) -> ("output_dataBlock"=w3216:u16[][], "output_dataCurrent"=w3214:u16[])  [unwired: 7 in]
            }
            frame "endTrial2" {
              # "update dataTrial"
              n1585 = call "myRIO_BRig_RT__Case_Exp_State_endTrial2.vi"("input_dataExp"=w3225, "input_spout"=w3234, "input_dataTrial"=w3238, "input_dataCurrent"=w3236) -> ("output_dataTrial"=w3237:u16[][], "output_dataCurrent"=w3235:u16[])  [unwired: 6 in]
            }
            frame "endTrial3" {
              # "nRewTrials"
              # "iTrial"
              # "I_blockUntilReward"
              # "TPB"
              # "end block?"
              n1586 = local read "STOP_endTrial"() -> (w3259:bool)
              n1587 = local read "STOP_abort"() -> (w3258:bool)
              n1588 = xnode "Read/Write Control"("FPGA VI Reference In"=w3249, "error in"=w3248, "SelectionState"=FALSE) -> ("error out"=w3242:errorcluster)  [unwired: 1 out]
              n1589 = local read "START"() -> (w3256:bool)
              n1590 = call "myRIO_BRig_RT_dataExp_IblockUntilReward.vi"() -> ("output_I_blockUntilReward"=w3266:i32)  [unwired: 11 in]
              n1591 = Index Array(array=w3252, index=w3266) -> (element=w3250:u16)
              n1592 = Not(x=w3256) -> (.not. x?=w3257:bool)
              n1593 = local write "error out"(w3242) -> ()
              n1594 = Not Equal To 0?(x=w3250) -> (x != 0?=w3264:bool)
              n1595 = Compound Arithmetic op=OR(w3259, w3257, w3258) -> (w3245:bool)
              n1596 = call "myRIO_BRig_RT_dataCurrent_nRewTrials.vi"() -> ("output_nRewTrials"=w3262:i32)  [unwired: 11 in]
              n1597 = call "myRIO_BRig_RT_dataCurrent_iTrial.vi"() -> ("output_iTrial"=w3263:i32)  [unwired: 11 in]
              n1598 = Select(t=w3262, s=w3264, f=w3263) -> (s? t:f=w3261:i32)
              n1599 = call "myRIO_BRig_RT_dataCurrent_TpB.vi"() -> ("output_TpB"=w3265:i32)  [unwired: 11 in]
              n1600 = Index Array(array=w3253, index #1=w3265, index #2=w3261) -> (element #1=w3254:u16, element #2=w3255:u16)
              n1601 = Less Or Equal?(x=w3254, y=w3255) -> (x <= y?=w3246:bool)
              n1602 = Or(x=w3245, y=w3246) -> (x .or. y?=w3243:bool)
              n1603 = Select(t=myRIO_BRig_RT__Case_Exp_stateList."saveData_dataBlock" ("Enum"), s=w3243, f=myRIO_BRig_RT__Case_Exp_stateList."dummyState" ("Enum")) -> (s? t:f=w3251:T2)
            }
            frame "endBlock" {
              # "R"
              # "L"
              # "idxDataBlock"
              n1604 = Equal?(x=w3286, y=enum16{"Left", "Right"}."Left") -> (x = y?=w3285:bool)
              n1605 = call "myRIO_BRig_RT_dataCurrent_idxDataBlockL.vi"() -> ("output_idxDataBlock__L"=w3289:i32)  [unwired: 11 in]
              n1606 = call "myRIO_BRig_RT_dataCurrent_idxDataBlockR.vi"() -> ("output_idxDataBlock__R"=w3288:i32)  [unwired: 11 in]
              n1607 = Increment(x=w3280) -> (x+1=w3279:i32)
              n1608 = local read "START"() -> (w3305:bool)
              n1609 = local read "STOP_endBlock"() -> (w3300:bool)
              n1610 = local read "STOP_endTrial"() -> (w3303:bool)
              n1611 = local read "STOP_abort"() -> (w3302:bool)
              n1612 = Select(t=w3289, s=w3285, f=w3288) -> (s? t:f=w3283:i32)
              n1613 = To Unsigned Word Integer(number=w3279) -> (unsigned 16bit integer=w3281:u16)
              n1614 = Not(x=w3305) -> (.not. x?=w3304:bool)
              n1615 = Replace Array Subset(array=w3284, new element=w3281, index=w3283) -> (w3282:u16[])
              n1616 = Compound Arithmetic op=OR(w3304, w3300, w3303, w3302) -> (w3301:bool)
              n1617 = Select(t=myRIO_BRig_RT__Case_Exp_stateList."endExp" ("Enum"), s=w3301, f=myRIO_BRig_RT__Case_Exp_stateList."dummyState_endBlock" ("Enum")) -> (s? t:f=w3309:T2)
            }
            frame "endExp" {
              n1618 = xnode "Read/Write Control"("FPGA VI Reference In"=w3312, "error in"=w3311, "A6_Act"=FALSE) -> ("error out"=w3313:errorcluster)  [unwired: 1 out]
              n1619 = local write "error out"(w3313) -> ()
            }
            frame "commConnect" {
              n1620 = call "myRIO_BRig_RT_comm_webdav_connect.vi"("input_password"="Host Password", "input_username"="Host UserName") -> ("output_Iconnected"=w3330:bool, "output_hSession"=w3344:T6)  [unwired: 7 in, 1 out]
              "Connected To Host?" <- w3330
              n1621 = case shown="False" w3330 {
                frame False {
                  n1622 = One Button Dialog(message="Connection Failed!\nData not being saved!") -> ()  [unwired: 1 in, 1 out]
                }
                frame True {
                }
              }
            }
            frame "commUpload_pre" {
              n1623 = Select(t=myRIO_BRig_RT__Case_Exp_stateList."commUpload_dataBlock" ("Enum"), s=w3351, f=myRIO_BRig_RT__Case_Exp_stateList."endBlock") -> (s? t:f=w3349:T2)
            }
            frame "commUpload_dataBlock" {
              n1624 = call "myRIO_BRig_RT_comm_webdav_uploadFile__data.vi"("input_fileName_prefix"=w3368, "input_fileName"="dataBlock" ("input_filename"), "input_hSession"=w3370) -> ()  [unwired: 8 in, 1 out]
            }
            frame "commUpload_dataCurrent" {
              n1625 = call "myRIO_BRig_RT_comm_webdav_uploadFile__data.vi"("input_fileName_prefix"=w3385, "input_fileName"="dataCurrent" ("input_filename"), "input_hSession"=w3387) -> ()  [unwired: 8 in, 1 out]
            }
            frame "commUpload_dataExp" {
              n1626 = call "myRIO_BRig_RT_comm_webdav_uploadFile__data.vi"("input_fileName_prefix"=w3402, "input_fileName"="dataExp" ("input_filename"), "input_hSession"=w3404) -> ()  [unwired: 8 in, 1 out]
            }
            frame "commUpload_dataLC" {
              n1627 = call "myRIO_BRig_RT_comm_webdav_uploadFile__data.vi"("input_fileName_prefix"=w3419, "input_fileName"="dataLC" ("input_filename"), "input_hSession"=w3421) -> ()  [unwired: 8 in, 1 out]
            }
            frame "commUpload_dataTrial" {
              n1628 = call "myRIO_BRig_RT_comm_webdav_uploadFile__data.vi"("input_fileName_prefix"=w3439, "input_fileName"="dataTrial" ("input_filename"), "input_hSession"=w3441) -> ()  [unwired: 8 in, 1 out]
            }
            frame "saveData_dataBlock" {
              # "idxDataBlockR"
              # "idxDataBlockL"
              n1629 = call "myRIO_BRig_RT_dataCurrent_idxDataBlockL.vi"() -> ("output_idxDataBlock__L"=w3461:i32)  [unwired: 11 in]
              n1630 = call "myRIO_BRig_RT_dataCurrent_idxDataBlockR.vi"() -> ("output_idxDataBlock__R"=w3462:i32)  [unwired: 11 in]
              n1631 = Index Array(array=w3463, index #1=w3461, index #2=w3462) -> (element #1=w3460:u16, element #2=w3459:u16)
              n1632 = Greater?(x=w3460, y=w3459) -> (0:w3458:bool)
              n1633 = Select(t=w3460, s=w3458, f=w3459) -> (s? t:f=w3456:u16)
              n1634 = Increment(x=w3456) -> (x+1=w3455:u16)
              n1635 = To Long Integer(number=w3455) -> (32bit integer=w3454:i32)
              n1636 = Array Subset(array=w3457, length (row)=w3454) -> (w3453:u16[][])  [unwired: 3 in]
              n1637 = call "myRIO_BRig_RT_comm_webdav_saveArrayToFile__2D_u16.vi"("Array"=w3453, "input_filename"="dataBlock") -> ()  [unwired: 10 in]
            }
            frame "saveData_dataCurrent" {
              n1638 = call "myRIO_BRig_RT_comm_webdav_saveArrayToFile__1D_u16.vi"("Array"=w3478, "input_filename"="dataCurrent") -> ()  [unwired: 10 in]
            }
            frame "saveData_dataExp" {
              # "runTime"
              n1639 = Get Date/Time In Seconds() -> (seconds since 1Jan1904=w3502:timestamp)
              n1640 = To Double Precision Float(number=w3502) -> (double precision float=w3501:dbl)
              n1641 = call "myRIO_BRig_RT_dataExp_runTime_seconds.vi"() -> ("output_RunTime_minutes"=w3500:i32)  [unwired: 11 in]
              n1642 = Subtract(x=w3501, y=w3499) -> (x-y=w3496:dbl)
              n1643 = To Unsigned Word Integer(number=w3496) -> (unsigned 16bit integer=w3495:u16)
              n1644 = Replace Array Subset(array=w3494, new element=w3495, index=w3500) -> (w3497:u16[])
              n1645 = call "myRIO_BRig_RT_comm_webdav_saveArrayToFile__1D_u16.vi"("Array"=w3497, "input_filename"="dataExp") -> ()  [unwired: 10 in]
            }
            frame "saveData_dataLC" {
              n1646 = call "myRIO_BRig_RT_comm_webdav_saveArrayToFile__1D_u16.vi"("Array"=w3517, "input_filename"="dataLC") -> ()  [unwired: 10 in]
            }
            frame "saveData_dataTrial" {
              # "idxTrial"
              n1647 = call "myRIO_BRig_RT_dataCurrent_idxDataTrial.vi"() -> ("output_idxDataTrial"=w3537:i32)  [unwired: 11 in]
              n1648 = Index Array(array=w3538, index=w3537) -> (element=w3530:u16)
              n1649 = Increment(x=w3530) -> ()  [unwired: 1 out]
              n1650 = To Long Integer(number=w3530) -> (32bit integer=w3534:i32)
              n1651 = Array Subset(array=w3535, length (row)=w3534) -> (w3536:u16[][])  [unwired: 3 in]
              n1652 = call "myRIO_BRig_RT_comm_webdav_saveArrayToFile__2D_u16.vi"("Array"=w3536, "input_filename"="dataTrial") -> ()  [unwired: 10 in]
            }
            frame "dummyState" {
              n1653 = call "myRIO_BRig_RT_dataCurrent_iTrial.vi"() -> ("output_iTrial"=w3556:i32)  [unwired: 11 in]
              n1654 = Index Array(array=w3557, index=w3556) -> (element=w3555:u16)
              n1655 = Equal?(x=w3555, y=u16 1) -> (x = y?=w3553:bool)
              n1656 = Equal To 0?(x=w3564) -> (x = 0?=w3565:bool)
              n1657 = Select(t=u16 13, s=w3553, f=u16 15) -> (s? t:f=w3550:u16)
              n1658 = Select(t=w3550, s=w3565, f=w3564) -> (s? t:f=w3563:u16)
              n1659 = Decrement(x=w3563) -> (x-1=w3562:u16)
              n1660 = Equal To 0?(x=w3562) -> (x = 0?=w3561:bool)
              n1661 = Select(t=myRIO_BRig_RT__Case_Exp_stateList."initTrial" ("Enum"), s=w3561, f=w3559) -> (s? t:f=w3558:T2)
            }
            frame "dummyState_endBlock" {
              n1662 = call "myRIO_BRig_RT_dataCurrent_iTrial.vi"() -> ("output_iTrial"=w3585:i32)  [unwired: 11 in]
              n1663 = Index Array(array=w3586, index=w3585) -> (element=w3584:u16)
              n1664 = Equal?(x=w3584, y=u16 1) -> (x = y?=w3582:bool)
              n1665 = Equal To 0?(x=w3593) -> (x = 0?=w3594:bool)
              n1666 = Select(t=u16 1, s=w3582, f=u16 3) -> (s? t:f=w3579:u16)
              n1667 = Select(t=w3579, s=w3594, f=w3593) -> (s? t:f=w3592:u16)
              n1668 = Decrement(x=w3592) -> (x-1=w3591:u16)
              n1669 = Equal To 0?(x=w3591) -> (x = 0?=w3590:bool)
              n1670 = Select(t=myRIO_BRig_RT__Case_Exp_stateList."initBlock" ("Enum"), s=w3590, f=w3588) -> (s? t:f=w3587:T2)
            }
          }
          n1671 = call "myRIO_BRig_RT_dataMTrig_main.vi"("input_dataMTrig"=w1675, "input_Solenoid_trig_L"=w1672, "input_Solenoid_trig_R"=w1671, "input_Audio_trig_L"=w1670, "input_Audio_trig_R"=w1669, "input_Laser_trig"=w1668) -> ("output_Laser"=w1609:bool, "output_dataMTrig"=w1674:u16[], "output_Solenoid_L"=w1612:bool, "output_Solenoid_R"=w1664:bool, "output_Audio_L"=w1666:bool, "output_Audio_R"=w1667:bool)  [unwired: 8 in]
          n1672 = Compound Arithmetic op=OR(w1672, w1671, w1670, w1669, w1668) -> (w1673:bool)
          n1673 = case shown="True" w1673 {
            frame False {
            }
            frame True {
              w1705 = FALSE
              n1674 = local write "MTrig_Solenoid_trig__L"(w1705) -> ()
              n1675 = local write "MTrig_Solenoid_trig__R"(w1705) -> ()
              n1676 = local write "MTrig_Audio_trig__L"(w1705) -> ()
              n1677 = local write "MTrig_Audio_trig__R"(w1705) -> ()
              n1678 = local write "MTrig_Laser_trig"(w1705) -> ()
            }
          }
          n1679 = local read "MTrig_Laser_Switch"() -> (w1607:bool)
          n1680 = Not(x=w1607) -> (.not. x?=w1608:bool)
          n1681 = And(x=w1609, y=w1608) -> (x .and. y?=w1603:bool)
          n1682 = And(x=w1609, y=w1607) -> (x .and. y?=w1605:bool)
          n1683 = Or(x=w1606, y=w1605) -> (x .or. y?=w1596:bool)
          n1684 = Or(x=w1605, y=w1604) -> (x .or. y?=w1595:bool)
          n1685 = Or(x=w1602, y=w1603) -> (x .or. y?=w1598:bool)
          n1686 = Or(x=w1603, y=w1601) -> (x .or. y?=w1597:bool)
          n1687 = Or(x=w1611, y=w1612) -> (x .or. y?=w1600:bool)
          n1688 = Or(x=w1665, y=w1664) -> (x .or. y?=w1599:bool)
          n1689 = case shown="False" w1685 {
            tunnel: w1682 -> [w1707 w1715]
            tunnel: w1684 -> [_ w1712]
            tunnel: w1683 -> [_ w1711]
            tunnel: w1586 -> [_ w1710]
            tunnel: w1662 -> [_ w1709]
            tunnel: [w1707 w1714] -> w1681
            tunnel: [w1706 w1713] -> w1680
            tunnel: w1594 -> [w1706 w1708]
            frame False {
            }
            frame True {
              n1690 = call "myRIO_BRig_RT__Case_Exp__recordLick.vi"("intput_state__trialEnd"=w1709, "intput_state__trialStart"=w1710, "input_lick__R"=w1711, "input_lick__L"=w1712, "input_dataCurrent"=w1708, "input_dataLick"=w1715) -> ("output_dataCurrent"=w1713:u16[], "output_dataLick"=w1714:u16[][])  [unwired: 4 in]
            }
          }
          n1691 = Or(x=w1666, y=w1652) -> (x .or. y?=w1642:bool)
          n1692 = Or(x=w1651, y=w1667) -> (x .or. y?=w1663:bool)
          n1693 = Or(x=w1686, y="STOP_abort") -> (x .or. y?=w1688:bool)
          n1694 = Select(t=w1632, s=w1633, f=w1631) -> (s? t:f=w1622:u16)
          n1695 = Select(t=w1593, s=w1635, f=w1634) -> (s? t:f=w1621:u16)
          n1696 = Select(t=u16 0, s=w1638, f=w1637) -> (s? t:f=w1624:u16)
          n1697 = xnode "Read/Write Control"("FPGA VI Reference In"=w1644, "error in"=w1643, "audioTrigger_L"=w1642, "audioTrigger_R"=w1663, "CueLed_Event"=w1610, "A3_SL"=w1600, "A1_SR"=w1599, "LC_Event_l1"=w1598, "LC_Laser_l1"=w1597, "LC_Event_l2"=w1596, "LC_Laser_l2"=w1595) -> ("FPGA VI Reference Out"=w1679:refnum<k20>, "error out"=w1678:errorcluster, "AnaIn_0"=w1615:u16, "AnaIn_1"=w1623:u16)
          n1698 = call "myRIO_BRig_RT_dataAnalog_enterData__PortA.vi"("input_iState"=w1586, "input_AI0"=w1615, "input_iEvent"=w1624, "input_AI1"=w1623, "input_iTrial"=w1622, "input_iBlock"=w1621, "input_index"=w1625, "input_dataAnalog"=w1641) -> ("output_dataAnalog"=w1640:u16[][])  [unwired: 3 in]
          n1699 = call "myRIO_BRig_RT_TCP__v3__PortA.vi"("input_hTCP"=w1629, "input_AI1"=w1623, "input_AI0"=w1615, "input_I_connected_TCP"=w1626, "input_iBlock"=w1621, "input_spout"=w1620, "input_iTrial"=w1622, "input_error"=w1627, "input_countTrial"=w1617, "input_iState"=w1586) -> ("output_hTCP"=w1628:refnum<k5>, "output_countTrial"=w1616:u16, "output_error"=w1590:errorcluster)  [unwired: 3 in]
          n1700 = call "test_myRIO_Exp_tLoop.vi"("input_error"=w1590, "input_Threshold"=w1587, "input_timestamp"=w1588, "input_state"=w1586) -> ("output_Threshold"=w1584:bool, "output_duration"=→"tLoop":dbl, "error out"=w1589:errorcluster)  [unwired: 5 in]
          "Threshold" <- w1584
          n1701 = node-c288() -> ()  [unwired: 1 in, 1 out]
          n1702 = Increment(x=w1624) -> (x+1=w1630:u16)
          n1703 = Increment(x=w1625) -> (x+1=w1639:i32)
          "cState" <- w1586
        }
        n1704 = node-c288(w1527) -> ()  [unwired: 1 out]
        n1705 = flat-sequence {
          tunnel: w1523 -> [w1572]
          tunnel: w1522 -> [w1571]
          tunnel: [w1570] -> w1515
          tunnel: [w1569] -> w1514
          tunnel: [w1575] -> w1516
          tunnel: [w1576] -> w1521
          tunnel: w1515 -> [w1576]
          tunnel: w1514 -> [w1575]
          frame #0 {
            w1566 = u8 0
            w1567 = u16 0 ("AudioLeft_phase_inc")
            w1568 = FALSE
            n1706 = xnode "Read/Write Control"("FPGA VI Reference In"=w1572, "error in"=w1571, "Counts_Reset"=TRUE, "audioTrigger_L"=w1568, "audioFreq_L_kHz"=w1566, "audioAmp_L"=w1567, "audioTrigger_R"=w1568, "audioFreq_R_kHz"=w1566, "audioAmp_R"=w1567, "A3_SL"=w1568, "A1_SR"=w1568, "A6_Act"=w1568) -> ("FPGA VI Reference Out"=w1570:refnum<k20>, "error out"=w1569:errorcluster)
          }
          frame #1 {
            w1574 = FALSE ("START")
            n1707 = local write "START"(w1574) -> ()
            n1708 = local write "STOP_endTrial"(w1574) -> ()
            n1709 = local write "STOP_endBlock"(w1574) -> ()
          }
        }
        n1710 = stacked-sequence {
          tunnel: w1500 -> [w1546 _]
          tunnel: w1498 -> [w1547 _]
          tunnel: w1497 -> [_ w1552]
          tunnel: w1496 -> [_ w1551]
          tunnel: w1495 -> [_ w1550]
          tunnel: w1494 -> [w1540 _]
          tunnel: w1476 -> [w1537 _]
          tunnel: w1475 -> [w1536 _]
          frame #0 {
            n1711 = call "myRIO_BRig_RT_dataCurrent_idxDataLick.vi"() -> ("output_idxDataLick"=w1541:i32)  [unwired: 11 in]
            n1712 = Index Array(array=w1540, index=w1541) -> (element=w1543:u16)
            n1713 = Array Subset(array=w1537, length (row)=w1536) -> (w1538:u16[][])  [unwired: 3 in]
            n1714 = Increment(x=w1543) -> (x+1=w1544:u16)
            n1715 = call "myRIO_BRig_RT_comm_webdav_saveArrayToFile__1D_u16.vi"("Array"=w1547, "input_filename"="dataMTrig") -> ()  [unwired: 10 in]
            n1716 = To Long Integer(number=w1544) -> (32bit integer=w1542:i32)
            n1717 = Array Subset(array=w1546, length (row)=w1542) -> (w1545:u16[][])  [unwired: 3 in]
            n1718 = call "myRIO_BRig_RT_comm_webdav_saveArrayToFile__2D_u16.vi"("Array"=w1545, "input_filename"="dataLick") -> ()  [unwired: 10 in]
            n1719 = call "myRIO_BRig_RT_comm_webdav_saveArrayToFile__2D_u16.vi"("Array"=w1538, "input_filename"="dataAnalog") -> ()  [unwired: 10 in]
          }
          frame #1 {
            n1720 = case shown="True" w1552 {
              tunnel: w1551 -> [_ w1554]
              tunnel: w1550 -> [_ w1553]
              frame False {
              }
              frame True {
                n1721 = stacked-sequence {
                  tunnel: w1554 -> [w1556 w1563 w1565]
                  tunnel: w1553 -> [w1557 w1562 _]
                  frame #0 {
                    n1722 = call "myRIO_BRig_RT_comm_webdav_uploadFile__announce.vi"("input_addText"=TRUE, "input_fileName_prefix"=w1557, "intput_fileName"="curExp_end", "intput_hSession"=w1556) -> ("output_Isuccess"=w1555:bool)  [unwired: 6 in, 1 out]
                    n1723 = case shown="True" w1555 {
                      frame False {
                        n1724 = One Button Dialog(message="!!! Warning !!! Your data is located at C:\\BehaviorRig\\commTransfer") -> ()  [unwired: 1 in, 1 out]
                      }
                      frame True {
                        n1725 = Wait (ms)(milliseconds to wait=u32 20) -> ()  [unwired: 1 out]
                      }
                    }
                  }
                  frame #1 {
                    n1726 = call "myRIO_BRig_RT__endExp_sendData.vi"("input_fileName_prefix"=w1562, "input_hSession"=w1563) -> ()  [unwired: 8 in, 2 out]
                  }
                  frame #2 {
                    n1727 = local write "Connected To Host?"(FALSE ("Connected To Host?")) -> ()
                    n1728 = call <vilib>:"Close Session.vi"("session handle"=w1565) -> ()  [unwired: 14 in, 1 out]
                  }
                }
              }
            }
          }
        }
      }
    }
    n1729 = local read "STOP_abort"() -> (w44:bool)
  }
  n1730 = case shown="True" w5 {
    tunnel: w4 -> [_ w3613]
    tunnel: w3 -> [_ w3612]
    frame False {
    }
    frame True {
      n1731 = call "myRIO__TCP_disconnect_forWrite.vi"("input_error"=w3612, "input_hTCP"=w3613) -> ()  [unwired: 9 in, 1 out]
    }
  }
  n1732 = xnode "Read/Write Control"("FPGA VI Reference In"=w16, "error in"=w15, "FPGA_Stop"=TRUE) -> ("FPGA VI Reference Out"=w21:refnum<k20>, "error out"=w22:errorcluster)
  n1733 = xnode "Close FPGA VI Reference"("FPGA VI Reference In"=w21, "error in"=w22) -> ("error out"=w20:errorcluster)
  n1734 = call <vilib>:"Reset myRIO.vi"("error in (no error)"=w20) -> ()  [unwired: 10 in, 1 out]
